vi "DM2000.vi"   [LabVIEW 2013, in "main.lvlib"]
uses:
  main.lvlib
  Controls/Enum Variables.ctl
  Controls/Enum Save Action Events.ctl
  Controls/Enum Paper Action Events.ctl
  Controls/Enum Process Data.ctl
  Controls/Enum DICOM.ctl
  Controls/Enum User Events.ctl
  New Design/Controls/Reference AE Control.ctl
  Controls/SaveDataCluster.ctl
  Controls/Combobox Filename.ctl
  <vilib>/Utility/error.llb/DialogTypeEnum.ctl
  Components/TypeDef - SHIFTER.ctl
  New Design/Menu/Top Menu.vi
  New Design/Profile/Profile.vi
  New Design/Configuration/Configuration.vi
  New Design/Configuration/Configuration_table.vi
  New Design/Acquisition/Acquisition.vi
  New Design/Data/Data.vi
  New Design/Journal/Journal.vi
  <userlib>/_MGI/Error Handling/MGI Suppress Error Code/MGI Suppress Error Code (Scalar).vi
  Acquisition/RefData(SubVI).vi
  Bluetooth/AsyncBluetoothHandler.vi
  Globals/DataPathGlobalVariable.vi
  <userlib>/_OpenG.lib/file/file.llb/File Exists - Scalar__ogtk.vi
  Globals/DataAcqRecordPathGlobal.vi
  <vilib>/Utility/file.llb/Write To Spreadsheet File (string).vi
  <userlib>/_OpenG.lib/error/error.llb/Filter Error Codes (Array)__ogtk.vi
  <vilib>/Utility/file.llb/Read From Spreadsheet File (DBL).vi
  <vilib>/Utility/file.llb/Write To Spreadsheet File (DBL).vi
  <vilib>/Utility/file.llb/Read From Spreadsheet File (string).vi
  <userlib>/_OpenG.lib/file/file.llb/Valid Path - Traditional__ogtk.vi
  <vilib>/regexp/Match Regular Expression.xnode
  Components/Dependencies.llb/TLB_Dependencies.lvlib
  Settings/Options/Options.vi
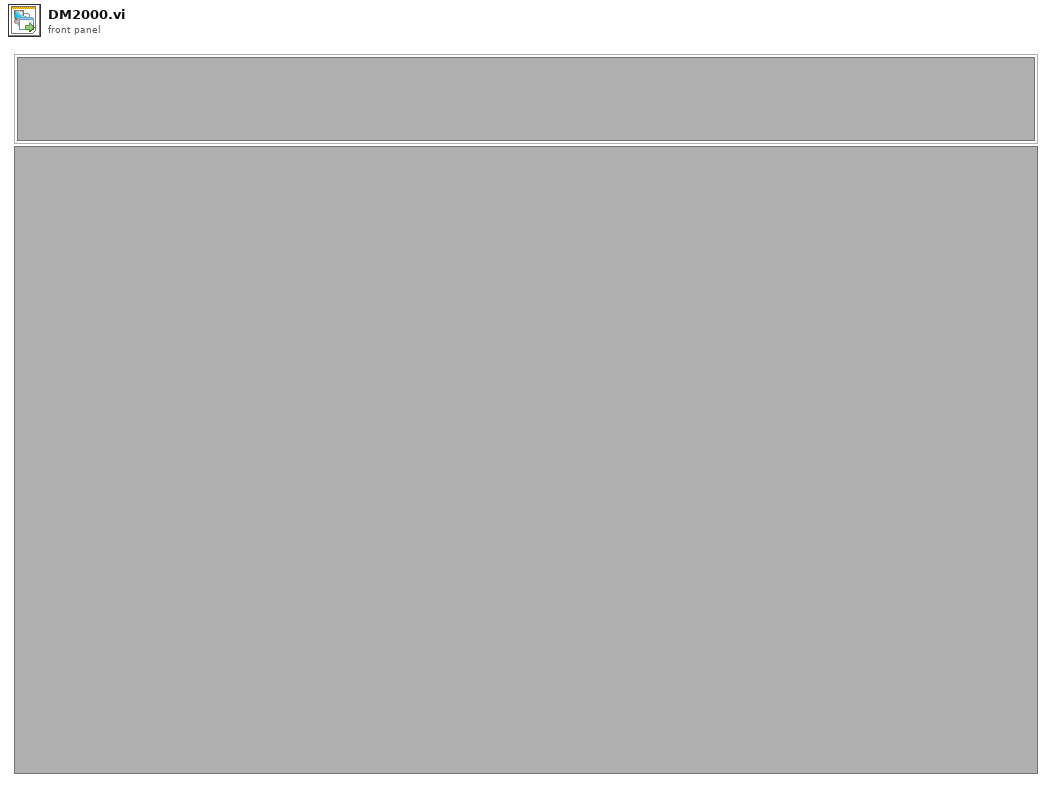
[diagram p1: front panel]
types:
  T1 = enum16{"Clear SR", "Set Display", "Set Shifter", "Initialize Events", "Init Q"}
  T2 = enum32{"Invalid", "Standard", "Closed", "Hidden", "Minimized", "Maximized"}
  T3 = typedef "main.lvlib/TypeDef - SHIFTER.ctl" = cluster{"Exit Event":T4, "Terminate Error":errorcluster, "User Parameter Controls":refnum<vi>[], "User Parameters":cluster{"Name":string, "CPR Number":string, "Measuring Type ":string, "Measuring Technique":string, "Measuring Limb":string, "Operator":string, "Doctor":string, "Comment":string, "AdditionalInfo":string, "RightArm":string[][], "LeftArm":string[][], "PalpationRight":string, "PalpationLeft":string, "Puls":dbl, "Temp One":dbl, "Temp Two":dbl, "ActivityBox":bool}, "System Parameters":cluster{"Paper Running?":bool, "GraphSelection":bool, "Date":string, "Active Page":string}, "Data Acquisition":cluster{"Acquisition":bool, "DAQmx Task":refnum<k21>, "DAQmx Error":errorcluster, "Record number":dbl, "RecordPath":path, "AcqDataRef":refnum<vi>, "Duration":timestamp, "Queue":refnum<queue>, "Control?":bool, "RelativeRecordPath":path}, "Reference signal":cluster{"DAQmx  Task ":refnum<k21>, "Monitor":bool, "Events":dbl, "Time":timestamp, "NullEvents":dbl, "RefDataRef":refnum<vi>, "Queue":refnum<queue>}, "Data Process":cluster{"SubpanelRef":refnum<vi>, "ActiveItemTag":string, "Queue":refnum<queue>}, "System Parameter Controls":refnum<vi>[], "Database":cluster{"PatientdataRef":refnum<file>, "PatientdataPath":path, "Blue Pressure":dbl, "Red Pressure":dbl, "ActiveItemTag":string, "Height Adjustment":dbl, "BluePositionArray":dbl[][], "RedPositionArray":dbl[][], "JournalPath":path}, "MWL":cluster{"PatientID":string, "Name":string, "DICOM Info":path, "DICOM Variables":string[], "Worklist":string[][]}, "Control":cluster{"Queue":refnum<queue>, "SignalCluster":cluster{"Pump":bool, "Finger":bool, "Ankle":bool, "Fast Def":bool, "Slow Def":bool, "Init Cal":bool, "Table Pres":bool, "Table":bool}}, "PageMenu":cluster{"VI Reference":refnum<vi>, "Queue":refnum<queue>}, "Profile":cluster{"VI Reference":refnum<vi>, "Queue":refnum<queue>}, "Configuration":cluster{"VI Reference":refnum<vi>, "Queue":refnum<queue>}, "Acquisition":cluster{"VI Reference":refnum<vi>, "Queue":refnum<queue>}, "Data":cluster{"VI Reference":refnum<vi>, "Queue":refnum<queue>}, "Journal":cluster{"VI Reference":refnum<vi>, "Queue":refnum<queue>}, "cRef":T5, "Bluetooth":cluster{"Queue":refnum<queue>, "VI Reference":refnum<vi>}}
  T4 = typedef "main.lvlib/TLB_Dependencies.lvlib/Exit Event Ref.ctl" = refnum<user-event>
  T5 = typedef "main.lvlib/Reference Cluster.ctl" = cluster{"Menu":cluster{"References":cluster{"Stop Acq":refnum<vi>, "MenuExit":refnum<vi>, "MenuStartADC":refnum<vi>, "PersonalInfoString":refnum<vi>, "Profile":refnum<vi>, "Configuration":refnum<vi>, "Acquisition":refnum<vi>, "Data":refnum<vi>, "Journal":refnum<vi>}}, "Profile":cluster{"References":cluster{"Search Patient ID":refnum<vi>, "Name":refnum<vi>, "CommentStr":refnum<vi>, "Listbox Patient ID":refnum<vi>, "ListboxDoctor":refnum<vi>, "ListboxOperator":refnum<vi>, "HospitalName":refnum<vi>, "HospitalDepartment":refnum<vi>, "HospitalAddress":refnum<vi>, "EditHospInfo":refnum<vi>, "Add Patient ID Btn":refnum<vi>, "Query Worklist":refnum<vi>}}, "Configuration":cluster{"References":cluster{"ListboxMeasurementArea":refnum<vi>, "ListboxMeasurementTechnique":refnum<vi>, "ListboxMeasurementMeth":refnum<vi>, "ListboxRightSegmentNr":refnum<vi>, "ListboxLeftSegmentNr":refnum<vi>, "HeightAdjustmentInt":refnum<vi>, "PalpationRight":refnum<vi>, "PalpationLeft":refnum<vi>, "ActivityBox":refnum<vi>}, "New method":cluster{"AddNewMeasurementBtn":refnum<vi>, "Left Time Table":refnum<vi>, "Right Time Table":refnum<vi>}, "Old method":cluster{"LeftArmPressureTable":refnum<vi>, "RightArmPressureTable":refnum<vi>, "SaveArmPressureBtn":refnum<vi>, "Puls":refnum<vi>, "TempTwo":refnum<vi>, "TempOne":refnum<vi>}, "Method":string}, "Acquisition":cluster{"References":cluster{"SegmentAcqString":refnum<vi>, "RingActGraph":refnum<vi>}}, "Data":cluster{"References":cluster{"cmString":refnum<vi>, "AdjustedHeight":refnum<vi>, "Menu":refnum<vi>, "Tangent On/Off":refnum<vi>, "FilterControl":refnum<vi>}}, "Journal":cluster{"References":cluster{"ReportSelection":refnum<vi>, "Data":refnum<vi>, "GenerateReport":refnum<vi>, "Menu":refnum<vi>, "Send To PACS":refnum<vi>}}}
  T6 = typedef "main.lvlib/TLB_Dependencies.lvlib/amc_Message Queue.ctl" = refnum<queue>
  T7 = typedef "main.lvlib/Enum Variables.ctl" = enum16{"SetAcqFilter", "GetAcqFilter", "Set Filter", "Get Filter", "Set Height", "Get Height", "Set Recorded Height", "Get Recorded Height", "Set Blue Pressure", "Get Blue Pressure", "Set Red Pressure", "Get Red Pressure", "Init", "Reset Pressure", "Set Red Cursors", "Get Red Cursors", "Set Blue Cursors", "Get Blue Cursors", "Set Language", "Get Language", "Set Active Graphs", "Get ActiveGraphs", "Set Method", "Get Method", "Set Encryption", "Get Encryption", "Set ExcelVersion", "Get ExcelVersion", "Set DICOM Avail", "Get DICOM Avail", "Set DICOM Encode", "Get DICOM Encode", "Set JournalExport", "Get JournalExport", "Set Sequence", "Get Sequence", "Set DAQ Connected", "Get DAQ Connected", "Set Current Graph", "Get Current Graph", "Set General Settings", "Get Hyphenation", "Set Arm Calc Method", "Get Arm Calc Method", "Set Dicom Tags", "Get Dicom Tags", "Set BT Serial", "Get BT Serial", "Set BT Accepted Serials", "Get BT Accepted Serials", "Get BT License", "Set BT License"}
  T8 = typedef "main.lvlib/Enum Save Action Events.ctl" = enum16{"LoadReportPath", "SaveReportPath", "Load Graph Path", "Save Graph Path", "LoadDataPath", "SaveDataPath", "Load Template Path", "Save Template Path", "Load PressureFactor", "Save PressureFactor", "Init", "Load Listbox", "Save Listbox", "LoadHospInfo", "SaveHospInfo", "Load DICOM Activation", "Save DICOM Activation", "LoadDICOMInfoWL", "SaveDICOMInfoWL", "LoadDICOMInfoPACS", "SaveDICOMInfoPACS", "Load ArmCalcMethod", "Save ArmCalcMethod", "LoadItemTags", "SaveItemTags", "LoadDICOMEncoding", "SaveDICOMEncoding", "LoadJournalType", "SaveJournalType", "LoadAcqFilterType", "SaveAcqFilterType", "Load Sequence", "Save Sequence", "Load Acquisition Mode", "Save Acquisition Mode", "Load General Settings", "Save General Settings", "Load Language", "Save Language", "Load Dicom Tags", "Save Dicom Tags", "Load BT Serial", "Save BT Serial", "Load BT License", "Save BT License"}
  T9 = typedef "LVPoint32TypeDef.ctl" = cluster{"Horizontal":i32, "Vertical":i32}
  T10 = typedef "LVRowAndColumnTypeDef.ctl" = cluster{"Row":i32, "Column":i32}
  T11 = typedef "eventvkey.ctl" = enum16{"ASCII", "Enter", "Return", "Shift", "Ctrl", "Alt", "Cmd", "Opt", "Caps", "NumLock", "Clear", "Break", "Up", "Down", "Left", "Right", "Insert", "Delete", "Home", "End", "PageUp", "PageDown", "Escape", "Help", "Pause", "ScrollLock", "F1", "F2", "F3", "F4", "F5", "F6", "F7", "F8", "F9", "F10", "F11", "F12", "F13", "F14", "F15", "F16", "F17", "F18", "F19", "F20", "F21", "F22", "F23", "F24", "Play", "VolumeUp", "VolumeDown", "Mute", "Two Byte Char"}
  T12 = typedef "main.lvlib/Enum Paper Action Events.ctl" = enum16{"Paper State", "Init"}
  T13 = typedef "main.lvlib/Enum Process Data.ctl" = enum16{"Init", "Set Cursor Mode", "Set Data Path", "Get All"}
  T14 = typedef "main.lvlib/Enum DICOM.ctl" = enum16{"Set DICOM itemTags", "Set Dicom Encoding", "Set DICOM Attributes"}
  T15 = typedef "main.lvlib/Reference AE Control.ctl" = enum16{"Initialize", "Set Menu", "Set Profile", "Set Configuration", "Set Configuration_old", "Set Configuration_new", "Set Configuration Method", "Set Acquisition", "Set Data", "Set Journal", "Get"}
  T16 = typedef "main.lvlib/Enum User Events.ctl" = enum16{"User Event", "Init"}
  T17 = cluster{"License":string, "Accepted Serials":string[]}
  T18 = typedef "main.lvlib/SaveDataCluster.ctl" = cluster{"HospInfo":cluster{"Name":string, "Address":string, "Department":string}, "Pressure":cluster{"Pressure":dbl}, "DataPath":cluster{"DataPath":path}, "ReportPath":cluster{"Path":path, "Name":string}, "DICOM Info WL":cluster{"port":i32, "AEtitle":string, "host":string, "remoteAE":string}, "DICOM Info PACS":cluster{"port":i32, "AEtitle":string, "host":string, "remoteAE":string}, "ArmCalcMethod":dbl, "itemTags":string[], "DicomEncoding":u16, "JournalType":u16, "General Settings":cluster{"Hyphenation":bool, "Language":u16, "CellStr1":string, "CellStr2":string}, "Dicom Tags":string[][], "BT Serial":cluster{"Serial Number":string, "Side":string, "Ignore?":bool}[], "BT License":cluster{"License":string, "Accepted Serials":string[]}}
  T19 = typedef "main.lvlib/Combobox Filename.ctl" = string
  T20 = enum16{"leave excel open after last close", "close only if opened by LabVIEW", "close excel after last close"}
  T21 = cluster{"sys":dbl, "dia":dbl, "puls":dbl, "date":string, "time":string, "code":string, "serial":string, "temp":dbl, "activity":string}
  T22 = cluster{"name":string, "department":string, "address":string}
  T23 = cluster{"id":string, "name":string, "operator":string, "doctor":string, "comment":string}
  T24 = typedef "DialogTypeEnum.ctl" = enum16{"no dialog", "OK message", "continue or stop message", "auto error handling dialog", "OK message + warnings", "continue/stop + warnings"}
  T25 = cluster{"port":i32, "AEtitle":string, "host":string, "remoteAE":string}
  T26 = cluster{"Search Patient ID":refnum<vi>, "Name":refnum<vi>, "CommentStr":refnum<vi>, "Listbox Patient ID":refnum<vi>, "ListboxDoctor":refnum<vi>, "ListboxOperator":refnum<vi>, "HospitalName":refnum<vi>, "HospitalDepartment":refnum<vi>, "HospitalAddress":refnum<vi>, "EditHospInfo":refnum<vi>, "Add Patient ID Btn":refnum<vi>, "Query Worklist":refnum<vi>}
  T27 = cluster{"Name":refnum<vi>, "ListboxOperator":refnum<vi>, "ListboxDoctor":refnum<vi>, "CommentStr":refnum<vi>, "Name":string, "Operator":string, "Doctor":string, "Comment":string}
  T28 = cluster{"Hospital Name 2":string, "Hospital Address 2":string, "Department 2":string}
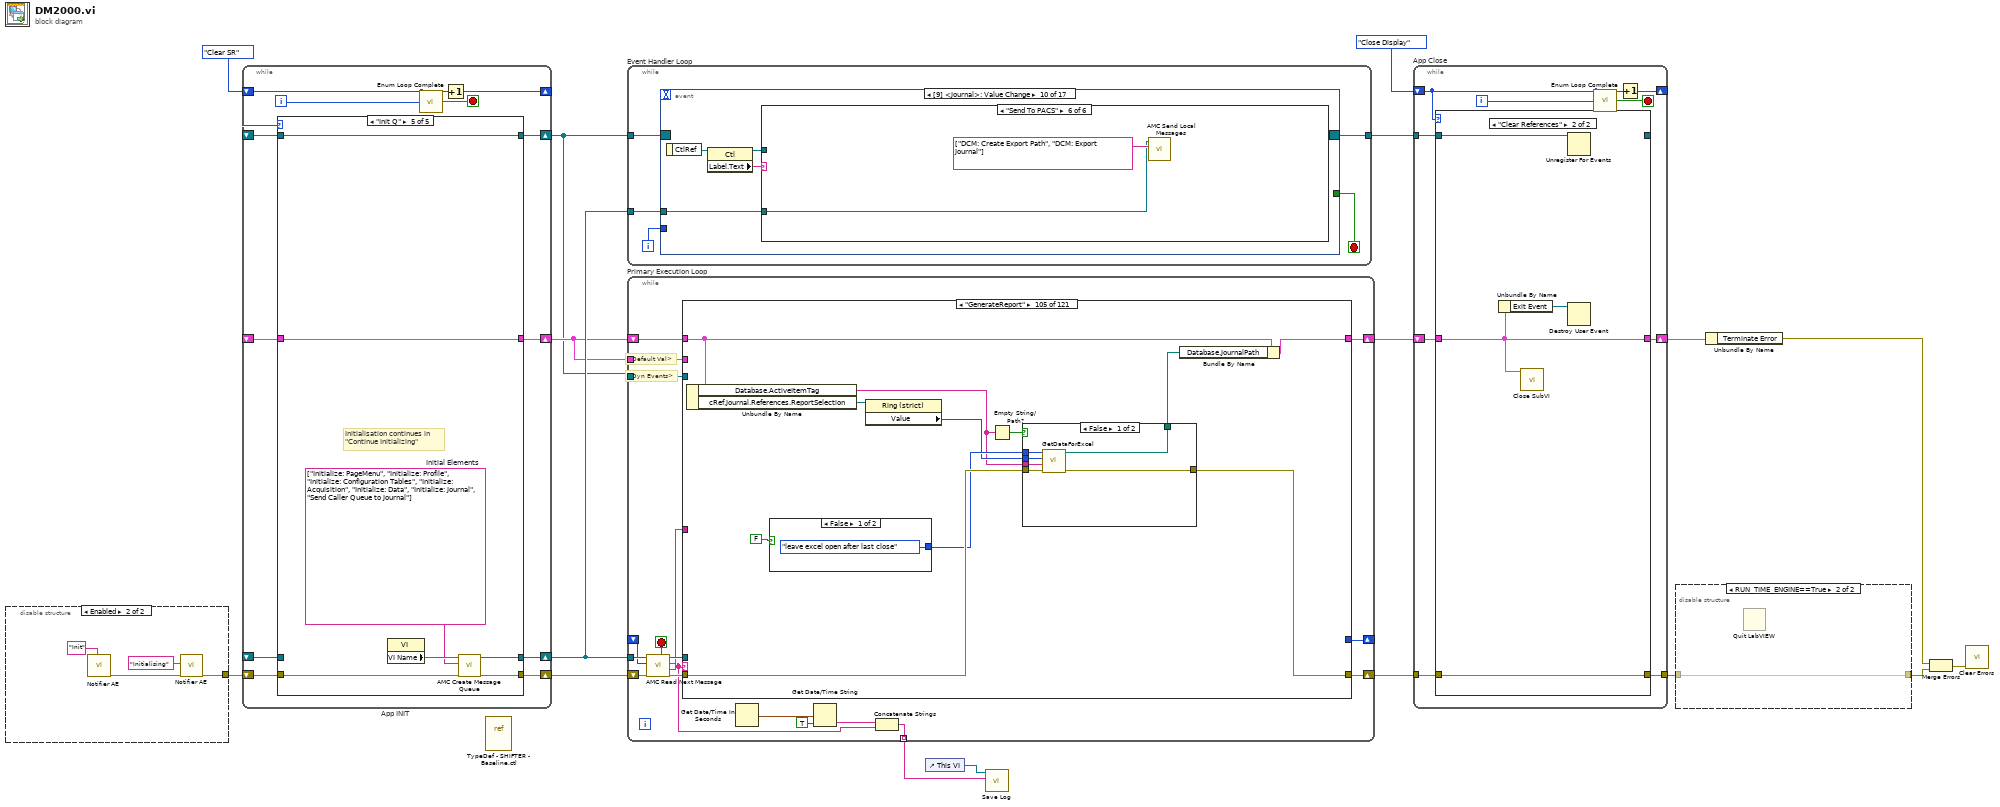
[diagram p0: block diagram]
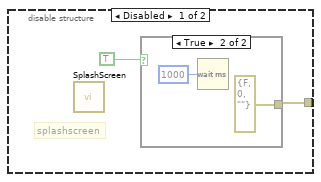
[diagram p2: hidden frame]
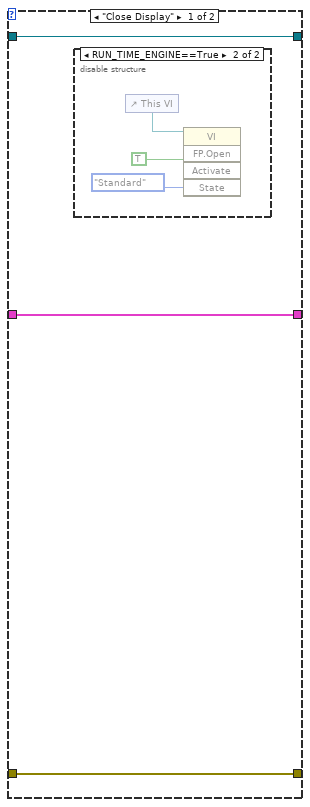
[diagram p5: hidden frame]
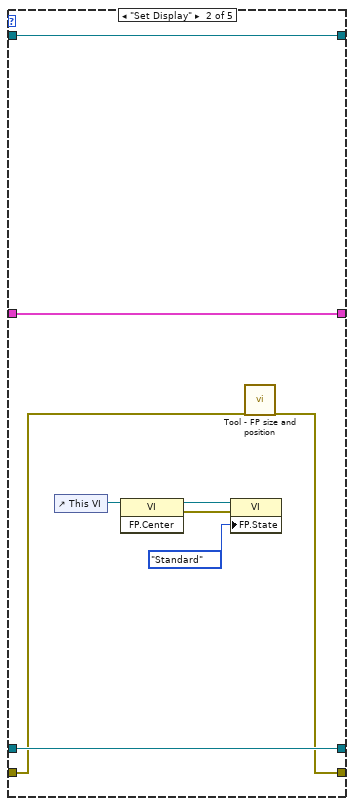
[diagram p8: hidden frame]
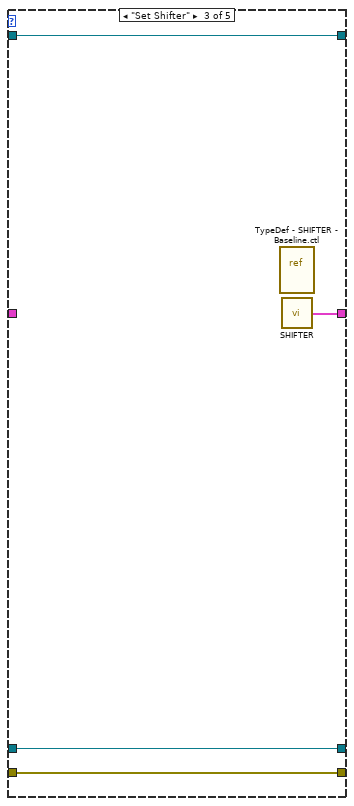
[diagram p9: hidden frame]
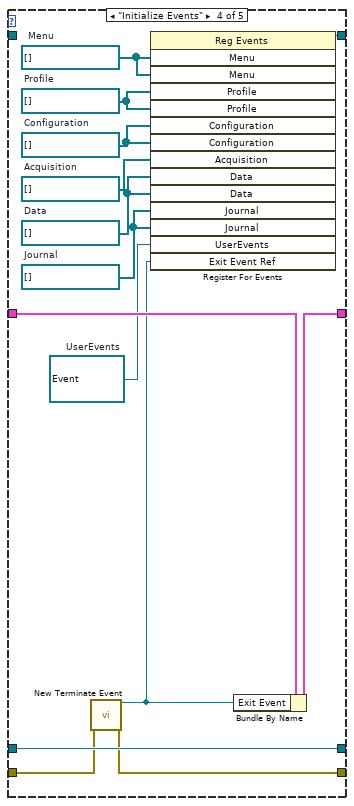
[diagram p10: hidden frame]
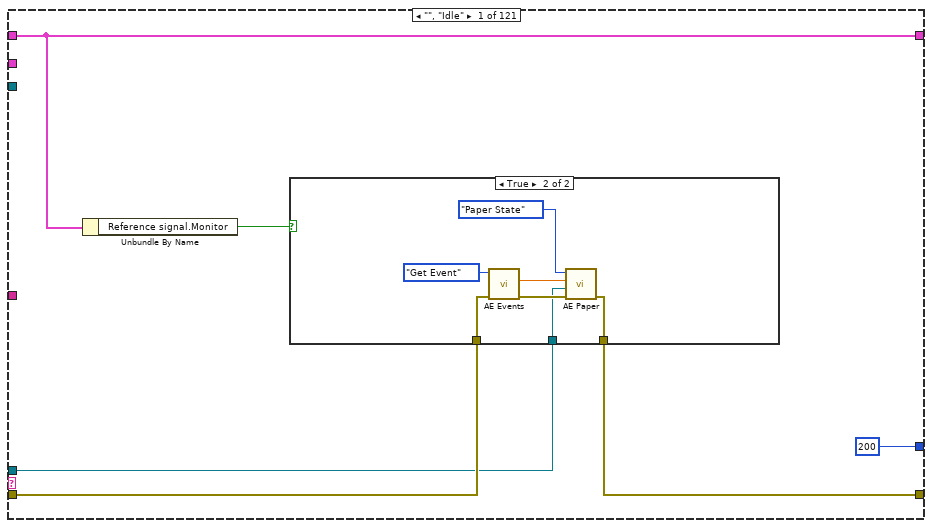
[diagram p11: hidden frame]
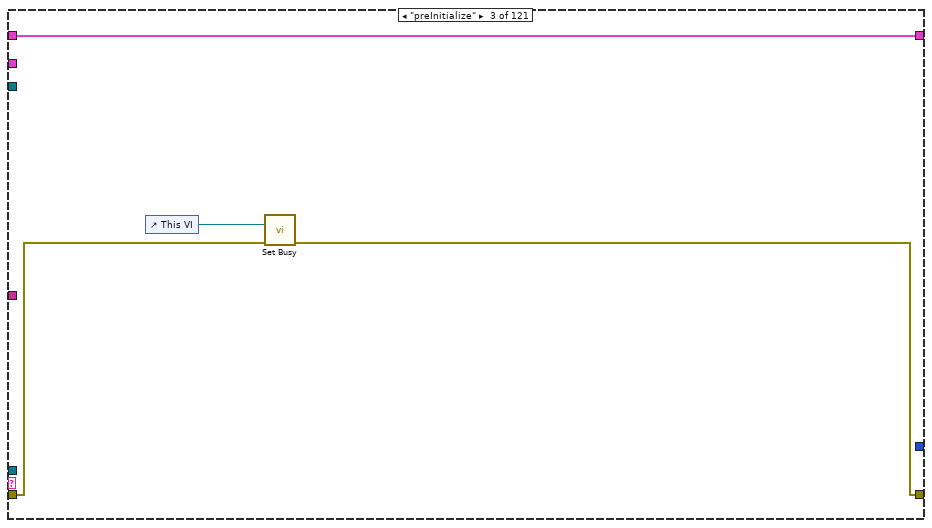
[diagram p14: hidden frame]
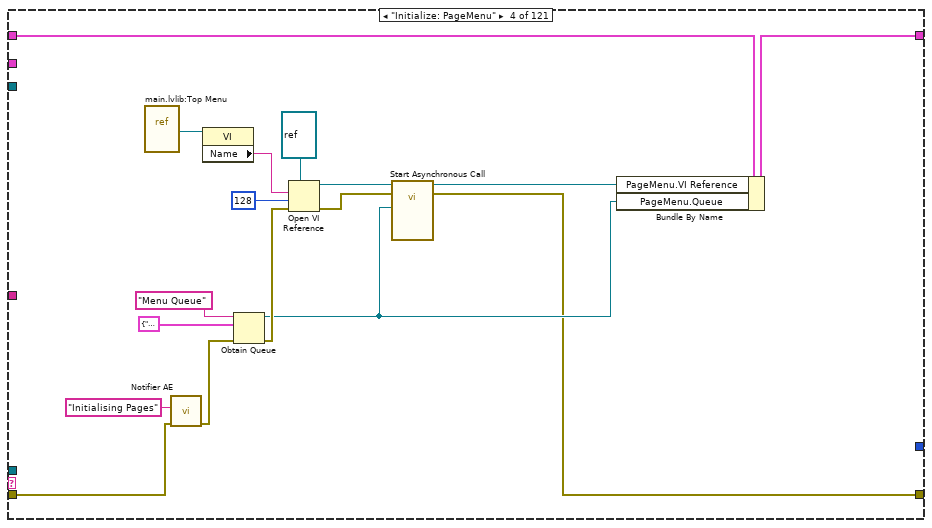
[diagram p15: hidden frame]
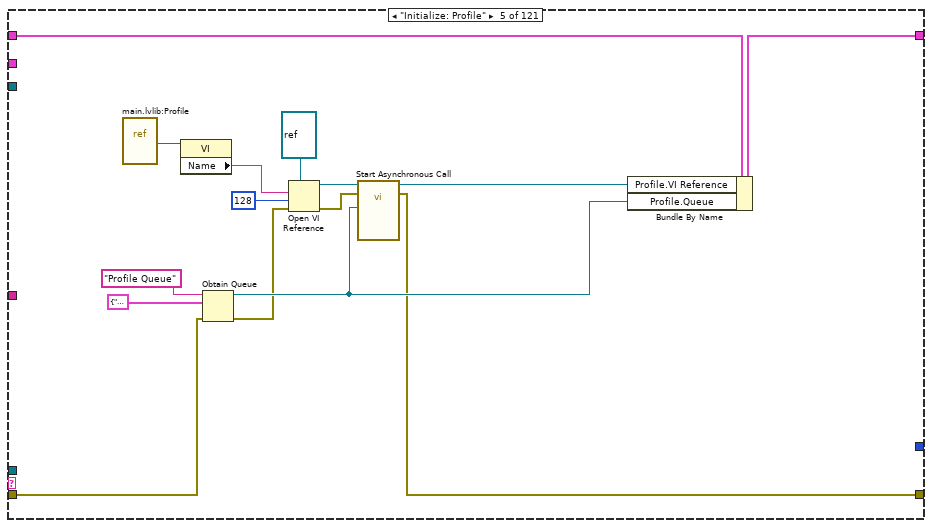
[diagram p16: hidden frame]
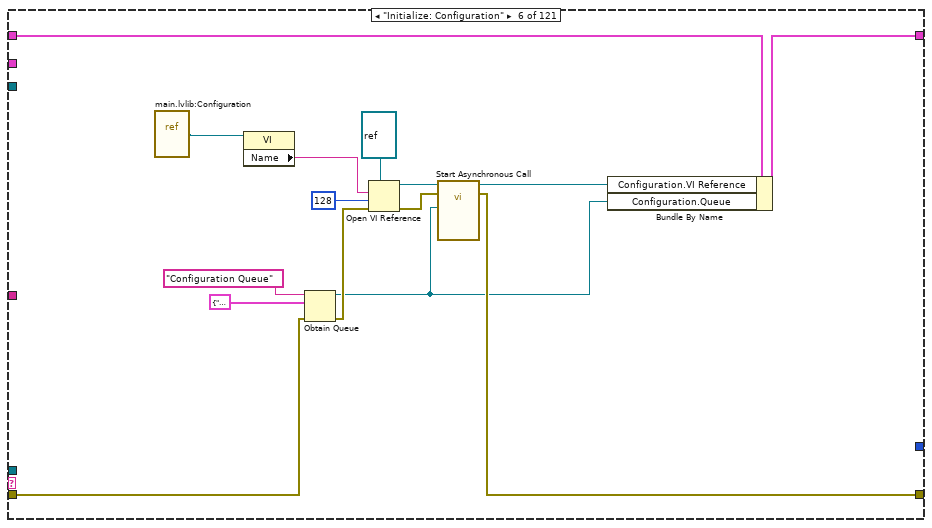
[diagram p17: hidden frame]
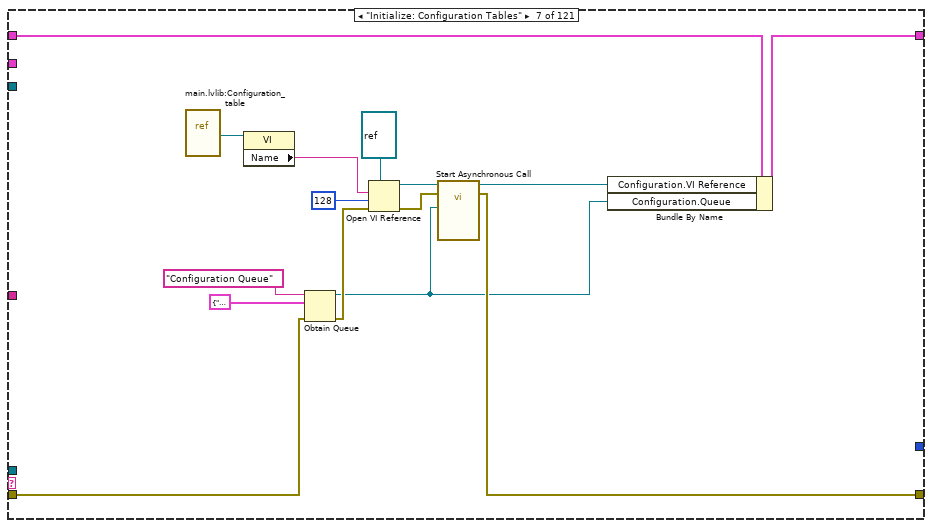
[diagram p18: hidden frame]
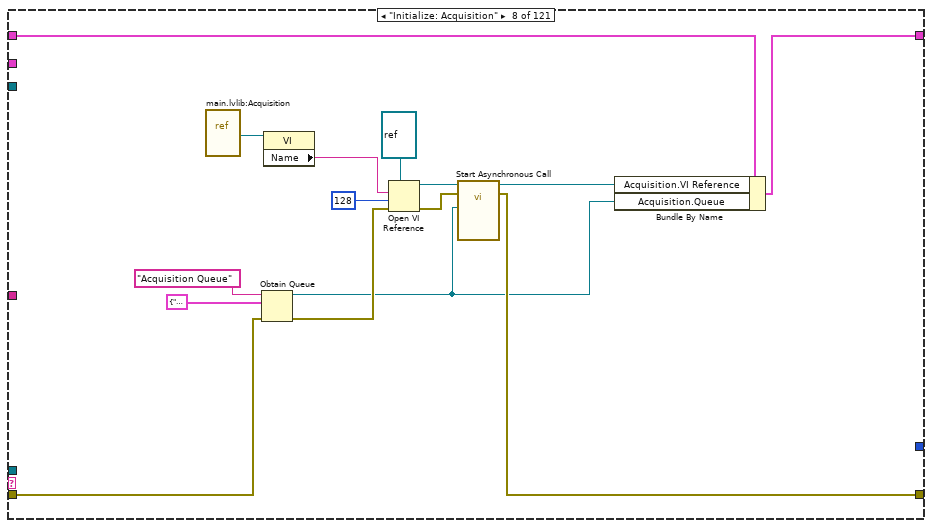
[diagram p19: hidden frame]
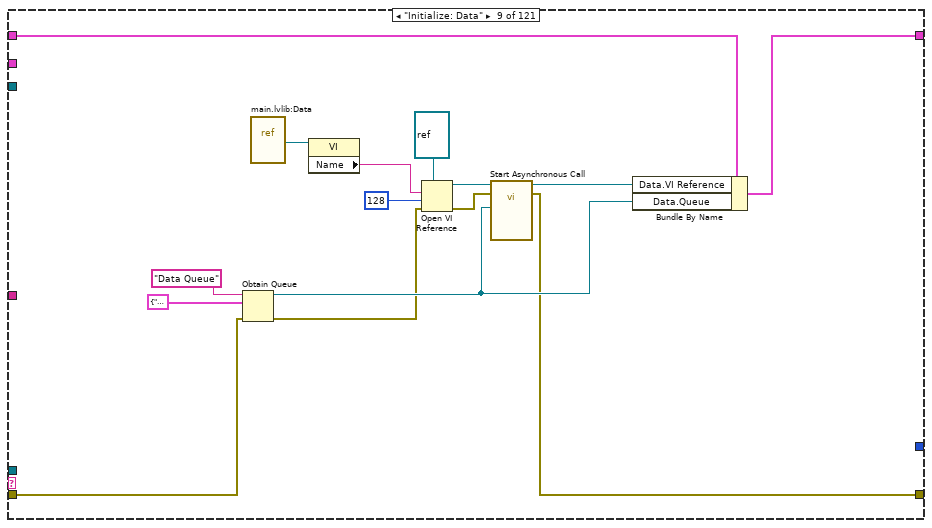
[diagram p20: hidden frame]
diagram:
  n1 = disable-structure shown="Enabled" {
    disable-tunnel: [w18 w23] -> w3
    frame Disabled {
      # "splashscreen"
      n2 = call "SplashScreen.vi"() -> ()  [unwired: 11 in, 1 out]
      n3 = case shown="True" TRUE {
        tunnel: [_ errorcluster {"status"=FALSE, "code"=0, "source"=""} ("error out")] -> w18
        frame False {
        }
        frame True {
          n4 = Wait (ms)(milliseconds to wait=u32 1000) -> ()  [unwired: 1 out]
        }
      }
    }
    frame Enabled {
      n5 = call "Notifier AE.vi"("Cmd"="Init") -> ("error out"=w24:errorcluster)  [unwired: 10 in]
      n6 = call "Notifier AE.vi"("error in (no error)"=w24, "String"="Initialising") -> ("error out"=w23:errorcluster)  [unwired: 9 in]
    }
  }
  n7 = while "App INIT" {
    shift-right: [w31] -> _
    shift-left: T1."Clear SR" -> [w26]
    shift-right: [w37] -> w7
    shift-left: _ -> [w30]
    shift-right: [w34] -> w12
    shift-left: w3 -> [w29]
    shift-right: [w36] -> w5
    shift-left: _ -> [w28]
    shift-right: [w35] -> w6
    shift-left: _ -> [w27]
    i -> [w32]
    stop <- w33 stop-if-true
    n8 = case shown="\"Init Q\"" w26 {
      tunnel: [_ w44 w49 w64 w68] -> w37
      tunnel: [_ w43 w48 w59 w66] -> w34
      tunnel: [_ w46 w50 w62 w70] -> w35
      tunnel: [_ w45 w47 w61 w71] -> w36
      tunnel: w30 -> [_ w44 w49 w64 _]
      tunnel: w29 -> [_ w42 w48 w60 w67]
      tunnel: w28 -> [_ w45 w47 _ w71]
      tunnel: w27 -> [_ w46 _ w63 w70]
      frame "Clear SR" {
      }
      frame "Set Display" {
        n9 = control-ref of="This VI"() -> (w40:refnum<vi>)
        n10 = invoke class="VI" method="FP.Center"(reference=w40) -> (reference out=w39:refnum<vi>, error out=w38:errorcluster)  [unwired: 2 in, 1 out]
        n11 = property class="VI"(reference=w39, error in=w38, "FP.State"=T2."Standard" ("Front Panel Window:State")) -> ()  [unwired: 2 out]
        n12 = call "Tool - FP size and position.vi"("error in (no error)"=w42) -> ("error out"=w43:errorcluster)  [unwired: 7 in, 11 out]
      }
      frame "Set Shifter" {
        n13 = vi-ref "TypeDef - SHIFTER - Baseline.ctl"() -> ()  [unwired: 1 out]
        n14 = call "SHIFTER.vi"() -> ("SHIFTER DATA"=w50:T3)  [unwired: 15 out]
      }
      frame "Initialize Events" {
        w53 = refnum<vi>[] []  # Journal
        w54 = refnum<vi>[] []  # Data
        w55 = refnum<vi>[] []  # Acquisition
        w56 = refnum<vi>[] []  # Configuration
        w52 = refnum<user-event> refnum  # UserEvents
        w57 = refnum<vi>[] []  # Profile
        w58 = refnum<vi>[] []  # Menu
        n15 = call "New Terminate Event.vi"("error in (no error)"=w60) -> ("Exit Event Ref"=w51:T4, "error out"=w59:errorcluster)  [unwired: 13 in]
        n16 = register-events(w58, w58, w57, w57, w56, w56, w55, w54, w54, w53, w53, w52, w51) -> (reference out=w61:refnum<event-registration>)  [unwired: 2 in, 1 out]
        n17 = Bundle By Name(cluster=w63, "Exit Event"=w51) -> (w62:T3)
      }
      frame "Init Q" {
        w65 = string[] ["Initialize: PageMenu", "Initialize: Profile", "Initialize: Configuration Tables", "Initialize: Acquisition", "Initialize: Data", "Initialize: Journal", "Send Caller Queue to Journal"]  # Initial Elements
        # "Initialisation continues in \n\"Continue Initializing\""
        n18 = property class="VI"() -> ("VI Name"=w69:string)  [unwired: 2 in, 2 out]
        n19 = call "AMC Create Message Queue.vi"("error in (no error)"=w67, "Initial Message Names"=w65, "Message Queue Name"=w69) -> ("error out"=w66:errorcluster, "Message Queue out"=w68:T6)  [unwired: 7 in]
      }
    }
    n20 = call "Enum Loop Complete.vi"("Current State Enum"=w26, "Itteration"=w32) -> ("Loop Complete?"=w33:bool)  [unwired: 13 out]
    n21 = Increment(x=w26) -> (x+1=w31:T1)
  }
  n22 = vi-ref "TypeDef - SHIFTER - Baseline.ctl"() -> ()  [unwired: 1 out]
  n23 = while "Event Handler Loop" {
    tunnel: w5 -> [w75]
    tunnel: w7 -> [w74]
    tunnel: [w73] -> w15
    i -> [w72]
    stop <- w76 stop-if-true
    n24 = event shown="[9] <Journal>: Value Change" {
      selector: w75 -> [_ _ _ _ _ _ _ _ _ _ _ _ _ _ _ _ _]
      dyn-events: [_ _ _ _ _ _ _ _ _ _ _ _ _ _ _ _ _] -> w73
      timeout: _ -> [_ _ _ _ _ _ _ _ _ _ _ _ _ _ _ _ _]
      tunnel: [_ _ _ _ _ _ _ _ _ _ _ _ TRUE ("NewVal") TRUE ("NewVal") _ w292 _] -> w76
      tunnel: w74 -> [w80 _ w106 w124 w155 _ _ w179 w191 w207 w219 w236 w269 w270 w274 w293 _]
      tunnel: w72 -> [_ _ _ _ _ _ _ _ _ _ _ _ _ _ _ _ _]
      event Value Change {
        n25 = event-data() -> ("CtlRef"=w82:refnum<vi>)  [unwired: 1 out]
        n26 = property class="Ctl"(reference=w82) -> (reference out=w77:refnum<vi>, "Label.Text"=w81:string)  [unwired: 1 in, 1 out]
        n27 = call "AMC Send Local Message.vi"("Message Name"="Cache User Parameters", "Message Queue in"=w80) -> ("Message Queue out"=w79:T6)  [unwired: 8 in, 1 out]
        n28 = case shown="\"Data\"" w81 {
          tunnel: w79 -> [_ w84 w85 w87 w89 w91 w97 w102 w105]
          tunnel: w77 -> [_ _ _ _ _ _ w96 _ _]
          frame "", Default {
          }
          frame "Profile" {
            n29 = call "AMC Send Local Messages.vi"("Message Names"=string[] ["Subpanel: Load Profile"], "Message Queue in"=w84) -> ()  [unwired: 8 in, 2 out]
          }
          frame "Configuration" {
            n30 = call "AMC Send Local Messages.vi"("Message Names"=string[] ["Subpanel: Load Configuration"], "Message Queue in"=w85) -> ()  [unwired: 8 in, 2 out]
          }
          frame "Acquisition" {
            n31 = call "AMC Send Local Messages.vi"("Message Names"=string[] ["Update Display", "Subpanel: Load Acquisition", "Send Segment to Acquisition"], "Message Queue in"=w87) -> ()  [unwired: 8 in, 2 out]
          }
          frame "Data" {
            n32 = call "AMC Send Local Messages.vi"("Message Names"=string[] ["Subpanel: Load Data"], "Message Queue in"=w89) -> ()  [unwired: 8 in, 2 out]
          }
          frame "Journal" {
            n33 = call "AMC Send Local Messages.vi"("Message Names"=string[] ["Subpanel: Load Journal", "FillDataTable"], "Message Queue in"=w91) -> ()  [unwired: 8 in, 2 out]
          }
          frame "MenuStartADC" {
            n34 = property class="Ctl"(reference=w96) -> ("Value"=w95:variant)  [unwired: 1 in, 2 out]
            n35 = Variant To Data(type=TRUE, Variant=w95) -> (data=w93:bool)  [unwired: 1 in, 1 out]
            n36 = case shown="True" w93 {
              tunnel: w97 -> [w98 w100]
              frame False {
                n37 = call "AMC Send Local Messages.vi"("Message Names"=string[] ["Stop Reference", "Update Display", "", "", ""], "Message Queue in"=w98) -> ()  [unwired: 8 in, 2 out]
              }
              frame True {
                n38 = call "AMC Send Local Messages.vi"("Message Names"=string[] ["Query DAQ Availability", "SavePatientDataOnDate"], "Message Queue in"=w100) -> ()  [unwired: 8 in, 2 out]
              }
            }
          }
          frame "Stop Acq" {
            n39 = call "AMC Send Local Messages.vi"("Message Names"=string[] ["Stop Reference", "Update Display", "", "", ""], "Message Queue in"=w102) -> ()  [unwired: 8 in, 2 out]
          }
          frame "MenuExit" {
            n40 = call "AMC Send Local Message.vi"("Message Name"="Exit", "Message Queue in"=w105) -> ()  [unwired: 8 in, 2 out]
          }
        }
      }
      event Shortcut Menu Selection (User) {
        n41 = event-data() -> ()  [unwired: 6 out]
      }
      event Value Change {
        n42 = event-data() -> ("CtlRef"=w108:refnum<vi>)  [unwired: 1 out]
        n43 = property class="Ctl"(reference=w108) -> ("Label.Text"=w107:string)  [unwired: 1 in, 2 out]
        n44 = case shown="\"CommentStr\", \"ListboxDoctor\", \"ListboxOperator\", \"Name\"" w107 {
          tunnel: w106 -> [_ w109 w111 w114 w115 w117 w119]
          frame "", Default {
          }
          frame "Search Patient ID" {
            n45 = call "AMC Send Local Message.vi"("Message Name"="FindCprNumber", "Message Queue in"=w109) -> ()  [unwired: 8 in, 2 out]
          }
          frame "CommentStr", "ListboxDoctor", "ListboxOperator", "Name" {
            n46 = call "AMC Send Local Messages.vi"("Message Names"=string[] ["Cache User Parameters", "SavePatientData", "Update Display", "DCM: Update Variables"], "Message Queue in"=w111) -> ()  [unwired: 8 in, 2 out]
          }
          frame "Listbox Patient ID" {
            n47 = call "AMC Send Local Messages.vi"("Message Names"=string[] ["ResetToDefault", "LoadNameCpr", "Cache User Parameters", "SelectCpr", "DCM: Load DICOM Info", "DCM: Update Variables", "Load Armpressure"], "Message Queue in"=w114) -> ()  [unwired: 8 in, 2 out]
          }
          frame "EditHospInfo" {
            n48 = call "AMC Send Local Message.vi"("Message Name"="EditHospInfo", "Message Queue in"=w115) -> ()  [unwired: 8 in, 2 out]
          }
          frame "Add Patient ID Btn" {
            n49 = call "AMC Send Local Messages.vi"("Message Names"=string[] ["AddCpr", ""], "Message Queue in"=w117) -> ()  [unwired: 8 in, 2 out]
          }
          frame "Query Worklist" {
            n50 = call "AMC Send Local Messages.vi"("Message Names"=string[] ["MWL: QueryWorklist", "MWL: PatientID", "ResetToDefault", "LoadNameCpr", "Cache User Parameters", "MWL: Update Data", "SelectCpr"], "Message Queue in"=w119) -> ()  [unwired: 8 in, 2 out]
          }
        }
      }
      event Shortcut Menu Selection (User) {
        n51 = event-data() -> ("CtlRef"=w123:refnum<vi>, "ItemTag"=w122:string, "Coords"=w121:T9)  [unwired: 3 out]
        n52 = case shown="\"Add New\"" w122 {
          tunnel: w124 -> [_ w129 w145 w152]
          tunnel: w123 -> [_ w128 w144 w151]
          tunnel: w121 -> [_ w125 w141 _]
          frame "False", Default {
          }
          frame "DeleteID" {
            w127 = refnum<vi> refnum  # ListBox
            n53 = To More Specific Class(target class=w127, reference=w128) -> (specific class reference=w126:refnum<vi>)  [unwired: 1 in, 1 out]
            n54 = invoke class="LstBox" method="Point To Row"(reference=w126, "Point"=w125) -> (reference out=w133:refnum<vi>, "Row"=w131:i32)  [unwired: 5 in, 5 out]
            n55 = property class="LstBox"(reference=w133) -> ("Item Names"=w132:string[])  [unwired: 1 in, 2 out]
            n56 = Index Array(array=w132, index=w131) -> (element=w130:string)
            n57 = call "AMC Send Local Message.vi"("Message Value"=w130, "Message Name"="RemoveCpr", "Message Queue in"=w129) -> ()  [unwired: 7 in, 2 out]
          }
          frame "Delete" {
            w143 = refnum<vi> refnum  # ListBox
            n58 = To More Specific Class(target class=w143, reference=w144) -> (specific class reference=w142:refnum<vi>)  [unwired: 1 in, 1 out]
            n59 = invoke class="LstBox" method="Point To Row"(reference=w142, "Point"=w141) -> (reference out=w140:refnum<vi>, "Row"=w139:i32)  [unwired: 5 in, 5 out]
            n60 = property class="LstBox"(reference=w140) -> ("Label.Text"=w137:string)  [unwired: 1 in, 2 out]
            n61 = Number To Decimal String(number=w139) -> (decimal integer string=w135:string)  [unwired: 1 in]
            n62 = Concatenate Strings("Delete: ", w137) -> (w136:string)
            n63 = call "AMC Send Local Message.vi"("Message Value"=w135, "Message Name"=w136, "Message Queue in"=w145) -> ()  [unwired: 7 in, 2 out]
          }
          frame "Add New" {
            w150 = refnum<vi> refnum  # ListBox
            n64 = To More Specific Class(target class=w150, reference=w151) -> (specific class reference=w146:refnum<vi>)  [unwired: 1 in, 1 out]
            n65 = property class="LstBox"(reference=w146) -> ("Label.Text"=w148:string)  [unwired: 1 in, 2 out]
            n66 = Concatenate Strings("Add New: ", w148) -> (w147:string)
            n67 = call "AMC Send Local Message.vi"("Message Name"=w147, "Message Queue in"=w152) -> ()  [unwired: 8 in, 2 out]
          }
        }
      }
      event Value Change {
        n68 = event-data() -> ("CtlRef"=w158:refnum<vi>)  [unwired: 1 out]
        n69 = call "AMC Send Local Message.vi"("Message Name"="Cache User Parameters", "Message Queue in"=w155) -> ("Message Queue out"=w154:T6)  [unwired: 8 in, 1 out]
        n70 = property class="Ctl"(reference=w158) -> (reference out=w156:refnum<vi>, "Label.Text"=w157:string)  [unwired: 1 in, 1 out]
        n71 = case shown="\"HeightAdjustmentInt\"" w157 {
          tunnel: w154 -> [_ _ _ _ _ _ w165 _ _ _ _ _ w166 _ _]
          tunnel: w156 -> [_ _ _ w162 _ _ _ _ _ _ _ _ _ _ _]
          frame "False", Default {
          }
          frame "ListboxMeasurementArea" {
          }
          frame "ListboxMeasurementTechnique" {
          }
          frame "ListboxMeasurementMeth" {
            w161 = refnum<vi> refnum  # ListBox
            n72 = To More Specific Class(target class=w161, reference=w162) -> (specific class reference=w160:refnum<vi>)  [unwired: 1 in, 1 out]
            n73 = property class="LstBox"(reference=w160) -> ("Value"=w159:variant)  [unwired: 1 in, 2 out]
            n74 = call "AE Variables.vi"("VariantIn"=w159, "Action"=Enum_Variables."Set Method") -> ()  [unwired: 10 in, 8 out]
          }
          frame "ListboxRightSegmentNr" {
          }
          frame "ListboxLeftSegmentNr" {
          }
          frame "HeightAdjustmentInt" {
            n75 = call "AMC Send Local Message.vi"("Message Name"="Set Height", "Message Queue in"=w165) -> ()  [unwired: 8 in, 2 out]
          }
          frame "TempOne" {
          }
          frame "TempTwo" {
          }
          frame "Puls" {
          }
          frame "RightArmPressureTable" {
          }
          frame "LeftArmPressureTable" {
          }
          frame "SaveArmPressureBtn" {
            n76 = call "AMC Send Local Messages.vi"("Message Names"=string[] ["SaveArmPressure", "SavePalpationData"], "Message Queue in"=w166) -> ()  [unwired: 8 in, 2 out]
          }
          frame "PalpationRight" {
          }
          frame "PalpationLeft" {
          }
        }
      }
      event Shortcut Menu Selection (User) {
        n77 = event-data() -> ("ItemTag"=w168:string)  [unwired: 5 out]
        n78 = case shown="\"True\"" w168 {
          frame "False", Default {
          }
          frame "True" {
          }
        }
      }
      event Value Change {
        n79 = event-data() -> ("CtlRef"=w171:refnum<vi>)  [unwired: 1 out]
        n80 = property class="Ctl"(reference=w171) -> (reference out=w169:refnum<vi>, "Label.Text"=w170:string)  [unwired: 1 in, 1 out]
        n81 = case shown="\"RingActGraph\"" w170 {
          tunnel: w169 -> [_ w176]
          frame "", Default {
          }
          frame "RingActGraph" {
            w175 = refnum<vi> refnum  # Ring
            n82 = To More Specific Class(target class=w175, reference=w176) -> (specific class reference=w174:refnum<vi>, error out=w173:errorcluster)  [unwired: 1 in]
            n83 = property class="Ring"(reference=w174, error in=w173) -> ("Value"=w172:variant)  [unwired: 2 out]
            n84 = call "AE Variables.vi"("VariantIn"=w172, "Action"=Enum_Variables."Set Active Graphs") -> ()  [unwired: 10 in, 8 out]
          }
        }
      }
      event Value Change {
        n85 = event-data() -> ("CtlRef"=w181:refnum<vi>)  [unwired: 1 out]
        n86 = property class="Ctl"(reference=w181) -> (reference out=w178:refnum<vi>, "Label.Text"=w180:string)  [unwired: 1 in, 1 out]
        n87 = case shown="\"ProcessDataTreeMenu\"" w180 {
          tunnel: w179 -> [_ w182 w187 w189]
          tunnel: w178 -> [_ w184 _ _]
          frame "", Default {
          }
          frame "ProcessDataTreeMenu" {
            n88 = call "Tree Menu to String.vi"("Control in"=w184) -> ("delimited string"=w183:string)  [unwired: 10 in]
            n89 = Build Array(w183) -> (w185:string[])
            n90 = call "AMC Send Local Messages.vi"("Message Values"=w185, "Message Names"=string[] ["GetActiveItemTag", "Display Data", "Update Display"], "Message Queue in"=w182) -> ()  [unwired: 7 in, 2 out]
          }
          frame "Tangent On/Off" {
            n91 = call "AMC Send Local Message.vi"("Message Name"="Set Tangent Mode", "Message Queue in"=w187) -> ()  [unwired: 8 in, 2 out]
          }
          frame "FilterControl" {
            n92 = call "AMC Send Local Messages.vi"("Message Names"=string[] ["FilterControl", "Display Data", ""], "Message Queue in"=w189) -> ()  [unwired: 8 in, 2 out]
          }
        }
      }
      event Shortcut Menu Selection (User) {
        n93 = event-data() -> ("CtlRef"=w192:refnum<vi>, "ItemTag"=w193:string)  [unwired: 4 out]
        n94 = case shown="\"ChangeSegment\"" w193 {
          tunnel: w192 -> [_ w196 w200 w204]
          tunnel: w191 -> [_ w194 w198 w202]
          frame "", Default {
          }
          frame "DeleteTreeItem" {
            n95 = call "Tree Menu to String.vi"("Control in"=w196) -> ("delimited string"=w195:string)  [unwired: 10 in]
            n96 = call "AMC Send Local Message.vi"("Message Value"=w195, "Message Name"="DeleteTreeItem", "Message Queue in"=w194) -> ()  [unwired: 7 in, 2 out]
          }
          frame "ChangeSegment" {
            n97 = call "Tree Menu to String.vi"("Control in"=w200) -> ("delimited string"=w199:string)  [unwired: 10 in]
            n98 = call "AMC Send Local Message.vi"("Message Value"=w199, "Message Name"="ChangeSegment", "Message Queue in"=w198) -> ()  [unwired: 7 in, 2 out]
          }
          frame "ExportGraphs" {
            n99 = call "Tree Menu to String.vi"("Control in"=w204) -> ("delimited string"=w203:string)  [unwired: 10 in]
            n100 = call "AMC Send Local Message.vi"("Message Value"=w203, "Message Name"="ExportGraphs", "Message Queue in"=w202) -> ()  [unwired: 7 in, 2 out]
          }
        }
      }
      event Value Change {
        n101 = event-data() -> ("CtlRef"=w209:refnum<vi>)  [unwired: 1 out]
        n102 = property class="Ctl"(reference=w209) -> (reference out=w206:refnum<vi>, "Label.Text"=w208:string)  [unwired: 1 in, 1 out]
        n103 = case shown="\"Send To PACS\"" w208 {
          tunnel: w207 -> [_ _ _ w210 w215 w217]
          tunnel: w206 -> [_ _ _ _ w214 _]
          frame "", Default {
          }
          frame "ReportSelection" {
          }
          frame "Data Listbox" {
          }
          frame "GenerateReport" {
            n104 = call "AMC Send Local Message.vi"("Message Name"="GenerateReport", "Message Queue in"=w210) -> ()  [unwired: 8 in, 2 out]
          }
          frame "Data Menu" {
            # "Need to convert to array because\nmultiple messages"
            n105 = call "Tree Menu to String.vi"("Control in"=w214) -> ("delimited string"=w213:string)  [unwired: 10 in]
            n106 = Build Array(w213) -> (w212:string[])
            n107 = call "AMC Send Local Messages.vi"("Message Values"=w212, "Message Names"=string[] ["FillDataTable", "DCM: Create Export Path", "DCM: Load DICOM Info", "DCM: Update Variables"], "Message Queue in"=w215) -> ()  [unwired: 7 in, 2 out]
          }
          frame "Send To PACS" {
            n108 = call "AMC Send Local Messages.vi"("Message Names"=string[] ["DCM: Create Export Path", "DCM: Export Journal"], "Message Queue in"=w217) -> ()  [unwired: 8 in, 2 out]
          }
        }
      }
      event Shortcut Menu Selection (User) {
        n109 = event-data() -> ("CtlRef"=w221:refnum<vi>, "ItemTag"=w222:string, "Coords"=w220:T9)  [unwired: 3 out]
        n110 = case shown="\"DeleteSingleMeasurement\"" w222 {
          tunnel: w221 -> [_ w224 w233]
          tunnel: w220 -> [_ _ w230]
          tunnel: w219 -> [_ w223 w228]
          frame "", Default {
          }
          frame "DeleteTreeItem" {
            n111 = call "Tree Menu to String.vi"("Control in"=w224) -> ("delimited string"=w225:string)  [unwired: 10 in]
            n112 = call "AMC Send Local Message.vi"("Message Value"=w225, "Message Name"="DeleteTreeItem", "Message Queue in"=w223) -> ()  [unwired: 7 in, 2 out]
          }
          frame "DeleteSingleMeasurement" {
            w232 = refnum<vi> refnum  # MulticolumnListbox
            n113 = To More Specific Class(target class=w232, reference=w233) -> (specific class reference=w231:refnum<vi>)  [unwired: 1 in, 1 out]
            n114 = invoke class="MCListbox" method="Point To Row Column"(reference=w231, "Point"=w230) -> ("CellPosition"=w234:T10)  [unwired: 5 in, 6 out]
            n115 = Flatten To String(anything=w234) -> (data string=w227:string)  [unwired: 3 in, 2 out]
            n116 = call "AMC Send Local Message.vi"("Message Value"=w227, "Message Name"="DeleteSingleMeasurement", "Message Queue in"=w228) -> ()  [unwired: 7 in, 2 out]
          }
        }
      }
      event User Event {
        n117 = event-data() -> ("Event"=w235:string)  [unwired: 1 out]
        n118 = case shown="\"BTelement\"" w235 {
          selector: w235 -> [_ _ _ _ _ _ _ _ _ w257 _ _ _ _]
          tunnel: w236 -> [_ w237 w243 w246 w247 w249 w251 w254 w256 w258 w260 w262 w264 w265]
          frame "", Default {
          }
          frame "DaqError" {
            n119 = One Button Dialog(message="Programmet kan ikke få kontakt til dit USB6008\ndataopsamlingskort. Undersøg venligst om dette er\ntilsluttet korrekt.", button name ("OK")="Luk") -> ()  [unwired: 1 out]
            n120 = call "AMC Send Local Messages.vi"("Message Names"=string[] ["Stop Reference", "Update Display"], "Message Queue in"=w237) -> ()  [unwired: 8 in, 2 out]
          }
          frame "tdmsError" {
            n121 = One Button Dialog(message="Data fejl", button name ("OK")="Luk") -> ()  [unwired: 1 out]
            n122 = call "AMC Send Local Messages.vi"("Message Names"=string[] ["Stop Reference", "Update Display"], "Message Queue in"=w243) -> ()  [unwired: 8 in, 2 out]
          }
          frame "SavePressure" {
            n123 = call "AMC Send Local Messages.vi"("Message Names"=string[] ["GetProcessData", "SaveProcessData"], "Message Queue in"=w246) -> ()  [unwired: 8 in, 2 out]
          }
          frame "TangentMode" {
            n124 = call "AMC Send Local Message.vi"("Message Name"="Set Tangent Mode: True", "Message Queue in"=w247) -> ()  [unwired: 8 in, 2 out]
          }
          frame "StopCalibration" {
            n125 = call "AMC Send Local Messages.vi"("Message Names"=string[] ["Calibrate Pressure: Step 3", "Monitor Reference"], "Message Queue in"=w249) -> ()  [unwired: 8 in, 2 out]
          }
          frame "Set Acquisition Mode" {
            n126 = call "AMC Send Local Messages.vi"("Message Names"=string[] ["Set Acquisition Mode"], "Message Queue in"=w251) -> ()  [unwired: 8 in, 2 out]
          }
          frame "Set DICOM Availability" {
            n127 = call "AMC Send Local Messages.vi"("Message Names"=string[] ["Load Menu", "Initialize: Dicom"], "Message Queue in"=w254) -> ()  [unwired: 8 in, 2 out]
          }
          frame "New Data Path" {
            n128 = call "AMC Send Local Messages.vi"("Message Names"=string[] ["ResetToDefault", "Load Patient Register"], "Message Queue in"=w256) -> ()  [unwired: 8 in, 2 out]
          }
          frame "Regulation Stopped" {
            n129 = call "AMC Send Local Message.vi"("Message Name"=w257, "Message Queue in"=w258) -> ()  [unwired: 8 in, 2 out]
          }
          frame "Set New Hospital Info" {
            n130 = call "AMC Send Local Message.vi"("Message Name"="Load Hospital Info", "Message Queue in"=w260) -> ()  [unwired: 8 in, 2 out]
          }
          frame "Change Language" {
            n131 = call "AMC Send Local Messages.vi"("Message Names"=string[] ["Change Language", "Load Patient Register", "Initialize: Dicom"], "Message Queue in"=w262) -> ()  [unwired: 8 in, 2 out]
          }
          frame "BTelement" {
            n132 = call "AMC Send Local Message.vi"("Message Name"="BT: Dequeue Element", "Message Queue in"=w264) -> ()  [unwired: 8 in, 2 out]
          }
          frame "SavePatientData" {
            n133 = call "AMC Send Local Message.vi"("Message Name"="SavePatientData", "Message Queue in"=w265) -> ()  [unwired: 8 in, 2 out]
          }
        }
      }
      event User Event {
        n134 = event-data() -> ()  [unwired: 2 out]
        n135 = call "AMC Send Local Messages.vi"("Message Names"=string[] ["BT: Stop", "Exit"], "Message Queue in"=w269) -> ()  [unwired: 8 in, 2 out]
      }
      event Panel Close? {
        w272 = TRUE  # Discard?
        n136 = event-data() -> ()  [unwired: 2 out]
        n137 = call "AMC Send Local Message.vi"("Message Name"="Exit", "Message Queue in"=w270) -> ()  [unwired: 8 in, 2 out]
        n138 = event-data("Discard?"=w272) -> ()  [unwired: 1 in, 1 out]
      }
      event Key Down {
        n139 = event-data() -> ("VKey"=w275:T11, "ScanCode"=w276:i16)  [unwired: 3 out]
        n140 = case shown="57" w276 {
          tunnel: w275 -> [_ _ w281 w286]
          tunnel: w274 -> [_ w278 w280 w285]
          frame 0, Default {
          }
          frame 57 {
            # "Space"
            n141 = call "AMC Send Local Message.vi"("Message Value"="Space", "Message Name"="KeyDown", "Message Queue in"=w278) -> ()  [unwired: 7 in, 2 out]
          }
          frame 77 {
            n142 = case shown="\"Right\"" w281 {
              tunnel: w280 -> [_ w283]
              frame "ASCII", Default {
              }
              frame "Right" {
                # "Rightarrow"
                n143 = call "AMC Send Local Message.vi"("Message Value"="Right", "Message Name"="KeyDown", "Message Queue in"=w283) -> ()  [unwired: 7 in, 2 out]
              }
            }
          }
          frame 75 {
            n144 = case shown="\"Left\"" w286 {
              tunnel: w285 -> [_ w288]
              frame "ASCII", Default {
              }
              frame "Left" {
                # "Leftarrow"
                n145 = call "AMC Send Local Message.vi"("Message Value"="Left", "Message Name"="KeyDown", "Message Queue in"=w288) -> ()  [unwired: 7 in, 2 out]
              }
            }
          }
        }
      }
      event Menu Selection (User) {
        n146 = event-data() -> ("MenuRef"=w290:refnum<k9>, "ItemTag"=w294:string, "ItemPath"=w291:string)  [unwired: 2 out]
        n147 = case shown="\"NewTest\"" w294 {
          tunnel: w293 -> [_ w295 w299 _ w301 _ w306 w312 _ _ w315 _ w318 w320 _ _ _ _ _ w330 _ _ _ _]
          tunnel: [_ _ TRUE _ _ _ _ _ _ _ _ _ _ _ _ _ _ _ _ _ _ _ _ _] -> w292
          tunnel: w291 -> [_ _ _ _ _ _ _ _ _ _ _ _ _ _ _ _ _ _ _ _ _ _ _ _]
          tunnel: w290 -> [_ _ _ _ _ _ _ _ _ _ _ _ _ _ _ _ _ _ _ _ _ _ _ _]
          frame Default {
          }
          frame "NewTest" {
            # "Opret ny undersøgelse"
            n148 = call "AMC Send Local Message.vi"("Message Name"="InitNewTest", "Message Queue in"=w295) -> ()  [unwired: 8 in, 2 out]
          }
          frame "ExitProgram" {
            n149 = call "AMC Send Local Messages.vi"("Message Names"=string[] ["Close SubVI", "Exit"], "Message Queue in"=w299) -> ()  [unwired: 8 in, 2 out]
          }
          frame "ArmPressureCalculation" {
            n150 = call "ArmPressureCalcMethod.vi"() -> ()  [unwired: 12 in]
          }
          frame "EditDataFolder" {
            n151 = call "SaveDataPath.vi"() -> ("Changed"=w300:bool)  [unwired: 11 in]
            n152 = case shown="True" w300 {
              tunnel: w301 -> [_ w302]
              frame False {
              }
              frame True {
                n153 = call "AMC Send Local Message.vi"("Message Name"="ResetToDefault", "Message Queue in"=w302) -> ()  [unwired: 8 in, 2 out]
              }
            }
          }
          frame "EditJournalFolder" {
            n154 = call "SaveReportPath.vi"() -> ()  [unwired: 12 in]
          }
          frame "StartCalibration" {
            # "Calibration is stopped as userEvent"
            n155 = call "AE Variables.vi"("Action"=Enum_Variables."Get DAQ Connected") -> ("BooleanOut"=w304:bool)  [unwired: 11 in, 7 out]
            n156 = case shown="True" w304 {
              tunnel: w306 -> [_ w309]
              frame False {
                n157 = One Button Dialog(message="Acquisition module must be active") -> ()  [unwired: 1 in, 1 out]
              }
              frame True {
                n158 = call "AMC Send Local Messages.vi"("Message Names"=string[] ["Idle Monitor Reference", "Calibrate Pressure: Step 1", "Calibrate Pressure: Step 2"], "Message Queue in"=w309) -> ()  [unwired: 8 in, 2 out]
                n159 = call "stopCalibrationPopUp.vi"() -> ()  [unwired: 12 in]
              }
            }
          }
          frame "MeasurementTest" {
            n160 = call "AE Variables.vi"("Action"=Enum_Variables."Get DAQ Connected") -> ("BooleanOut"=w310:bool)  [unwired: 11 in, 7 out]
            n161 = case shown="True" w310 {
              tunnel: w312 -> [_ w313]
              frame False {
              }
              frame True {
                n162 = call "AMC Send Local Messages.vi"("Message Names"=string[] ["Stop Monitor Reference", "AcqTest", "Monitor Reference"], "Message Queue in"=w313) -> ()  [unwired: 8 in, 2 out]
              }
            }
          }
          frame "LowpassFilter" {
            n163 = call "acqFilterSelection.vi"() -> ()  [unwired: 12 in]
          }
          frame "Options" {
            n164 = call-by-ref "?"() -> ()  [unwired: 14 in, 2 out]
          }
          frame "FlowCalc" {
            n165 = call "AMC Send Local Message.vi"("Message Name"="Flow: View Signals", "Message Queue in"=w315) -> ()  [unwired: 8 in, 2 out]
          }
          frame "DICOM Server" {
            n166 = call "DICOMServerSettings.vi"() -> ()  [unwired: 12 in]
          }
          frame "EditDicomValues" {
            n167 = call "AMC Send Local Messages.vi"("Message Names"=string[] ["DCM: Edit Values"], "Message Queue in"=w318) -> ()  [unwired: 8 in, 2 out]
          }
          frame "ShowDicomValues" {
            n168 = call "AMC Send Local Messages.vi"("Message Names"=string[] ["DCM: Show Values"], "Message Queue in"=w320) -> ()  [unwired: 8 in, 2 out]
          }
          frame "Journal" {
            w321 = u16 0 items=["Journal", "Graph"]
            n169 = call "AE Variables.vi"("VariantIn"=w321, "Action"=Enum_Variables."Set JournalExport") -> ()  [unwired: 10 in, 8 out]
            n170 = call "AE Save.vi"("Variant In"=w321, "Action"=Enum_Save_Action_Events."SaveJournalType") -> ()  [unwired: 7 in, 2 out]
          }
          frame "Graph" {
            w324 = u16 1 items=["Journal", "Graph"]
            n171 = call "AE Variables.vi"("VariantIn"=w324, "Action"=Enum_Variables."Set JournalExport") -> ()  [unwired: 10 in, 8 out]
            n172 = call "AE Save.vi"("Variant In"=w324, "Action"=Enum_Save_Action_Events."SaveJournalType") -> ()  [unwired: 7 in, 2 out]
          }
          frame "Bitmap" {
            w327 = u16 0 items=["Bitmap", "JPEG"] ("Encoding")
            n173 = call "DICOMFileEncoding.vi"("Encoding"=w327) -> ()  [unwired: 11 in]
          }
          frame "JPEG" {
            w328 = u16 1 items=["Bitmap", "JPEG"] ("Encoding")
            n174 = call "DICOMFileEncoding.vi"("Encoding"=w328) -> ()  [unwired: 11 in]
          }
          frame "ChangePassword" {
            n175 = call "change_password.vi"() -> ()  [unwired: 12 in]
          }
          frame "UpdateProgram" {
            n176 = call "AMC Send Local Message.vi"("Message Name"="Update Program", "Message Queue in"=w330) -> ()  [unwired: 8 in, 2 out]
          }
          frame "ActivateDICOM" {
            n177 = call "Activation.vi"() -> ()  [unwired: 12 in]
          }
          frame "Danish" {
            (unwired) u16 0 ("Value (Signaling)")
          }
          frame "English" {
            (unwired) u16 1 ("Value (Signaling)")
          }
          frame "French" {
            (unwired) u16 2 ("Value (Signaling)")
          }
        }
      }
      event Menu Activation? {
        n178 = event-data() -> ("MenuRef"=w331:refnum<k9>)  [unwired: 1 out]
        n179 = call "AE Variables.vi"("Action"=Enum_Variables."Get DICOM Avail") -> ("BooleanOut"=w332:bool)  [unwired: 11 in, 7 out]
        n180 = case shown="True" w332 {
          tunnel: w331 -> [_ w334]
          frame False {
          }
          frame True {
            n181 = Get Menu Item Info(7:"FileEncoding" ("item tag"), 11:w334) -> (3:w342:refnum<k9>, 5:w343:string[])  [unwired: 1 in, 5 out]
            n182 = call "AE Variables.vi"("Action"=Enum_Variables."Get DICOM Encode") -> ("RingOut"=w341:u16)  [unwired: 11 in, 7 out]
            n183 = for {
              tunnel: w343 -> [w355] mode=indexing
              tunnel: w342 -> [w356]
              tunnel: w341 -> [w354]
              tunnel: [w351] -> w340
              i -> [w353]
              n184 = Equal?(x=w354, y=w353) -> (x = y?=w352:bool)
              n185 = Set Menu Item Info(6:w352, 7:w355, 11:w356) -> (3:w351:refnum<k9>)  [unwired: 4 in, 1 out]
            }
            n186 = Get Menu Item Info(7:"ExportType" ("item tag"), 11:w340) -> (3:w337:refnum<k9>, 5:w338:string[])  [unwired: 1 in, 5 out]
            n187 = call "AE Variables.vi"("Action"=Enum_Variables."Get JournalExport") -> ("RingOut"=w336:u16)  [unwired: 11 in, 7 out]
            n188 = for {
              tunnel: w338 -> [w349] mode=indexing
              tunnel: w337 -> [w350]
              tunnel: w336 -> [w348]
              i -> [w347]
              n189 = Equal?(x=w348, y=w347) -> (x = y?=w346:bool)
              n190 = Set Menu Item Info(6:w346, 7:w349, 11:w350) -> ()  [unwired: 4 in, 2 out]
            }
          }
        }
        n191 = event-data() -> ()  [unwired: 2 in, 1 out]
      }
    }
  }
  n192 = while "Primary Execution Loop" {
    shift-right: [w374] -> w17
    shift-left: w12 -> [w362]
    shift-right: [w371] -> _
    shift-left: _ -> [w365]
    shift-right: [w370] -> w16
    shift-left: w6 -> [w373]
    tunnel: w6 -> [w372]
    tunnel: w7 -> [w368]
    tunnel: w5 -> [w369]
    tunnel: [w358] -> w1 mode=indexing
    stop <- w366 stop-if-true
    # "<Dyn Events>"
    # "<Default Val>"
    n193 = call "AMC Read Next Message.vi"("error in (no error)"=w362, "timeout (1ms)"=w365, "Message Queue in"=w368) -> ("error out"=w364:errorcluster, "Message Value"=w363:string, "Message Name"=w360:string, "Message Queue out"=w367:T6, "Exit Process"=w366:bool)  [unwired: 2 in, 2 out]
    n194 = case shown="\"GenerateReport\"" w360 {
      selector: w360 -> [_ _ _ _ _ _ _ _ _ _ _ _ _ _ _ _ _ _ _ w615 _ _ _ _ _ _ _ _ _ _ _ _ _ _ _ _ _ _ _ _ _ _ _ _ _ _ _ _ _ _ _ _ _ _ _ _ _ _ _ _ _ _ _ _ _ _ _ _ _ _ _ _ _ _ _ _ _ _ _ _ _ _ _ _ _ _ _ _ _ _ _ _ _ _ _ _ _ _ _ _ _ _ _ _ _ _ _ _ _ _ _ _ _ _ _ _ _ _ _ _ w2306]
      tunnel: [w377 w390 w391 w399 w414 w429 w443 w459 w472 w487 w503 w514 w525 w531 w549 w568 w577 w586 w611 w627 w631 w635 w648 w666 w672 w683 w685 w686 w693 w699 w705 w711 w717 w720 w726 w738 w757 w783 w785 w786 w807 w817 w828 w833 w863 w886 w916 w923 w1075 w1107 w1124 w1145 w1165 w1173 w1182 w1207 w1225 w1242 w1284 w1295 w1312 w1325 w1328 w1346 w1367 w1395 w1401 w1403 w1411 w1419 w1420 w1435 w1470 w1495 w1503 w1512 w1523 w1537 w1547 w1562 w1572 w1579 w1598 w1618 w1658 w1686 w1700 w1708 w1729 w1774 w1784 w1786 w1790 w1796 w1801 w1827 w1834 w1843 w1852 w1856 w1878 w1909 w1930 w1940 w1959 w1977 w2024 w2044 w2078 w2101 w2122 w2157 w2187 w2202 w2219 w2236 w2275 w2282 w2299 w2304 w2310] -> w374
      tunnel: w364 -> [w379 w390 w392 w396 w416 w430 w444 w458 w473 w488 w502 w515 w525 w532 w556 w563 w579 w583 w612 w617 w631 w634 w659 w666 w670 w683 w685 w687 w694 w700 w706 w712 w718 w721 w726 w731 w762 w783 w785 w788 w814 w820 w828 w833 w867 w887 w916 w927 w1076 w1108 w1125 w1145 w1166 w1174 w1184 w1206 w1226 w1241 w1285 w1297 w1300 w1313 w1329 w1347 w1366 w1395 w1401 w1404 w1412 w1419 w1428 w1436 w1471 w1496 w1504 w1513 w1525 w1539 w1549 w1563 w1573 w1584 w1598 w1616 w1659 w1685 w1700 w1707 w1730 w1775 w1784 w1786 w1790 w1792 w1802 w1827 w1836 w1845 w1854 w1867 w1881 w1906 w1930 w1932 w1964 w1980 w2024 w2045 w2079 w2100 w2123 w2158 w2187 w2194 w2219 w2238 w2275 w2283 w2297 w2304 w2311]
      tunnel: w367 -> [w375 _ _ _ _ _ _ _ _ _ w511 w519 w523 _ _ _ _ _ _ _ _ _ _ _ _ _ _ _ _ _ _ _ _ _ _ _ _ _ _ w789 _ _ _ w832 w861 _ _ _ _ _ _ _ _ _ _ _ _ _ _ _ _ _ _ _ _ _ _ _ _ _ _ w1438 w1473 _ _ _ _ _ _ _ _ w1583 _ _ _ _ _ _ _ w1776 _ _ _ _ _ _ _ _ _ _ _ _ _ _ _ _ _ _ _ _ _ _ w2185 _ _ _ _ w2281 _ _ _]
      tunnel: w373 -> [w376 w389 w394 w409 w422 w437 w452 w467 w482 w497 w513 w521 w524 w540 w545 w567 w582 w585 w614 w623 w630 w633 w664 w665 w681 w682 w684 w689 w692 w697 w703 w709 w715 w724 w725 w737 w760 w782 w784 w792 w816 w826 w827 w830 w860 w888 w913 w939 w1074 w1103 w1126 w1144 w1156 w1176 w1178 w1205 w1229 w1231 w1273 w1290 w1304 w1317 w1327 w1345 w1365 w1394 w1398 w1410 w1415 w1418 w1426 w1442 w1476 w1502 w1507 w1511 w1526 w1540 w1550 w1566 w1575 w1582 w1597 w1619 w1657 w1692 w1698 w1715 w1732 w1778 w1783 w1785 w1789 w1795 w1799 w1826 w1833 w1842 w1851 w1866 w1875 w1903 w1929 w1939 w1962 w1992 w2023 w2052 w2082 w2107 w2131 w2173 w2186 w2201 w2218 w2241 w2274 w2278 w2302 w2303 w2312]
      tunnel: w372 -> [_ _ _ _ _ _ _ _ _ _ _ _ _ _ _ _ _ _ _ _ _ _ _ _ _ _ _ _ _ _ _ _ _ _ _ _ _ _ _ _ _ _ _ _ _ _ _ _ _ _ _ _ _ _ _ _ _ _ _ _ _ _ _ _ _ _ _ _ _ _ _ _ _ _ _ _ _ _ _ _ _ _ _ _ _ _ _ _ _ _ _ _ _ _ _ _ _ _ _ _ _ _ _ _ _ _ _ _ _ _ _ _ _ _ _ _ _ _ _ _ _]
      tunnel: [w376 w389 w394 w408 w421 w436 w451 w466 w481 w496 w513 w521 w524 w540 w545 w567 w582 w587 w614 w622 w630 w636 w664 w665 w681 w682 w684 w689 w691 w696 w702 w708 w714 w724 w725 w736 w759 w782 w784 w792 w816 w826 w827 w830 w868 w888 w913 w938 w1074 w1109 w1126 w1143 w1156 w1176 w1178 w1205 w1229 w1240 w1272 w1290 w1304 w1317 w1327 w1345 w1365 w1394 w1397 w1410 w1414 w1418 w1425 w1442 w1476 w1502 w1507 w1511 w1526 w1540 w1550 w1565 w1577 w1586 w1597 w1619 w1656 w1691 w1705 w1715 w1751 w1778 w1783 w1785 w1788 w1795 w1798 w1826 w1833 w1842 w1851 w1866 w1875 w1903 w1929 w1941 w1961 w1992 w2023 w2052 w2082 w2107 w2131 w2173 w2186 w2200 w2218 w2241 w2274 w2277 w2302 w2303 w2312] -> w370
      tunnel: [200 _ _ _ _ _ _ _ _ _ _ _ _ _ _ _ _ _ _ _ _ _ _ _ _ _ _ _ _ _ _ _ _ _ _ _ _ _ _ _ _ _ _ _ _ _ _ _ _ _ _ _ _ _ _ _ _ _ _ _ _ _ _ _ _ _ _ _ _ _ _ _ _ _ _ _ _ _ _ _ _ _ _ _ _ _ _ _ _ _ _ _ _ _ _ _ _ _ _ _ _ _ _ _ _ _ _ _ _ _ _ _ _ _ _ _ _ _ _ _ _] -> w371
      tunnel: w369 -> [_ _ _ _ _ _ _ _ _ _ _ _ _ _ _ _ _ _ _ w621 _ _ _ _ _ _ _ _ _ _ _ _ _ _ _ _ _ _ _ _ _ _ _ _ _ _ _ _ _ _ _ _ _ _ _ _ _ _ _ _ _ _ _ _ _ _ _ _ _ _ _ _ _ _ _ _ _ _ _ _ _ _ _ _ _ _ _ _ _ _ _ _ _ _ _ _ _ _ _ _ _ _ _ _ _ _ _ _ _ _ _ _ _ _ _ _ _ _ _ _ _]
      tunnel: w363 -> [_ _ _ _ _ _ _ _ _ _ _ _ _ _ _ _ _ _ _ _ _ _ _ _ _ _ _ _ _ _ _ _ _ _ _ _ _ _ _ _ _ _ _ w831 _ _ _ _ _ _ _ _ _ _ _ _ _ w1236 _ _ w1302 w1315 _ _ _ _ _ w1406 _ _ _ _ _ _ _ _ _ _ _ _ _ _ _ _ _ _ _ _ _ _ _ _ w1787 _ _ _ _ _ _ w1863 w1876 w1908 _ w1936 _ w1995 _ _ _ _ _ _ _ _ _ _ _ _ _ _ _]
      frame "", "Idle" {
        n195 = Unbundle By Name(w376) -> ("Reference signal.Monitor"=w378:bool)
        n196 = case shown="True" w378 {
          tunnel: w379 -> [w381 w388]
          tunnel: [w381 w385] -> w377
          tunnel: w375 -> [_ w383]
          frame False {
          }
          frame True {
            n197 = call "AE Events.vi"("error in (no error)"=w388, "Action"=enum16{"Init", "Get Event", "Set Event"}."Get Event") -> ("error out"=w386:errorcluster, "Event Out"=w382:dbl)  [unwired: 8 in]
            n198 = call "AE Paper.vi"("error in (no error)"=w386, "Message Queue in"=w383, "Events"=w382, "Action Events"=Enum_Paper_Action_Events."Paper State") -> ("error out"=w385:errorcluster)  [unwired: 5 in, 1 out]
          }
        }
      }
      frame "/*********Initialize********/" {
      }
      frame "preInitialize" {
        n199 = control-ref of="This VI"() -> (w393:refnum<vi>)
        n200 = call <vilib>:"Set Busy.vi"("error in (no error)"=w392, "VI reference (current VI)"=w393) -> ("error out"=w391:errorcluster)  [unwired: 8 in, 1 out]
      }
      frame "Initialize: PageMenu" {
        n201 = vi-ref "main.lvlib:Top Menu.vi"() -> (w402:refnum<vi>)
        n202 = call "Notifier AE.vi"("error in (no error)"=w396, "String"="Initialising Pages") -> ("error out"=w395:errorcluster)  [unwired: 9 in]
        n203 = property class="VI"(reference=w402) -> ("Name"=w401:string)  [unwired: 1 in, 2 out]
        n204 = Obtain Queue(name (unnamed)="Menu Queue", element data type=cluster{"Msg":string, "Data":variant} {"Msg"="", "Data"=variant}, error in (no error)=w395) -> (queue out=w400:refnum<queue>, error out=w403:errorcluster)  [unwired: 2 in, 1 out]
        n205 = Open VI Reference(type specifier VI Refnum (for type only)=refnum<vi> refnum, vi path=w401, options=128, error in (no error)=w403) -> (vi reference=w407:refnum<vi>, error out=w406:errorcluster)  [unwired: 2 in]
        n206 = call-by-ref "Start Asynchronous Call"(reference=w407, error in=w406, "Menu Queue"=w400) -> (reference out=w398:refnum<vi>, error out=w399:errorcluster)  [unwired: 11 in]
        n207 = Bundle By Name(cluster=w409, "PageMenu.VI Reference"=w398, "PageMenu.Queue"=w400) -> (w408:T3)
      }
      frame "Initialize: Profile" {
        n208 = vi-ref "main.lvlib:Profile.vi"() -> (w413:refnum<vi>)
        n209 = property class="VI"(reference=w413) -> ("Name"=w412:string)  [unwired: 1 in, 2 out]
        n210 = Obtain Queue(name (unnamed)="Profile Queue", element data type=cluster{"Msg":string, "Data":variant} {"Msg"="", "Data"=variant}, error in (no error)=w416) -> (queue out=w417:refnum<queue>, error out=w415:errorcluster)  [unwired: 2 in, 1 out]
        n211 = Open VI Reference(type specifier VI Refnum (for type only)=refnum<vi> refnum, vi path=w412, options=128, error in (no error)=w415) -> (vi reference=w420:refnum<vi>, error out=w418:errorcluster)  [unwired: 2 in]
        n212 = call-by-ref "Start Asynchronous Call"(reference=w420, error in=w418, "Queue In"=w417) -> (reference out=w419:refnum<vi>, error out=w414:errorcluster)  [unwired: 11 in]
        n213 = Bundle By Name(cluster=w422, "Profile.VI Reference"=w419, "Profile.Queue"=w417) -> (w421:T3)
      }
      frame "Initialize: Configuration" {
        n214 = vi-ref "main.lvlib:Configuration.vi"() -> (w427:refnum<vi>)
        n215 = property class="VI"(reference=w427) -> ("Name"=w432:string)  [unwired: 1 in, 2 out]
        n216 = Obtain Queue(name (unnamed)="Configuration Queue", element data type=cluster{"Msg":string, "Data":variant} {"Msg"="", "Data"=variant}, error in (no error)=w430) -> (queue out=w428:refnum<queue>, error out=w431:errorcluster)  [unwired: 2 in, 1 out]
        n217 = Open VI Reference(type specifier VI Refnum (for type only)=refnum<vi> refnum, vi path=w432, options=128, error in (no error)=w431) -> (vi reference=w435:refnum<vi>, error out=w433:errorcluster)  [unwired: 2 in]
        n218 = call-by-ref "Start Asynchronous Call"(reference=w435, error in=w433, "Queue In"=w428) -> (reference out=w434:refnum<vi>, error out=w429:errorcluster)  [unwired: 11 in]
        n219 = Bundle By Name(cluster=w437, "Configuration.VI Reference"=w434, "Configuration.Queue"=w428) -> (w436:T3)
      }
      frame "Initialize: Configuration Tables" {
        n220 = vi-ref "main.lvlib:Configuration_table.vi"() -> (w447:refnum<vi>)
        n221 = property class="VI"(reference=w447) -> ("Name"=w446:string)  [unwired: 1 in, 2 out]
        n222 = Obtain Queue(name (unnamed)="Configuration Queue", element data type=cluster{"Msg":string, "Data":variant} {"Msg"="", "Data"=variant}, error in (no error)=w444) -> (queue out=w442:refnum<queue>, error out=w445:errorcluster)  [unwired: 2 in, 1 out]
        n223 = Open VI Reference(type specifier VI Refnum (for type only)=refnum<vi> refnum, vi path=w446, options=128, error in (no error)=w445) -> (vi reference=w450:refnum<vi>, error out=w448:errorcluster)  [unwired: 2 in]
        n224 = call-by-ref "Start Asynchronous Call"(reference=w450, error in=w448, "Queue In"=w442) -> (reference out=w449:refnum<vi>, error out=w443:errorcluster)  [unwired: 11 in]
        n225 = Bundle By Name(cluster=w452, "Configuration.VI Reference"=w449, "Configuration.Queue"=w442) -> (w451:T3)
      }
      frame "Initialize: Acquisition" {
        n226 = vi-ref "main.lvlib:Acquisition.vi"() -> (w462:refnum<vi>)
        n227 = Obtain Queue(name (unnamed)="Acquisition Queue", element data type=cluster{"Msg":string, "Data":variant} {"Msg"="", "Data"=variant}, error in (no error)=w458) -> (queue out=w457:refnum<queue>, error out=w460:errorcluster)  [unwired: 2 in, 1 out]
        n228 = property class="VI"(reference=w462) -> ("Name"=w461:string)  [unwired: 1 in, 2 out]
        n229 = Open VI Reference(type specifier VI Refnum (for type only)=refnum<vi> refnum, vi path=w461, options=128, error in (no error)=w460) -> (vi reference=w465:refnum<vi>, error out=w463:errorcluster)  [unwired: 2 in]
        n230 = call-by-ref "Start Asynchronous Call"(reference=w465, error in=w463, "Queue In"=w457) -> (reference out=w464:refnum<vi>, error out=w459:errorcluster)  [unwired: 11 in]
        n231 = Bundle By Name(cluster=w467, "Acquisition.VI Reference"=w464, "Acquisition.Queue"=w457) -> (w466:T3)
      }
      frame "Initialize: Data" {
        n232 = Obtain Queue(name (unnamed)="Data Queue", element data type=cluster{"Msg":string, "Data":variant} {"Msg"="", "Data"=variant}, error in (no error)=w473) -> (queue out=w475:refnum<queue>, error out=w474:errorcluster)  [unwired: 2 in, 1 out]
        n233 = vi-ref "main.lvlib:Data.vi"() -> (w477:refnum<vi>)
        n234 = property class="VI"(reference=w477) -> ("Name"=w476:string)  [unwired: 1 in, 2 out]
        n235 = Open VI Reference(type specifier VI Refnum (for type only)=refnum<vi> refnum, vi path=w476, options=128, error in (no error)=w474) -> (vi reference=w480:refnum<vi>, error out=w478:errorcluster)  [unwired: 2 in]
        n236 = call-by-ref "Start Asynchronous Call"(reference=w480, error in=w478, "Queue In"=w475) -> (reference out=w479:refnum<vi>, error out=w472:errorcluster)  [unwired: 11 in]
        n237 = Bundle By Name(cluster=w482, "Data.VI Reference"=w479, "Data.Queue"=w475) -> (w481:T3)
      }
      frame "Initialize: Journal" {
        n238 = vi-ref "main.lvlib:Journal.vi"() -> (w492:refnum<vi>)
        n239 = Obtain Queue(name (unnamed)="Journal Queue", element data type=cluster{"Msg":string, "Data":variant} {"Msg"="", "Data"=variant}, error in (no error)=w488) -> (queue out=w490:refnum<queue>, error out=w489:errorcluster)  [unwired: 2 in, 1 out]
        n240 = property class="VI"(reference=w492) -> ("Name"=w491:string)  [unwired: 1 in, 2 out]
        n241 = Open VI Reference(type specifier VI Refnum (for type only)=refnum<vi> refnum, vi path=w491, options=128, error in (no error)=w489) -> (vi reference=w495:refnum<vi>, error out=w493:errorcluster)  [unwired: 2 in]
        n242 = call-by-ref "Start Asynchronous Call"(reference=w495, error in=w493, "Queue In"=w490) -> (reference out=w494:refnum<vi>, error out=w487:errorcluster)  [unwired: 11 in]
        n243 = Bundle By Name(cluster=w497, "Journal.VI Reference"=w494, "Journal.Queue"=w490) -> (w496:T3)
      }
      frame "Send Caller Queue to Journal" {
        w508 = cluster{"Msg":string, "Data":variant} {"Msg"="", "Data"=variant} ("element")
        # "To make sure all references are passed to References.vi the rest of the initialization is activated from Journal.vi"
        n244 = Unbundle By Name(w513) -> ("Journal.Queue"=w512:refnum<queue>)
        n245 = Bundle By Name(cluster=w508, "Msg"="Set Caller Queue", "Data"=w511) -> (w510:cluster{"Msg":string, "Data":variant})
        n246 = Enqueue Element(queue=w512, element=w510, error in (no error)=w502) -> (queue out=w506:refnum<queue>, error out=w504:errorcluster)  [unwired: 1 in, 1 out]
        n247 = Bundle By Name(cluster=w508, "Msg"="Register Refs") -> (w505:cluster{"Msg":string, "Data":variant})
        n248 = Enqueue Element(queue=w506, element=w505, error in (no error)=w504) -> (error out=w503:errorcluster)  [unwired: 1 in, 2 out]
      }
      frame "Send Caller Queue to Acquisition" {
        # "To control the acquisition"
        n249 = Unbundle By Name(w521) -> ("Acquisition.Queue"=w520:refnum<queue>)
        n250 = Bundle By Name(cluster=cluster{"Msg":string, "Data":variant} {"Msg"="", "Data"=variant} ("element"), "Msg"="Set Caller Queue", "Data"=w519) -> (w518:cluster{"Msg":string, "Data":variant})
        n251 = Enqueue Element(queue=w520, element=w518, error in (no error)=w515) -> (error out=w514:errorcluster)  [unwired: 1 in, 2 out]
      }
      frame "Continue Initializing" {
        w522 = string[] ["Send Caller Queue to Acquisition", "Register User Parameters", "InitNewTest", "Initialize", "Change Language", "Initialize: Dicom", "Load Patient Register", "Cache User Parameters", "Load Hospital Info", "Subpanel: Load Menu", "Subpanel: Load Profile", "Reset Graphs", "Set SubVi Color", "Silent DAQ Initialization", "Update Display", "Set Acquisition Mode", "BT: Initialize", "Set Height", "ResetToDefault", "End Initializing"]  # Initial Elements
        n252 = call "AMC Send Local Messages.vi"("Message Names"=w522, "Message Queue in"=w523) -> ()  [unwired: 8 in, 2 out]
      }
      frame "Set SubVi Color" {
        w526 = u32 16777226
        n253 = Unbundle By Name(w540) -> ("PageMenu.Queue"=w539:refnum<queue>, "Profile.Queue"=w538:refnum<queue>, "Configuration.Queue"=w537:refnum<queue>, "Acquisition.Queue"=w536:refnum<queue>, "Data.Queue"=w535:refnum<queue>, "Journal.Queue"=w534:refnum<queue>)
        n254 = Bundle By Name(cluster=cluster{"Msg":string, "Data":variant} {"Msg"="", "Data"=variant} ("element"), "Msg"="Set Color", "Data"=w526) -> (w528:cluster{"Msg":string, "Data":variant})
        n255 = control-ref of="This VI"() -> (w527:refnum<vi>)
        n256 = call "Set VI Color.vi"("Pane Color"=w526, "VI in"=w527) -> ()  [unwired: 10 in]
        n257 = Build Array(w539, w538, w537, w536, w535, w534) -> (w533:refnum<queue>[])
        n258 = for {
          tunnel: w533 -> [w544] mode=indexing
          shift-right: [w543] -> w531
          shift-left: w532 -> [w542]
          tunnel: w528 -> [w541]
          n259 = Enqueue Element(queue=w544, element=w541, error in (no error)=w542) -> (error out=w543:errorcluster)  [unwired: 1 in, 2 out]
        }
      }
      frame "Initialize" {
        n260 = Unbundle By Name(w545) -> ("cRef.Profile.References.ListboxDoctor"=w552:refnum<vi>, "cRef.Profile.References.ListboxOperator"=w551:refnum<vi>)
        n261 = call "UpdateGlobals.vi"("error in (no error)"=w556, "Operator Listbox Ref"=w551, "Doctor Listbox Ref"=w552) -> ("error out"=w550:errorcluster)  [unwired: 7 in]
        n262 = call "AE DataProcessControl.vi"("Action"=Enum_Process_Data."Init", "error in (no error)"=w550) -> ("error out"=w557:errorcluster)  [unwired: 7 in, 2 out]
        n263 = call "AE Variables.vi"("VariantIn"=TRUE, "error in (no error)"=w557, "Action"=Enum_Variables."Set Encryption") -> ("error out"=w555:errorcluster)  [unwired: 9 in, 7 out]
        n264 = call "AE Variables.vi"("error in (no error)"=w555, "Action"=Enum_Variables."Set ExcelVersion") -> ("error out"=w553:errorcluster)  [unwired: 10 in, 7 out]
        n265 = call "PassNill.vi"("Error In"=w553) -> ("Error Out"=w546:errorcluster)  [unwired: 10 in]
        n266 = call-poly <userlib>:"MGI Suppress Error Code.vi"("Error Code"=666, "Error In"=w546) -> ("Error Supressed?"=w547:bool, "Error Out"=w549:errorcluster)  [unwired: 4 in]
        n267 = disable-structure shown="Default" {
          disable-tunnel: w547 -> [w561 _]
          frame condition #0 {
            n268 = Quit LabVIEW(quit? (T)=w561) -> ()
          }
          frame condition #1 (active) {
          }
        }
      }
      frame "Initialize: Dicom" {
        n269 = Unbundle By Name(w567) -> ("cRef.Profile.References.Query Worklist"=w566:refnum<vi>, "cRef.Journal.References.Send To PACS"=w565:refnum<vi>)
        n270 = call "CheckLicens.vi"("error in (no error)"=w563) -> ("error out"=w564:errorcluster, "Dicom Active"=w562:bool)  [unwired: 9 in]
        n271 = case shown="False" w562 {
          frame False {
            n272 = Current VI's Menubar() -> (w576:refnum<k9>)
            n273 = Delete Menu Items(7:"DICOM" ("item name"), 9:w576) -> ()  [unwired: 2 in, 2 out]
          }
          frame True {
          }
        }
        n274 = property class="Bool"(reference=w565, "Visible"=w562) -> ()  [unwired: 1 in, 2 out]
        n275 = property class="Bool"(reference=w566, "Visible"=w562) -> ()  [unwired: 1 in, 2 out]
        n276 = case shown="True" w562 {
          tunnel: w564 -> [w569 w572]
          tunnel: [w569 w573] -> w568
          frame False {
          }
          frame True {
            n277 = call "AE Save.vi"("error in (no error)"=w572, "Action"=Enum_Save_Action_Events."Load Dicom Tags") -> ("error out"=w571:errorcluster)  [unwired: 7 in, 1 out]
            n278 = call "AE DICOM.vi"("Action"=Enum_DICOM."Set Dicom Encoding", "Error In"=w571) -> ("Error Out"=w573:errorcluster)  [unwired: 9 in]
          }
        }
      }
      frame "postInitialize" {
        n279 = control-ref of="This VI"() -> (w581:refnum<vi>)
        n280 = call <vilib>:"Unset Busy.vi"("error in (no error)"=w579, "VI reference (current VI)"=w581) -> ("error out"=w578:errorcluster)  [unwired: 9 in]
        n281 = property class="VI"(reference=w581, error in=w578, "FP:Transparency"=u8 0 ("Front Panel Window:Transparency")) -> (error out=w577:errorcluster)  [unwired: 1 out]
      }
      frame "Initialize Reference" {
        n282 = Unbundle By Name(w585) -> ("Data Acquisition.Control?"=w584:bool)
        n283 = case shown="False" w584 {
          tunnel: [w608 w609] -> w587
          tunnel: [w590 w610] -> w586
          tunnel: w583 -> [w589 w610]
          tunnel: w585 -> [w588 w609]
          frame False {
            # "Initialize reference  signal acquisition"
            n284 = vi-ref "main.lvlib:RefData(SubVI).vi"() -> (w599:refnum<vi>)
            n285 = property class="VI"(reference=w599) -> ("Name"=w598:string)  [unwired: 1 in, 2 out]
            n286 = Open VI Reference(type specifier VI Refnum (for type only)=refnum<vi> refnum, vi path=w598, options=128, error in (no error)=w589) -> (vi reference=w595:refnum<vi>, error out=w596:errorcluster)  [unwired: 2 in]
            n287 = call-by-ref "Start Asynchronous Call"(reference=w595, error in=w596) -> (reference out=w592:refnum<vi>, error out=w593:errorcluster)  [unwired: 1 in, 1 out]
            n288 = Obtain Queue(name (unnamed)="RefControl", element data type="", error in (no error)=w593) -> (queue out=w602:refnum<queue>, error out=w601:errorcluster)  [unwired: 2 in, 1 out]
            n289 = Flush Queue(queue=w602, error in (no error)=w601) -> (queue out=w600:refnum<queue>, error out=w591:errorcluster)  [unwired: 1 out]
            n290 = Close Reference(reference=w592, error in (no error)=w591) -> (error out=w590:errorcluster)
            n291 = Bundle By Name(cluster=w588, "Reference signal.Queue"=w600, "Reference signal.Monitor"=TRUE, "System Parameters.Paper Running?"=FALSE ("Paper Running?"), "Reference signal.Events"=0.0) -> (w608:T3)
          }
          frame True {
          }
        }
      }
      frame "End Initializing" {
        n292 = call "Notifier AE.vi"("error in (no error)"=w612, "String"="Ready") -> ("error out"=w611:errorcluster)  [unwired: 9 in]
      }
      frame "Register User Parameters" {
        w628 = ""  # Event
        n293 = call "Notifier AE.vi"("error in (no error)"=w617, "String"=w615) -> ("error out"=w616:errorcluster)  [unwired: 9 in]
        n294 = Create User Event(user event datatype=w628, error in=w616) -> (user event=w620:refnum<user-event>, error out=w626:errorcluster)
        n295 = call "Register User Parameters.vi"("User Events"=w620, "error in (no error)"=w617, "SHIFTER DATA"=w623, "Event Registration Refnum in"=w621) -> ("error out"=w619:errorcluster)  [unwired: 7 in]
        n296 = call "References.vi"("error in"=w619, "Reference AE Control"=Reference_AE_Control."Get") -> ("error out"=w618:errorcluster, "Cluster out"=w624:T5)  [unwired: 8 in]
        n297 = call "AE User Events.vi"("Action"=Enum_User_Events."Init", "user event in"=w620) -> ()  [unwired: 8 in, 2 out]
        n298 = Bundle By Name(cluster=w623, "cRef"=w624) -> (w622:T3)
        n299 = Merge Errors(w618, w626) -> (w627:errorcluster)
      }
      frame "/*********Display Updates********/" {
      }
      frame "Cache User Parameters" {
        n300 = Unbundle By Name(w633) -> ("cRef.Configuration.Method"=w632:string)
        n301 = case shown="\"new\", Default" w632 {
          tunnel: [w638 w644] -> w636
          tunnel: [w637 w643] -> w635
          tunnel: w634 -> [w639 w642]
          tunnel: w633 -> [w640 w641]
          frame "new", Default {
            n302 = call "Cache User Parameters_new method.vi"("error in (no error)"=w639, "SHIFTER DATA in"=w640) -> ("error out"=w637:errorcluster, "SHIFTER DATA out"=w638:T3)  [unwired: 8 in]
          }
          frame "old" {
            n303 = call "Cache User Parameters.vi"("error in (no error)"=w642, "SHIFTER DATA in"=w641) -> ("error out"=w643:errorcluster, "SHIFTER DATA out"=w644:T3)  [unwired: 8 in]
          }
        }
      }
      frame "Update Display" {
        n304 = Unbundle By Name(w664) -> ("cRef.Menu.References.PersonalInfoString"=w652:refnum<vi>, "User Parameters.Name"=w650:string, "User Parameters.CPR Number"=w651:string, "cRef.Data.References.AdjustedHeight"=w656:refnum<vi>, "cRef.Acquisition.References.SegmentAcqString"=w663:refnum<vi>, "User Parameters.Measuring Limb"=w662:string, "cRef.Menu.References.MenuStartADC"=w661:refnum<vi>)
        n305 = call "AE Variables.vi"("error in (no error)"=w659, "Action"=Enum_Variables."Get DAQ Connected") -> ("BooleanOut"=w658:bool, "error out"=w657:errorcluster)  [unwired: 10 in, 6 out]
        n306 = property class="Bool (strict)"(reference=w661, error in=w657, "Value"=w658) -> (error out=w645:errorcluster)  [unwired: 1 out]
        n307 = property class="Str"(reference=w663, error in=w645, "Value"=w662) -> (error out=w655:errorcluster)  [unwired: 1 out]
        n308 = call "AE Variables.vi"("Action"=Enum_Variables."Get Recorded Height") -> ("NumericOut"=w647:dbl)  [unwired: 11 in, 7 out]
        n309 = property class="DigNum (strict)"(reference=w656, error in=w655, "Val(Sgnl)"=w647) -> (error out=w649:errorcluster)  [unwired: 1 out]
        n310 = Concatenate Strings(w650, "\r", w651) -> (w653:string)
        n311 = property class="Str"(reference=w652, error in=w649, "Value"=w653) -> (error out=w648:errorcluster)  [unwired: 1 out]
      }
      frame "/ ***Language***/" {
      }
      frame "Change Language" {
        n312 = call "AE Variables.vi"("Action"=Enum_Variables."Get Language") -> ("RingOut"=w667:u16)  [unwired: 11 in, 7 out]
        n313 = call "getAllRefs.vi"("error in (no error)"=w670, "Language"=w667, "Change Language"=TRUE) -> ("error out"=w669:errorcluster)  [unwired: 7 in, 1 out]
        n314 = Current VI's Path() -> (path=w677:path)
        n315 = Strip Path(path=w677) -> (stripped path=w676:path)  [unwired: 1 out]
        n316 = Index Array(array=string[] ["DM2000RuntimeMenu.rtm", "DM2000RuntimeMenuEng.rtm", "DM2000RuntimeMenuFrench.rtm"], index=w667) -> (element=w678:string)
        n317 = control-ref of="This VI"() -> (w680:refnum<vi>)
        n318 = Build Path(base path=w676, name or relative path=w678) -> (appended path=w675:path)
        n319 = property class="VI"(reference=w680, error in=w669, "RT Menu Path"=w675) -> (reference out=w673:refnum<vi>, error out=w674:errorcluster)
        n320 = Close Reference(reference=w673, error in (no error)=w674) -> (error out=w672:errorcluster)
      }
      frame "/*********Primary Execution********/" {
      }
      frame "/***Subpanel Control***/" {
      }
      frame "Subpanel: Load Menu" {
        n321 = Unbundle By Name(w689) -> ("PageMenu.VI Reference"=w688:refnum<vi>)
        n322 = invoke on="Top Subpanel" class="SubPanel" method="Insert VI"(error in=w687, "VI Ref"=w688) -> (error out=w686:errorcluster)  [unwired: 2 in, 3 out]
      }
      frame "Subpanel: Load Profile" {
        n323 = Unbundle By Name(w692) -> ("Profile.VI Reference"=w695:refnum<vi>)
        n324 = invoke on="Main Subpanel" class="SubPnl" method="Insert VI"(error in=w694, "VI Ref"=w695) -> (error out=w693:errorcluster)  [unwired: 2 in, 3 out]
        n325 = Bundle By Name(cluster=w692, "System Parameters.Active Page"="Profile") -> (w691:T3)
      }
      frame "Subpanel: Load Configuration" {
        n326 = Unbundle By Name(w697) -> ("Configuration.VI Reference"=w701:refnum<vi>)
        n327 = invoke on="Main Subpanel" class="SubPanel" method="Insert VI"(error in=w700, "VI Ref"=w701) -> (error out=w699:errorcluster)  [unwired: 2 in, 3 out]
        n328 = Bundle By Name(cluster=w697, "System Parameters.Active Page"="Configuration") -> (w696:T3)
      }
      frame "Subpanel: Load Acquisition" {
        n329 = Unbundle By Name(w703) -> ("Acquisition.VI Reference"=w707:refnum<vi>)
        n330 = invoke on="Main Subpanel" class="SubPanel" method="Insert VI"(error in=w706, "VI Ref"=w707) -> (error out=w705:errorcluster)  [unwired: 2 in, 3 out]
        n331 = Bundle By Name(cluster=w703, "System Parameters.Active Page"="Acquisition") -> (w702:T3)
      }
      frame "Subpanel: Load Data" {
        n332 = Unbundle By Name(w709) -> ("Data.VI Reference"=w713:refnum<vi>)
        n333 = invoke on="Main Subpanel" class="SubPanel" method="Insert VI"(error in=w712, "VI Ref"=w713) -> (error out=w711:errorcluster)  [unwired: 2 in, 3 out]
        n334 = Bundle By Name(cluster=w709, "System Parameters.Active Page"="Data") -> (w708:T3)
      }
      frame "Subpanel: Load Journal" {
        n335 = Unbundle By Name(w715) -> ("Journal.VI Reference"=w719:refnum<vi>)
        n336 = invoke on="Main Subpanel" class="SubPanel" method="Insert VI"(error in=w718, "VI Ref"=w719) -> (error out=w717:errorcluster)  [unwired: 2 in, 3 out]
        n337 = Bundle By Name(cluster=w715, "System Parameters.Active Page"="Journal") -> (w714:T3)
      }
      frame "Subpanel: Set Splitters" {
        n338 = Unbundle By Name(w724) -> ("Configuration.Queue"=w723:refnum<queue>)
        n339 = Enqueue Element(queue=w723, element=cluster{"Msg":string, "Data":variant} {"Msg"="Set Splitter", "Data"=variant}, error in (no error)=w721) -> (error out=w720:errorcluster)  [unwired: 1 in, 2 out]
      }
      frame "/*** Bluetooth ***/" {
      }
      frame "BT: Initialize" {
        n340 = call "AE Save.vi"("error in (no error)"=w731, "Action"=Enum_Save_Action_Events."Load BT License") -> ("error out"=w734:errorcluster, "Anything"=w733:variant)  [unwired: 7 in]
        n341 = Variant To Data(error in=w734, type=T17 {"License"="", "Accepted Serials"=[]} ("data"), Variant=w733) -> (data=w728:T17, error out=w730:errorcluster)
        n342 = Unbundle By Name(w728) -> ("License"=w727:string)
        n343 = Empty String/Path?(string/path=w727) -> (empty?=w732:bool)
        n344 = case shown="False" w732 {
          tunnel: [w742 w756] -> w738
          tunnel: w730 -> [w740 w756]
          tunnel: w737 -> [w748 w755]
          tunnel: [w747 w755] -> w736
          frame False {
            # "Start listening for incomming BT messages"
            n345 = vi-ref "main.lvlib:AsyncBluetoothHandler.vi"() -> (w750:refnum<vi>)
            n346 = property class="VI"(reference=w750, error in=w740) -> (error out=w739:errorcluster, "Name"=w749:string)  [unwired: 1 out]
            n347 = Open VI Reference(type specifier VI Refnum (for type only)=refnum<vi> refnum, vi path=w749, options=128, error in (no error)=w739) -> (vi reference=w752:refnum<vi>, error out=w751:errorcluster)  [unwired: 2 in]
            n348 = Obtain Queue(element data type=cluster{"Cmd":string, "Msg":string} {"Cmd"="", "Msg"=""}, error in (no error)=w740) -> (queue out=w746:refnum<queue>, error out=w743:errorcluster)  [unwired: 3 in, 1 out]
            n349 = call-by-ref "Start Asynchronous Call"(reference=w752, error in=w751, "Queue"=w746) -> (reference out=w745:refnum<vi>, error out=w741:errorcluster)  [unwired: 11 in]
            n350 = Merge Errors(w741, w743) -> (w742:errorcluster)
            n351 = Bundle By Name(cluster=w748, "Bluetooth.VI Reference"=w745, "Bluetooth.Queue"=w746) -> (w747:T3)
          }
          frame True {
          }
        }
      }
      frame "BT: Dequeue Element" {
        n352 = Unbundle By Name(w760) -> ("Bluetooth.Queue"=w766:refnum<queue>)
        n353 = Dequeue Element(queue=w766, timeout in ms (-1)=10, error in (no error)=w762) -> (element=w765:cluster{"Cmd":string, "Msg":string}, error out=w761:errorcluster)  [unwired: 2 out]
        n354 = Unbundle By Name(w765) -> ("Cmd"=w764:string, "Msg"=w763:string)
        n355 = case shown="\"BTelement\"" w764 {
          tunnel: w763 -> [w767 w770 w776]
          tunnel: w761 -> [w768 w771 w774]
          tunnel: [w768 w771 w775] -> w757
          tunnel: w760 -> [w769 w772 w773]
          tunnel: [w769 w772 w773] -> w759
          frame "False", Default {
            n356 = One Button Dialog(message=w767) -> ()  [unwired: 1 in, 1 out]
          }
          frame "Error" {
            # "Handle .NET error"
            n357 = One Button Dialog(message=w770) -> ()  [unwired: 1 in, 1 out]
          }
          frame "BTelement" {
            # "Received new Bluetooth message"
            n358 = call "HandleMessage.vi"("error in (no error)"=w774, "Msg"=w776, "SHIFTER DATA"=w773) -> ("error out"=w775:errorcluster)  [unwired: 7 in, 1 out]
          }
        }
      }
      frame "BT: Stop" {
        n359 = Unbundle By Name(w782) -> ("Bluetooth.Queue"=w781:refnum<queue>, "Bluetooth.VI Reference"=w780:refnum<vi>)
        n360 = Release Queue(queue=w781) -> (error out=w778:errorcluster)  [unwired: 2 in, 2 out]
        n361 = Close Reference(reference=w780) -> (error out=w779:errorcluster)  [unwired: 1 in]
        n362 = Merge Errors(w778, w779) -> (w777:errorcluster)
        n363 = call <vilib>:"Clear Errors.vi"("error in (no error)"=w777) -> ()  [unwired: 6 in, 1 out]
      }
      frame "/*** Menu ***/" {
      }
      frame "Update Program" {
        n364 = call "Update.vi"("error in (no error)"=w788) -> ("error out"=w787:errorcluster, "Update"=w790:bool, "UpdatePath"=w791:string)  [unwired: 8 in]
        n365 = case shown="True" w790 {
          tunnel: w789 -> [_ w805]
          tunnel: w791 -> [_ w798]
          tunnel: w787 -> [w793 w795]
          tunnel: [w793 w794] -> w786
          frame False {
          }
          frame True {
            w797 = "\""
            n366 = Concatenate Strings("cmd /c", w797, w798, w797, "\r\n") -> (w803:string)
            n367 = Temporary Directory() -> (w800:path)
            n368 = call <vilib>:"System Exec.vi"("run minimized? (F)"=TRUE, "wait until completion? (T)"=FALSE, "error in (no error)"=w795, "working directory"=w800, "command line"=w803) -> ("error out"=w796:errorcluster)  [unwired: 3 in, 3 out]
            n369 = call "AMC Send Local Messages.vi"("error in (no error)"=w796, "Message Names"=string[] ["Close SubVI", "Exit"], "Message Queue in"=w805) -> ("error out"=w794:errorcluster)  [unwired: 7 in, 1 out]
          }
        }
      }
      frame "Load Patient Register" {
        n370 = Unbundle By Name(w816) -> ("cRef.Profile.References.ListboxOperator"=w812:refnum<vi>, "cRef.Profile.References.ListboxDoctor"=w811:refnum<vi>, "cRef.Profile.References.Listbox Patient ID"=w815:refnum<vi>)
        n371 = call "ListboxItemsCpr(SubVI).vi"("error in (no error)"=w814, "LstBox Refnum"=w815) -> ("error out"=w809:errorcluster)  [unwired: 8 in, 1 out]
        n372 = call "AE Save.vi"("error in (no error)"=w809, "LstBox Refnum"=w811, "Action"=Enum_Save_Action_Events."Load Listbox") -> ("error out"=w810:errorcluster)  [unwired: 6 in, 1 out]
        n373 = call "AE Save.vi"("error in (no error)"=w810, "LstBox Refnum"=w812, "Action"=Enum_Save_Action_Events."Load Listbox") -> ("error out"=w807:errorcluster)  [unwired: 6 in, 1 out]
      }
      frame "Load Menu" {
        n374 = control-ref of="This VI"() -> (w823:refnum<vi>)
        n375 = Current VI's Path() -> (path=w825:path)
        n376 = Strip Path(path=w825) -> (stripped path=w821:path)  [unwired: 1 out]
        n377 = Build Path(base path=w821, name or relative path="DM2000RuntimeMenu.rtm") -> (appended path=w822:path)
        n378 = property class="VI"(reference=w823, error in=w820, "RT Menu Path"=w822) -> (reference out=w819:refnum<vi>, error out=w818:errorcluster)
        n379 = Close Reference(reference=w819, error in (no error)=w818) -> (error out=w817:errorcluster)
      }
      frame "/****Profile Page***/" {
      }
      frame "KeyDown" {
        n380 = Unbundle By Name(w830) -> ("System Parameters.Active Page"=w829:string)
        n381 = case shown="\"Left\"" w831 {
          tunnel: w832 -> [_ w835 w844 w853]
          tunnel: w829 -> [_ w834 w845 w852]
          frame "0", Default {
          }
          frame "Right" {
            # "Rightarrow"
            n382 = case shown="\"Configuration\"" w834 {
              tunnel: w835 -> [_ w836 w838 w840 w842]
              frame "Profile", Default {
              }
              frame "Configuration" {
                n383 = call "AMC Send Local Messages.vi"("Message Names"=string[] ["Subpanel: Load Acquisition"], "Message Queue in"=w836) -> ()  [unwired: 8 in, 2 out]
              }
              frame "Acquisition" {
                n384 = call "AMC Send Local Messages.vi"("Message Names"=string[] ["Subpanel: Load Data"], "Message Queue in"=w838) -> ()  [unwired: 8 in, 2 out]
              }
              frame "Data" {
                n385 = call "AMC Send Local Messages.vi"("Message Names"=string[] ["Subpanel: Load Journal"], "Message Queue in"=w840) -> ()  [unwired: 8 in, 2 out]
              }
              frame "Journal" {
                n386 = call "AMC Send Local Messages.vi"("Message Names"=string[] ["Subpanel: Load Profile"], "Message Queue in"=w842) -> ()  [unwired: 8 in, 2 out]
              }
            }
          }
          frame "Left" {
            # "Leftarrow"
            n387 = case shown="\"Journal\"" w845 {
              tunnel: w844 -> [_ _ w846 w848 w850]
              frame "Profile", Default {
              }
              frame "Configuration" {
              }
              frame "Acquisition" {
                n388 = call "AMC Send Local Messages.vi"("Message Names"=string[] ["Subpanel: Load Configuration"], "Message Queue in"=w846) -> ()  [unwired: 8 in, 2 out]
              }
              frame "Data" {
                n389 = call "AMC Send Local Messages.vi"("Message Names"=string[] ["Subpanel: Load Acquisition"], "Message Queue in"=w848) -> ()  [unwired: 8 in, 2 out]
              }
              frame "Journal" {
                n390 = call "AMC Send Local Messages.vi"("Message Names"=string[] ["Subpanel: Load Data"], "Message Queue in"=w850) -> ()  [unwired: 8 in, 2 out]
              }
            }
          }
          frame "Space" {
            # "Space"
            n391 = case shown="\"Configuration\"" w852 {
              tunnel: w853 -> [_ w855 w857 w858 _]
              frame "Profile", Default {
              }
              frame "Configuration" {
                n392 = call "AMC Send Local Messages.vi"("Message Names"=string[] ["Subpanel: Load Acquisition"], "Message Queue in"=w855) -> ()  [unwired: 8 in, 2 out]
              }
              frame "Acquisition" {
                n393 = call "AMC Send Local Message.vi"("Message Name"="Subpanel: Load Data", "Message Queue in"=w857) -> ()  [unwired: 8 in, 2 out]
              }
              frame "Data" {
                n394 = call "AMC Send Local Message.vi"("Message Name"="Subpanel: Load Configuration", "Message Queue in"=w858) -> ()  [unwired: 8 in, 2 out]
              }
              frame "Journal" {
              }
            }
          }
        }
      }
      frame "MWL: QueryWorklist" {
        n395 = call "fo_MWLQuery.vi"("error in (no error)"=w867) -> ("error out"=w864:errorcluster, "Cancel?"=w862:bool, "Worklist"=w866:string[][], "SelectedRow"=w865:string[])  [unwired: 7 in]
        n396 = case shown="False" w862 {
          tunnel: [w879 w882] -> w868
          tunnel: w860 -> [w876 w882]
          tunnel: w866 -> [w875 _]
          tunnel: w865 -> [w874 _]
          tunnel: w864 -> [w872 w881]
          tunnel: [w871 w881] -> w863
          tunnel: w861 -> [_ w880]
          frame False {
            n397 = global read "DataPathGlobalVariable.vi" "Current Measurement ID"() -> (w869:string)
            n398 = call "fo_LocatePatientInfo.vi"("subarray"=w874) -> ("PatientId"=w873:string, "PatientName"=w878:string)  [unwired: 9 in]
            n399 = call "CreateDicomPath.vi"("error in (no error)"=w872, "Measurement ID"=w869, "patientID"=w873) -> ("error out"=w871:errorcluster, "Path"=w870:path)  [unwired: 6 in, 1 out]
            n400 = call "DICOMFormatToName.vi"("DICOM Format Name"=w878) -> ("Name"=w877:string)  [unwired: 10 in]
            n401 = Bundle By Name(cluster=w876, "MWL.Name"=w877, "MWL.PatientID"=w873, "MWL.DICOM Variables"=w874, "MWL.Worklist"=w875, "MWL.DICOM Info"=w870, "System Parameters.Date"=w869) -> (w879:T3)
          }
          frame True {
            n402 = call "AMC Flush Message Queue.vi"("Message Queue in"=w880) -> ()  [unwired: 8 in, 2 out]
          }
        }
      }
      frame "MWL: PatientID" {
        # "This will put patientID into the listbox and\nthen select that patientID"
        n403 = Unbundle By Name(w888) -> ("cRef.Profile.References.Listbox Patient ID"=w883:refnum<vi>, "MWL.PatientID"=w885:string)
        n404 = Empty String/Path?(string/path=w885) -> (empty?=w884:bool)
        n405 = case shown="False" w884 {
          tunnel: w887 -> [w899 w909]
          tunnel: [w897 w909] -> w886
          tunnel: w885 -> [w893 _]
          tunnel: w883 -> [w889 _]
          frame False {
            # "Already exist?"
            n406 = property class="LstBox (strict)"(reference=w889) -> (reference out=w890:refnum<vi>, "Item Names"=w894:string[])  [unwired: 1 in, 1 out]
            n407 = Search 1D Array(1D array=w894, element=w893) -> (index of element=w892:i32)  [unwired: 1 in]
            n408 = Greater Or Equal To 0?(x=w892) -> (x >= 0?=w891:bool)
            n409 = case shown="False" w891 {
              tunnel: w893 -> [w905 w907]
              tunnel: w899 -> [w900 w908]
              tunnel: [w904 w908] -> w898
              tunnel: [w903 w906] -> w896
              tunnel: [w902 w907] -> w895
              tunnel: w890 -> [w901 w906]
              frame False {
                n410 = call "InsertPatientIDIntoList.vi"("error in (no error)"=w900, "CPR Number"=w905, "ListBox in"=w901) -> ("error out"=w904:errorcluster, "CPR Number Out"=w902:string, "ListBox out"=w903:refnum<vi>)  [unwired: 6 in]
              }
              frame True {
              }
            }
            n411 = call "FocusItemInListbox.vi"("error in (no error)"=w898, "patientID"=w895, "ListBox in"=w896) -> ("error out"=w897:errorcluster)  [unwired: 8 in]
          }
          frame True {
          }
        }
      }
      frame "MWL: Update Data" {
        n412 = Unbundle By Name(w913) -> ("MWL.PatientID"=w910:string, "cRef.Profile.References.Name"=w911:refnum<vi>, "MWL.Name"=w914:string, "User Parameters.Name"=w915:string)  [unwired: 1 out]
        n413 = Empty String/Path?(string/path=w910) -> (empty?=w912:bool)
        n414 = case shown="False" w912 {
          tunnel: w915 -> [w920 _]
          tunnel: w914 -> [w919 _]
          tunnel: w911 -> [w917 _]
          frame False {
            n415 = Empty String/Path?(string/path=w920) -> (empty?=w918:bool)
            n416 = case shown="True" w918 {
              tunnel: w919 -> [_ w921]
              tunnel: w917 -> [_ w922]
              frame False {
              }
              frame True {
                n417 = property class="Str"(reference=w922, "Val(Sgnl)"=w921) -> ()  [unwired: 1 in, 2 out]
              }
            }
          }
          frame True {
          }
        }
      }
      frame "DCM: Create Export Path" {
        # "patient id and date"
        # "Search existing journal"
        n418 = Unbundle By Name(w939) -> ("User Parameters.CPR Number"=w935:string, "Database.ActiveItemTag"=w926:string)
        n419 = global read "DataPathGlobalVariable.vi" "DataPath"() -> (w944:path)
        n420 = global read "DataPathGlobalVariable.vi" "ReportPath"() -> (w934:path)
        n421 = call "Encrypt.vi"("Input"=w935) -> ("Output"=w940:string)  [unwired: 10 in]
        n422 = String To Path(string=w926) -> (path=w925:path)
        n423 = Strip Path(path=w925) -> (name=w924:string)  [unwired: 1 out]
        n424 = Build Path(base path=w944, name or relative path=w940) -> (appended path=w941:path)
        n425 = call <vilib>:"Space Constant.vi"() -> ("String"=w936:string)
        n426 = List Folder(path=w934, error in=w927) -> (filenames=w931:string[], error out=w923:errorcluster)  [unwired: 2 in, 2 out]
        n427 = Build Path(base path=w941, name or relative path=w924) -> (appended path=w943:path)
        n428 = Concatenate Strings(w935, w936, w924) -> (w933:string)
        n429 = Build Path(base path=w943, name or relative path="info.dcm") -> (appended path=w937:path)
        n430 = while {
          tunnel: w931 -> [w953] mode=indexing
          tunnel: w933 -> [w956]
          tunnel: [w953] -> w932
          tunnel: w931 -> [w952]
          tunnel: [w947] -> w928
          i -> [w951]
          stop <- w949 stop-if-true
          n431 = Array Size(array=w952) -> (size(s)=w950:i32)
          n432 = xnode "Match Regular Expression"("input string"=w953, "regular expression"=w956) -> ("offset past match"=w955:i32)  [unwired: 4 in, 4 out]
          n433 = Less?(x=w950, y=w951) -> (x < y?=w947:bool)
          n434 = Greater?(x=w955, y=0) -> (0:w948:bool)
          n435 = Or(x=w948, y=w947) -> (x .or. y?=w949:bool)
        }
        n436 = Build Path(base path=w934, name or relative path=w932) -> (appended path=w930:path)
        n437 = case shown="False" w928 {
          tunnel: [w945 path "" ("appended path")] -> w929
          tunnel: w930 -> [w945 _]
          frame False {
          }
          frame True {
          }
        }
        n438 = Bundle By Name(cluster=w939, "Database.JournalPath"=w929, "MWL.DICOM Info"=w937) -> (w938:T3)
      }
      frame "DCM: Export Journal" {
        n439 = Unbundle By Name(w1074) -> ("Database.JournalPath"=w1072:path, "MWL.DICOM Info"=w1073:path)
        n440 = Empty String/Path?(string/path=w1072) -> (empty?=w1071:bool)
        n441 = call-poly <userlib>:"File Exists__ogtk.vi"("file path"=w1073) -> ("exists"=w1068:bool)  [unwired: 6 in, 1 out]
        n442 = Not(x=w1071) -> (.not. x?=w1070:bool)
        n443 = And(x=w1070, y=w1068) -> (x .and. y?=w1069:bool)
        n444 = case shown="True" w1069 {
          tunnel: w1076 -> [w1078 w1092]
          tunnel: [w1078 w1091] -> w1075
          tunnel: w1072 -> [_ w1082]
          tunnel: w1073 -> [_ w1081]
          frame False {
            n445 = One Button Dialog(message="To generate a DICOM file it is neccessary to acquire study information from the Worklist beforehand or generate DICOM values manually. It is also neccessary to generate a journal beforehand by using the button to the left.") -> ()  [unwired: 1 in, 1 out]
          }
          frame True {
            n446 = Unbundle By Name(T18 {"HospInfo"={"Name"="", "Address"="", "Department"=""}, "Pressure"={"Pressure"=0.0}, "DataPath"={"DataPath"=path ""}, "ReportPath"={"Path"=path "", "Name"=""}, "DICOM Info WL"={"port"=0, "AEtitle"="", "host"="", "remoteAE"=""}, "DICOM Info PACS"={"port"=0, "AEtitle"="", "host"="", "remoteAE"=""}, "ArmCalcMethod"=0.0, "itemTags"=[], "DicomEncoding"=0, "JournalType"=0, "General Settings"={"Hyphenation"=FALSE, "Language"=0, "CellStr1"="", "CellStr2"=""}, "Dicom Tags"=[], "BT Serial"=[], "BT License"={"License"="", "Accepted Serials"=[]}} ("Data")) -> ("DICOM Info PACS"=w1093:T25)
            n447 = call "AE Save.vi"("error in (no error)"=w1092, "Action"=Enum_Save_Action_Events."LoadDICOMInfoPACS") -> ("error out"=w1096:errorcluster, "Anything"=w1095:variant)  [unwired: 7 in]
            n448 = Variant To Data(error in=w1096, type=w1093, Variant=w1095) -> (data=w1090:T25, error out=w1089:errorcluster)
            n449 = call <vilib>:"Set Busy.vi"("error in (no error)"=w1089) -> ("error out"=w1088:errorcluster)  [unwired: 9 in, 1 out]
            n450 = call "fo_ExcelToDcm.vi"("DICOM Info"=w1081, "error in (no error)"=w1088, "JournalPath"=w1082, "ServerInfo"=w1090) -> ("error out"=w1085:errorcluster, "No active excel error"=w1080:bool)  [unwired: 6 in]
            n451 = call-poly <userlib>:"MGI Suppress Error Code.vi"("Error Code"=51000, "Error In"=w1085) -> ("Error Supressed?"=w1083:bool, "Error Out"=w1086:errorcluster)  [unwired: 4 in]
            n452 = call <vilib>:"Unset Busy.vi"("error in (no error)"=w1086) -> ("error out"=w1087:errorcluster)  [unwired: 10 in]
            n453 = case shown="True" w1080 {
              tunnel: w1087 -> [w1099 w1100]
              tunnel: [w1099 w1100] -> w1091
              frame False {
              }
              frame True {
                n454 = One Button Dialog(message="Cannot connect to Excel. Please make sure that Excel is running. ") -> ()  [unwired: 1 in, 1 out]
              }
            }
            n455 = case shown="True" w1083 {
              tunnel: "Some error: 51000" ("VerificationFailure") -> [_ w1098]
              frame False {
              }
              frame True {
                n456 = One Button Dialog(message=w1098) -> ()  [unwired: 1 in, 1 out]
              }
            }
          }
        }
      }
      frame "DCM: Load DICOM Info" {
        n457 = Unbundle By Name(w1103) -> ("MWL.DICOM Info"=w1102:path)
        n458 = call-poly <userlib>:"File Exists__ogtk.vi"("file path"=w1102) -> ("exists"=w1106:bool)  [unwired: 6 in, 1 out]
        n459 = Empty String/Path?(string/path=w1102) -> (empty?=w1105:bool)
        n460 = Implies(1:w1105, 2:w1106) -> (0:w1104:bool)
        n461 = case shown="False" w1104 {
          tunnel: w1103 -> [w1116 w1120]
          tunnel: [w1115 w1119] -> w1109
          tunnel: w1102 -> [w1114 w1117]
          tunnel: w1108 -> [w1112 w1121]
          tunnel: [w1111 w1121] -> w1107
          frame False {
            n462 = Path To String(path=w1114) -> (string=w1113:string)
            n463 = call "fo_DumpDataset.vi"("error in (no error)"=w1112, "file"=w1113) -> ("error out"=w1111:errorcluster, "items"=w1110:string[])  [unwired: 6 in, 2 out]
            n464 = Bundle By Name(cluster=w1116, "MWL.DICOM Info"=w1114, "MWL.DICOM Variables"=w1110) -> (w1115:T3)
          }
          frame True {
            n465 = Bundle By Name(cluster=w1120, "MWL.DICOM Info"=w1117, "MWL.DICOM Variables"=string[] []) -> (w1119:T3)
          }
        }
      }
      frame "DCM: Show Values" {
        n466 = Unbundle By Name(w1126) -> ("MWL.DICOM Info"=w1123:path)
        n467 = call-poly <userlib>:"File Exists__ogtk.vi"("file path"=w1123) -> ("exists"=w1122:bool)  [unwired: 6 in, 1 out]
        n468 = case shown="True" w1122 {
          tunnel: w1125 -> [w1128 w1135]
          tunnel: [w1128 w1137] -> w1124
          tunnel: w1123 -> [_ w1136]
          frame False {
            n469 = One Button Dialog(message="No DICOM files found") -> ()  [unwired: 1 in, 1 out]
          }
          frame True {
            n470 = Path To String(path=w1136) -> (string=w1133:string)
            n471 = call "fo_DumpDataset.vi"("error in (no error)"=w1135, "file"=w1133) -> ("error out"=w1134:errorcluster, "items"=w1130:string[], "keywords"=w1131:string[], "tags"=w1132:string[])  [unwired: 6 in]
            n472 = Build Array(w1132, w1131, w1130) -> (w1129:string[][])
            n473 = call "ShowDicomValues.vi"("error in (no error)"=w1134, "Array"=w1129) -> ("error out"=w1137:errorcluster)  [unwired: 9 in]
          }
        }
      }
      frame "DCM: Update Variables" {
        n474 = Unbundle By Name(w1144) -> ("MWL.DICOM Variables"=w1138:string[], "User Parameters.Name"=w1142:string, "User Parameters.CPR Number"=w1141:string, "User Parameters.Operator"=w1139:string)
        n475 = call "InputDICOMVariables.vi"("values"=w1138, "Operator"=w1139, "CPR Number"=w1141, "Name"=w1142) -> ("Array"=w1140:string[])  [unwired: 7 in]
        n476 = Bundle By Name(cluster=w1144, "MWL.DICOM Variables"=w1140) -> (w1143:T3)
      }
      frame "LoadNameCpr" {
        n477 = Unbundle By Name(w1156) -> ("cRef.Profile.References"=w1154:T26, "cRef.Profile.References.Listbox Patient ID"=w1155:refnum<vi>, "System Parameters.Date"=w1147:string)
        n478 = property class="LstBox (strict)"(reference=w1155, error in=w1166) -> (error out=w1158:errorcluster, "Item Names"=w1169:string[], "Value"=w1168:i32)  [unwired: 1 out]
        n479 = Index Array(array=w1169, index=w1168) -> (element=w1159:string)
        n480 = global read "DataPathGlobalVariable.vi" "DataPath"() -> (w1167:path)
        n481 = call "Encrypt.vi"("Input"=w1159) -> ("Output"=w1160:string)  [unwired: 10 in]
        n482 = Build Path(base path=w1167, name or relative path=w1160) -> (appended path=w1148:path)
        n483 = Build Path(base path=w1148, name or relative path=w1147) -> (appended path=w1146:path)
        n484 = global write "DataPathGlobalVariable.vi" "DataPatientDatePath"(w1146) -> ()
        n485 = global write "DataPathGlobalVariable.vi" "DataPatientPath"(w1148) -> ()
        n486 = Unbundle By Name(w1154) -> ("Name"=w1153:refnum<vi>, "ListboxOperator"=w1152:refnum<vi>, "ListboxDoctor"=w1151:refnum<vi>, "CommentStr"=w1150:refnum<vi>)
        n487 = call "LoadProfileInfo.vi"("error in (no error)"=w1158, "DataPatientPath"=w1148) -> ("error out"=w1157:errorcluster, "Doctor"=w1162:string, "Operator"=w1163:string, "Name"=w1164:string, "Comment"=w1161:string)  [unwired: 5 in]
        n488 = Bundle("Name"=w1153, "ListboxOperator"=w1152, "ListboxDoctor"=w1151, "CommentStr"=w1150, "Name"=w1164, "Operator"=w1163, "Doctor"=w1162, "Comment"=w1161) -> (w1149:T27)  [unwired: 1 in]
        n489 = call "UpdateProfile.vi"("error in"=w1157, "cluster"=w1149) -> ("error out"=w1165:errorcluster)  [unwired: 5 in]
      }
      frame "Load Armpressure" {
        n490 = Unbundle By Name(w1176) -> ("Configuration.Queue"=w1175:refnum<queue>)
        n491 = Bundle By Name(cluster=cluster{"Msg":string, "Data":variant} {"Msg"="", "Data"=variant} ("element"), "Msg"="Load Arm Pressure") -> (w1172:cluster{"Msg":string, "Data":variant})
        n492 = Enqueue Element(queue=w1175, element=w1172, error in (no error)=w1174) -> (error out=w1173:errorcluster)  [unwired: 1 in, 2 out]
      }
      frame "AddCpr" {
        n493 = Unbundle By Name(w1178) -> ("cRef.Profile.References.Listbox Patient ID"=w1177:refnum<vi>)
        n494 = call "TypeCPRNum(SubVI).vi"() -> ("CprOut"=w1180:string, "Boolean"=w1181:bool)  [unwired: 2 in]
        n495 = property class="LstBox (strict)"(reference=w1177, error in=w1184) -> (reference out=w1179:refnum<vi>, error out=w1183:errorcluster, "Item Names"=w1185:string[])
        n496 = case shown="False" w1181 {
          tunnel: w1185 -> [w1200 _]
          tunnel: w1179 -> [w1199 _]
          tunnel: w1183 -> [w1194 w1203]
          tunnel: w1180 -> [w1187 _]
          tunnel: [w1197 w1203] -> w1182
          frame False {
            w1192 = 10 items=["No error", "Argument error", "Memory is full", "Out of zone", "End of file", "File already open", "Generic file I/O error", "File not found", "File permission error", "Disk is full", "Duplicate path", "Too many files open", "System feature not enabled", "Resource file not found", "Cannot add resource", "Resource not found", "Image not found", "Image memory error", "Pen does not exist", "Config type invalid", "Config token not found", "Config parse error", "Config memory error", "Bad external code format", "Bad external code offset", "External code not present", "Null window", "Destroy window error", "Null menu", "Print aborted", "Bad print record", "Print driver error", "Windows error during printing", "Memory error during printing", "Print dialog error", "Generic print error", "Invalid device refnum", "Device not found", "Device parameter error", "Device unit error", "Cannot open device", "Device call aborted", "Generic error", "Cancelled by user", "Object ID too low", "Object ID too high", "Object not in heap", "Unknown heap", "Unknown object (invalid DefProc)", "Unknown object (DefProc not in table)", "Message out of range", "Invalid (null) method", "Unknown message", "Manager call not supported", "Bad address", "Network operation in progress", "Network operation timed out", "Connection is busy", "Network attribute not supported", "Network error", "Address in use", "System out of memory", "Connection aborted", "Connection refused", "Not connected", "Already connected", "Connection closed", "Initialization error (interapplication manager)", "Bad occurrence", "Wait on unbound occurrence handler", "Occurrence queue overflow", "Datalog type conflict", "Unused", "Unrecognized type (interapplication manager)", "Memory corrupt", "Failed to make temporary DLL", "Old CIN version", "Drag socket not found", "Failed to load drop-object", "Failed to register OLE object", "Failed to release OLE object", "Format specifier type mismatch", "Unknown format specifier", "Too few format specifiers", "Too many format specifiers", "Scan failed", "Newer CIN version", "OLE Convert", "Runtime menu error", "Password tampered", "Unknown error code"] ("Error Code")
            # "If CPR number exists, suppress error\nand display message"
            # "Create new folder"
            n497 = global read "DataPathGlobalVariable.vi" "DataPath"() -> (w1198:path)
            n498 = Insert Into Array(array=w1200, index=0, new element=w1187) -> (w1190:string[])
            n499 = call "Encrypt.vi"("Input"=w1187) -> ("Output"=w1186:string)  [unwired: 10 in]
            n500 = Build Path(base path=w1198, name or relative path=w1186) -> (appended path=w1193:path)
            n501 = Create Folder(path (use dialog)=w1193, error in=w1194) -> (error out=w1195:errorcluster)  [unwired: 1 in, 2 out]
            n502 = property class="LstBox (strict)"(reference=w1199, error in=w1195, "Item Names"=w1190, "Val(Sgnl)"=0 ("Value (Signaling)")) -> (error out=w1196:errorcluster)  [unwired: 1 out]
            n503 = call-poly <userlib>:"MGI Suppress Error Code.vi"("Error Code"=w1192, "Error In"=w1196) -> ("Error Supressed?"=w1191:bool, "Error Out"=w1197:errorcluster)  [unwired: 4 in]
            n504 = case shown="True" w1191 {
              frame False {
              }
              frame True {
                n505 = One Button Dialog(message="The CPR number already exists", button name ("OK")="Close") -> ()  [unwired: 1 out]
              }
            }
          }
          frame True {
            # "Cancel true?"
          }
        }
      }
      frame "EditHospInfo" {
        n506 = Unbundle By Name(w1205) -> ("Profile.Queue"=w1204:refnum<queue>)
        n507 = call "SaveHospInfo.vi"() -> ("Cancel?"=w1208:bool, "Department 2"=w1209:string, "Hospital Address 2"=w1210:string, "Hospital Name 2"=w1211:string)  [unwired: 8 in]
        n508 = case shown="False" w1208 {
          tunnel: w1211 -> [w1222 _]
          tunnel: w1210 -> [w1221 _]
          tunnel: w1209 -> [w1220 _]
          tunnel: [w1216 w1224] -> w1207
          tunnel: w1206 -> [w1218 w1224]
          tunnel: w1204 -> [w1215 _]
          frame False {
            n509 = Bundle("Hospital Name 2"=w1222, "Hospital Address 2"=w1221, "Department 2"=w1220) -> (w1219:T28)  [unwired: 1 in]
            n510 = To Variant(anything=w1219) -> (Variant=w1213:variant)
            n511 = call "AE Save.vi"("error in (no error)"=w1218, "Variant In"=w1213, "Action"=Enum_Save_Action_Events."SaveHospInfo") -> ("error out"=w1217:errorcluster)  [unwired: 6 in, 1 out]
            n512 = Bundle By Name(cluster=cluster{"Msg":string, "Data":variant} {"Msg"="Load Hospital Info", "Data"=variant} ("element"), "Data"=w1213) -> (w1212:cluster{"Msg":string, "Data":variant})
            n513 = Enqueue Element(queue=w1215, element=w1212, error in (no error)=w1217) -> (error out=w1216:errorcluster)  [unwired: 1 in, 2 out]
          }
          frame True {
          }
        }
      }
      frame "Load Hospital Info" {
        n514 = Unbundle By Name(w1229) -> ("Profile.Queue"=w1228:refnum<queue>)
        n515 = Enqueue Element(queue=w1228, element=cluster{"Msg":string, "Data":variant} {"Msg"="Load Hospital Info", "Data"=variant}, error in (no error)=w1226) -> (error out=w1225:errorcluster)  [unwired: 1 in, 2 out]
      }
      frame "RemoveCpr" {
        n516 = global read "DataPathGlobalVariable.vi" "DataPath"() -> (w1237:path)
        n517 = Unbundle By Name(w1231) -> ("cRef.Profile.References.Listbox Patient ID"=w1230:refnum<vi>)
        n518 = call "Encrypt.vi"("Input"=w1236) -> ("Output"=w1238:string)  [unwired: 10 in]
        n519 = Build Path(base path=w1237, name or relative path=w1238) -> (appended path=w1232:path)
        n520 = call-poly <userlib>:"File Exists__ogtk.vi"("file path"=w1232) -> ("is directory"=w1234:bool, "exists"=w1233:bool)  [unwired: 6 in]
        n521 = And(x=w1234, y=w1233) -> (x .and. y?=w1235:bool)
        n522 = case shown="True" w1235 {
          tunnel: [w1243 w1250] -> w1242
          tunnel: w1241 -> [w1243 w1249]
          tunnel: [w1244 w1248] -> w1239
          tunnel: w1236 -> [w1244 w1246]
          tunnel: w1232 -> [_ w1247]
          tunnel: w1230 -> [_ w1245]
          frame False {
          }
          frame True {
            n523 = Concatenate Strings("Do you want to delete patient ID: " ("message"), w1246, " and all the data in the folder?" ("string")) -> (w1253:string)
            n524 = Two Button Dialog(message=w1253, 1:"Cancel" ("F button name (\"Cancel\")"), 2:"Yes" ("T button name (\"OK\")")) -> (T button?=w1256:bool)
            n525 = case shown="True" w1256 {
              tunnel: [w1258 w1263] -> w1250
              tunnel: w1249 -> [w1258 w1262]
              tunnel: [w1257 w1261] -> w1248
              tunnel: w1247 -> [_ w1260]
              tunnel: w1246 -> [w1257 _]
              tunnel: w1245 -> [_ w1259]
              frame False {
              }
              frame True {
                n526 = while {
                  tunnel: [w1269] -> w1264
                  tunnel: w1262 -> [w1268]
                  tunnel: w1260 -> [w1267]
                  stop <- w1265 continue-if-true
                  n527 = Delete(path (use dialog)=w1267, entire hierarchy (F)=TRUE, error in=w1268) -> (deleted path=w1266:path, error out=w1269:errorcluster)  [unwired: 2 in, 1 out]
                  n528 = call-poly <userlib>:"File Exists__ogtk.vi"("file path"=w1266) -> ("exists"=w1265:bool)  [unwired: 6 in, 1 out]
                }
                n529 = call "ListboxItemsCpr(SubVI).vi"("error in (no error)"=w1264, "LstBox Refnum"=w1259) -> ("error out"=w1263:errorcluster, "FirstCpr"=w1261:string)  [unwired: 8 in]
              }
            }
          }
        }
        n530 = Bundle By Name(cluster=w1231, "User Parameters.CPR Number"=w1239) -> (w1240:T3)
      }
      frame "SelectCpr" {
        n531 = Unbundle By Name(w1273) -> ("User Parameters.Name"=w1289:string, "User Parameters.CPR Number"=w1275:string, "cRef.Menu.References.PersonalInfoString"=w1287:refnum<vi>, "System Parameters.Date"=w1274:string, "cRef.Data.References.Menu"=w1283:refnum<vi>, "cRef.Journal.References.Data"=w1282:refnum<vi>, "cRef.Journal.References.Menu"=w1281:refnum<vi>)
        n532 = call "SelectCprRutine.vi"("CPR Number"=w1275, "error in"=w1285, "Journal Menu"=w1281, "Data Listbox"=w1282, "ProcessDataTreeMenu"=w1283) -> ("error out"=w1284:errorcluster)  [unwired: 5 in]
        n533 = global read "DataPathGlobalVariable.vi" "DataPath"() -> (w1280:path)
        n534 = Concatenate Strings(w1289, "\r", w1275) -> (w1286:string)
        n535 = call "Encrypt.vi"("Input"=w1275) -> ("Output"=w1279:string)  [unwired: 10 in]
        n536 = property class="Str"(reference=w1287, "Value"=w1286) -> ()  [unwired: 1 in, 2 out]
        n537 = Build Path(base path=w1280, name or relative path=w1279) -> (appended path=w1278:path)
        n538 = Build Path(base path=w1278, name or relative path=w1274) -> (appended path=w1277:path)
        n539 = Build Path(base path=w1277, name or relative path="info.dcm") -> (appended path=w1271:path)
        n540 = Bundle By Name(cluster=w1273, "MWL.DICOM Info"=w1271) -> (w1272:T3)
      }
      frame "ResetToDefault" {
        n541 = Unbundle By Name(w1290) -> ("Configuration.Queue"=w1294:refnum<queue>, "Journal.Queue"=w1293:refnum<queue>, "Data.Queue"=w1292:refnum<queue>)
        n542 = Enqueue Element(queue=w1292, element=cluster{"Msg":string, "Data":variant} {"Msg"="ResetGraphs", "Data"=variant}, error in (no error)=w1297) -> (error out=w1295:errorcluster)  [unwired: 1 in, 2 out]
        n543 = Build Array(w1294, w1293, w1292) -> (w1291:refnum<queue>[])
        n544 = for {
          tunnel: w1291 -> [w1299] mode=indexing
          n545 = Enqueue Element(queue=w1299, element=cluster{"Msg":string, "Data":variant} {"Msg"="Clear", "Data"=variant}) -> ()  [unwired: 2 in, 3 out]
        }
      }
      frame "Delete: ListboxDoctor" {
        n546 = Unbundle By Name(w1304) -> ("cRef.Profile.References.ListboxDoctor"=w1303:refnum<vi>)
        n547 = Decimal String To Number(string=w1302) -> (number=w1301:i32)  [unwired: 2 in, 1 out]
        n548 = property class="LstBox (strict)"(reference=w1303, error in=w1300) -> (reference out=w1309:refnum<vi>, error out=w1308:errorcluster, "Item Names"=w1311:string[])
        n549 = Delete From Array(array=w1311, index=w1301) -> (array with subset deleted=w1310:string[])  [unwired: 1 in, 1 out]
        n550 = property class="LstBox (strict)"(reference=w1309, error in=w1308, "Item Names"=w1310) -> (reference out=w1305:refnum<vi>, error out=w1307:errorcluster)
        n551 = call "AE Save.vi"("error in (no error)"=w1307, "LstBox Refnum"=w1305, "Action"=Enum_Save_Action_Events."Save Listbox") -> ("error out"=w1312:errorcluster)  [unwired: 6 in, 1 out]
      }
      frame "Delete: ListboxOperator" {
        n552 = Unbundle By Name(w1317) -> ("cRef.Profile.References.ListboxOperator"=w1316:refnum<vi>)
        n553 = Decimal String To Number(string=w1315) -> (number=w1314:i32)  [unwired: 2 in, 1 out]
        n554 = property class="LstBox (strict)"(reference=w1316, error in=w1313) -> (reference out=w1322:refnum<vi>, error out=w1321:errorcluster, "Item Names"=w1324:string[])
        n555 = Delete From Array(array=w1324, index=w1314) -> (array with subset deleted=w1323:string[])  [unwired: 1 in, 1 out]
        n556 = property class="LstBox (strict)"(reference=w1322, error in=w1321, "Item Names"=w1323) -> (reference out=w1318:refnum<vi>, error out=w1320:errorcluster)
        n557 = call "AE Save.vi"("error in (no error)"=w1320, "LstBox Refnum"=w1318, "Action"=Enum_Save_Action_Events."Save Listbox") -> ("error out"=w1325:errorcluster)  [unwired: 6 in, 1 out]
      }
      frame "Add New: ListboxDoctor" {
        n558 = Unbundle By Name(w1327) -> ("cRef.Profile.References.ListboxDoctor"=w1326:refnum<vi>)
        n559 = call "AddName.vi"() -> ("Cancel Indicator"=w1330:bool, "NameString"=w1331:string)  [unwired: 9 in]
        n560 = case shown="False" w1330 {
          tunnel: w1331 -> [w1340 _]
          tunnel: w1329 -> [w1334 w1343]
          tunnel: [w1333 w1343] -> w1328
          tunnel: w1326 -> [w1332 _]
          frame False {
            n561 = property class="LstBox (strict)"(reference=w1332, error in=w1334) -> (reference out=w1342:refnum<vi>, error out=w1336:errorcluster, "Item Names"=w1339:string[])
            n562 = Insert Into Array(array=w1339, new element=w1340) -> (w1341:string[])  [unwired: 1 in]
            n563 = property class="LstBox (strict)"(reference=w1342, error in=w1336, "Item Names"=w1341) -> (reference out=w1337:refnum<vi>, error out=w1335:errorcluster)
            n564 = call "AE Save.vi"("error in (no error)"=w1335, "LstBox Refnum"=w1337, "Action"=Enum_Save_Action_Events."Save Listbox") -> ("error out"=w1333:errorcluster)  [unwired: 6 in, 1 out]
          }
          frame True {
          }
        }
      }
      frame "Add New: ListboxOperator" {
        n565 = Unbundle By Name(w1345) -> ("cRef.Profile.References.ListboxOperator"=w1344:refnum<vi>)
        n566 = call "AddName.vi"() -> ("Cancel Indicator"=w1348:bool, "NameString"=w1349:string)  [unwired: 9 in]
        n567 = case shown="False" w1348 {
          tunnel: w1349 -> [w1358 _]
          tunnel: w1347 -> [w1352 w1361]
          tunnel: [w1351 w1361] -> w1346
          tunnel: w1344 -> [w1350 _]
          frame False {
            n568 = property class="LstBox (strict)"(reference=w1350, error in=w1352) -> (reference out=w1360:refnum<vi>, error out=w1354:errorcluster, "Item Names"=w1357:string[])
            n569 = Insert Into Array(array=w1357, new element=w1358) -> (w1359:string[])  [unwired: 1 in]
            n570 = property class="LstBox (strict)"(reference=w1360, error in=w1354, "Item Names"=w1359) -> (reference out=w1355:refnum<vi>, error out=w1353:errorcluster)
            n571 = call "AE Save.vi"("error in (no error)"=w1353, "LstBox Refnum"=w1355, "Action"=Enum_Save_Action_Events."Save Listbox") -> ("error out"=w1351:errorcluster)  [unwired: 6 in, 1 out]
          }
          frame True {
          }
        }
      }
      frame "FindCprNumber" {
        # "Exclude non-match"
        # "Search for CPR number"
        n572 = Unbundle By Name(w1365) -> ("cRef.Profile.References.Listbox Patient ID"=w1364:refnum<vi>, "cRef.Profile.References.Search Patient ID"=w1363:refnum<vi>)
        n573 = global read "DataPathGlobalVariable.vi" "DataPath"() -> (w1378:path)
        n574 = property class="Str"(reference=w1363) -> ("Value"=w1362:string)  [unwired: 1 in, 2 out]
        n575 = call <userlib>:"List Directory__ogtk.vi"("directory path"=w1378) -> ("directory names"=w1377:string[])  [unwired: 3 in, 3 out]
        n576 = for {
          tunnel: w1377 -> [w1390] mode=indexing
          tunnel: [w1392] -> w1376 mode=indexing
          tunnel: [w1391] -> w1375 mode=indexing
          tunnel: w1362 -> [w1388]
          n577 = call "Decrypt.vi"("Input"=w1390) -> ("Output"=w1389:string)  [unwired: 10 in]
          n578 = String Subset(string=w1389) -> (substring=w1393:string)  [unwired: 2 in]
          n579 = Search/Split String(string=w1393, search string/char (-)=w1388) -> (match + rest of string=w1391:string, offset of match=w1392:i32)  [unwired: 1 in, 1 out]
        }
        n580 = for {
          tunnel: w1376 -> [w1382] mode=indexing
          tunnel: w1375 -> [w1380] mode=indexing
          shift-right: [w1379] -> w1371
          shift-left: string[] [] -> [w1383]
          n581 = Equal To 0?(x=w1382) -> (x = 0?=w1381:bool)
          n582 = case shown="True" w1381 {
            tunnel: [w1384 w1387] -> w1379
            tunnel: w1383 -> [w1384 w1386]
            tunnel: w1380 -> [_ w1385]
            frame False {
            }
            frame True {
              n583 = Build Array (concatenate)(w1386, w1385) -> (w1387:string[])
            }
          }
        }
        n584 = property class="LstBox (strict)"(reference=w1364, error in=w1366, "Item Names"=w1371) -> (reference out=w1372:refnum<vi>, error out=w1373:errorcluster)
        n585 = property class="LstBox (strict)"(reference=w1372, error in=w1373, "Value"=-1 ("Value (Signaling)")) -> (reference out=w1369:refnum<vi>, error out=w1368:errorcluster)
        n586 = Close Reference(reference=w1369, error in (no error)=w1368) -> (error out=w1367:errorcluster)
      }
      frame "/*** Configuration ***/" {
      }
      frame "InitNewTest" {
        n587 = Get Date/Time In Seconds() -> (seconds since 1Jan1904=w1400:timestamp)
        n588 = Format Date/Time String(time format string (%c)="%Y-%m-%d", seconds (now)=w1400) -> (date/time string=w1396:string)  [unwired: 1 in]
        n589 = Bundle By Name(cluster=w1398, "System Parameters.Date"=w1396) -> (w1397:T3)
        n590 = global write "DataPathGlobalVariable.vi" "Current Measurement ID"(w1396) -> ()
      }
      frame "Change Segment" {
        n591 = Unbundle By Name(w1410) -> ("cRef.Configuration.References.ListboxMeasurementArea"=w1409:refnum<vi>)
        n592 = property class="LstBox (strict)"(reference=w1409, error in=w1404) -> (reference out=w1408:refnum<vi>, error out=w1402:errorcluster, "Item Names"=w1407:string[])
        n593 = Match First String(2:w1407, 3:w1406) -> (0:w1405:i32)  [unwired: 1 out]
        n594 = property class="LstBox (strict)"(reference=w1408, error in=w1402, "Value"=w1405) -> (error out=w1403:errorcluster)  [unwired: 1 out]
      }
      frame "Set Height" {
        n595 = Unbundle By Name(w1415) -> ("cRef.Configuration.References.HeightAdjustmentInt"=w1416:refnum<vi>)
        n596 = property class="DigNum (strict)"(reference=w1416) -> ("Value"=w1413:dbl)  [unwired: 1 in, 2 out]
        n597 = Bundle By Name(cluster=w1415, "Database.Height Adjustment"=w1413) -> (w1414:T3)
        n598 = call "AE Variables.vi"("VariantIn"=w1413, "error in (no error)"=w1412, "Action"=Enum_Variables."Set Height") -> ("error out"=w1411:errorcluster)  [unwired: 9 in, 7 out]
      }
      frame "/******Acquisition******/" {
      }
      frame "Set Acquisition Mode" {
        n599 = call "AE Save.vi"("error in (no error)"=w1428, "Action"=Enum_Save_Action_Events."Load Acquisition Mode") -> ("error out"=w1427:errorcluster, "Anything"=w1424:variant)  [unwired: 7 in]
        n600 = Unbundle By Name(w1426) -> ("Acquisition.Queue"=w1433:refnum<queue>)
        n601 = Bundle By Name(cluster=cluster{"Msg":string, "Data":variant} {"Msg"="", "Data"=variant} ("element"), "Msg"="Set Mode", "Data"=w1424) -> (w1430:cluster{"Msg":string, "Data":variant})
        n602 = Enqueue Element(queue=w1433, element=w1430, error in (no error)=w1427) -> (error out=w1421:errorcluster)  [unwired: 1 in, 2 out]
        n603 = Variant To Data(error in=w1421, type=FALSE, Variant=w1424) -> (data=w1422:bool, error out=w1420:errorcluster)
        n604 = Bundle By Name(cluster=w1426, "Data Acquisition.Control?"=w1422) -> (w1425:T3)
      }
      frame "Query DAQ Availability" {
        n605 = Unbundle By Name(w1442) -> ("Acquisition.Queue"=w1434:refnum<queue>, "cRef.Menu.References.MenuStartADC"=w1439:refnum<vi>)
        n606 = call "availableDAQ.vi"("error in (no error)"=w1436) -> ("error out"=w1437:errorcluster, "DAQmx Device Name"=w1441:tag)  [unwired: 9 in]
        n607 = Empty String/Path?(string/path=w1441) -> (empty?=w1440:bool)
        n608 = case shown="False" w1440 {
          tunnel: w1439 -> [_ w1466]
          tunnel: w1438 -> [w1446 w1464]
          tunnel: w1437 -> [w1445 w1463]
          tunnel: [w1444 w1462] -> w1435
          tunnel: w1434 -> [w1443 _]
          frame False {
            n609 = call "AE Variables.vi"("error in (no error)"=w1445, "Action"=Enum_Variables."Get DAQ Connected") -> ("BooleanOut"=w1447:bool, "error out"=w1449:errorcluster)  [unwired: 10 in, 6 out]
            n610 = case shown="False" w1447 {
              tunnel: [w1450 w1459] -> w1444
              tunnel: w1449 -> [w1451 w1460]
              tunnel: w1446 -> [w1452 w1461]
              tunnel: w1443 -> [w1457 _]
              frame False {
                n611 = Enqueue Element(queue=w1457, element=cluster{"Msg":string, "Data":variant} {"Msg"="Initialize DAQ", "Data"=variant}, error in (no error)=w1451) -> (error out=w1455:errorcluster)  [unwired: 1 in, 2 out]
                n612 = call "AE Variables.vi"("VariantIn"=TRUE, "error in (no error)"=w1455, "Action"=Enum_Variables."Set DAQ Connected") -> ("error out"=w1450:errorcluster)  [unwired: 9 in, 7 out]
                n613 = call "AMC Send Local Messages.vi"("Message Names"=string[] ["Initialize Reference", "Monitor Reference", "Update Display"], "Message Queue in"=w1452) -> ()  [unwired: 8 in, 2 out]
              }
              frame True {
                # "If DAQ is already active\nignore commands"
                n614 = call "AMC Flush Message Queue.vi"("error in (no error)"=w1460, "Message Queue in"=w1461) -> ("error out"=w1459:errorcluster)  [unwired: 7 in, 1 out]
              }
            }
          }
          frame True {
            n615 = call "AMC Flush Message Queue.vi"("Message Queue in"=w1464) -> ()  [unwired: 8 in, 2 out]
            n616 = property class="Bool (strict)"(reference=w1466, error in=w1463, "Value"=FALSE) -> (error out=w1462:errorcluster)  [unwired: 1 out]
            n617 = One Button Dialog(message="The USB interface cannot be registered. Please connect") -> ()  [unwired: 1 in, 1 out]
          }
        }
      }
      frame "Silent DAQ Initialization" {
        n618 = Unbundle By Name(w1476) -> ("Acquisition.Queue"=w1469:refnum<queue>, "cRef.Menu.References.MenuStartADC"=w1468:refnum<vi>)
        n619 = call "availableDAQ.vi"("error in (no error)"=w1471) -> ("error out"=w1472:errorcluster, "DAQmx Device Name"=w1475:tag)  [unwired: 9 in]
        n620 = Empty String/Path?(string/path=w1475) -> (empty?=w1474:bool)
        n621 = case shown="False" w1474 {
          tunnel: w1468 -> [w1486 w1494]
          tunnel: w1473 -> [w1481 _]
          tunnel: w1472 -> [w1487 w1493]
          tunnel: w1469 -> [w1488 _]
          tunnel: [w1477 w1490] -> w1470
          frame False {
            n622 = property class="Bool (strict)"(reference=w1486, "Value"=TRUE) -> ()  [unwired: 1 in, 2 out]
            n623 = call "AMC Send Local Messages.vi"("Message Names"=string[] ["Initialize Reference", "Monitor Reference"], "Message Queue in"=w1481) -> ()  [unwired: 8 in, 2 out]
            n624 = Enqueue Element(queue=w1488, element=cluster{"Msg":string, "Data":variant} {"Msg"="Initialize DAQ", "Data"=variant}, error in (no error)=w1487) -> (error out=w1482:errorcluster)  [unwired: 1 in, 2 out]
            n625 = call "AE Variables.vi"("VariantIn"=TRUE, "error in (no error)"=w1482, "Action"=Enum_Variables."Set DAQ Connected") -> ("error out"=w1478:errorcluster)  [unwired: 9 in, 7 out]
            n626 = call "Notifier AE.vi"("error in (no error)"=w1478, "String"="Starting DAQ") -> ("error out"=w1477:errorcluster)  [unwired: 9 in]
          }
          frame True {
            w1492 = FALSE ("Value")
            n627 = property class="Bool (strict)"(reference=w1494, error in=w1493, "Value"=w1492) -> (error out=w1490:errorcluster)  [unwired: 1 out]
            n628 = call "AE Variables.vi"("VariantIn"=w1492, "Action"=Enum_Variables."Set DAQ Connected") -> ()  [unwired: 10 in, 8 out]
          }
        }
      }
      frame "Send Segment to Acquisition" {
        n629 = Unbundle By Name(w1502) -> ("Acquisition.Queue"=w1501:refnum<queue>, "User Parameters.Measuring Limb"=w1498:string)
        n630 = Bundle By Name(cluster=cluster{"Msg":string, "Data":variant} {"Msg"="", "Data"=variant} ("element"), "Msg"="Set Segment", "Data"=w1498) -> (w1500:cluster{"Msg":string, "Data":variant})
        n631 = Enqueue Element(queue=w1501, element=w1500, error in (no error)=w1496) -> (error out=w1495:errorcluster)  [unwired: 1 in, 2 out]
      }
      frame "Regulation Stopped" {
        n632 = Unbundle By Name(w1507) -> ("Acquisition.Queue"=w1506:refnum<queue>)
        n633 = Enqueue Element(queue=w1506, element=cluster{"Msg":string, "Data":variant} {"Msg"="Control: Regulation Stopped", "Data"=variant}, error in (no error)=w1504) -> (error out=w1503:errorcluster)  [unwired: 1 in, 2 out]
      }
      frame "AcqTest" {
        n634 = Unbundle By Name(w1511) -> ("Acquisition.Queue"=w1510:refnum<queue>)
        n635 = flat-sequence {
          tunnel: w1510 -> [w1516]
          tunnel: [w1515] -> w1508
          tunnel: w1513 -> [w1519]
          tunnel: [w1519] -> w1512
          tunnel: [w1517] -> w1509
          tunnel: w1508 -> [w1517]
          tunnel: w1509 -> [w1521]
          frame #0 {
            n636 = Enqueue Element(queue=w1516, element=cluster{"Msg":string, "Data":variant} {"Msg"="Test", "Data"=variant}) -> (queue out=w1515:refnum<queue>)  [unwired: 2 in, 2 out]
          }
          frame #1 {
            n637 = Wait (ms)(milliseconds to wait=u32 10000) -> ()  [unwired: 1 out]
          }
          frame #2 {
            n638 = Enqueue Element(queue=w1521, element=cluster{"Msg":string, "Data":variant} {"Msg"="Idle", "Data"=variant}) -> ()  [unwired: 2 in, 3 out]
          }
        }
      }
      frame "Monitor Reference" {
        n639 = Unbundle By Name(w1526) -> ("Reference signal.Queue"=w1524:refnum<queue>, "Data Acquisition.Control?"=w1522:bool)
        n640 = case shown="False" w1522 {
          tunnel: w1525 -> [w1534 w1535]
          tunnel: w1524 -> [w1530 _]
          tunnel: [w1527 w1535] -> w1523
          frame False {
            n641 = call "AE Paper.vi"("error in (no error)"=w1534, "Action Events"=Enum_Paper_Action_Events."Init") -> ("error out"=w1532:errorcluster)  [unwired: 7 in, 1 out]
            n642 = call "AE Events.vi"("error in (no error)"=w1532, "Action"=enum16{"Init", "Get Event", "Set Event"}."Init") -> ("error out"=w1529:errorcluster)  [unwired: 8 in, 1 out]
            n643 = Enqueue Element(queue=w1530, element="Start", error in (no error)=w1529) -> (error out=w1527:errorcluster)  [unwired: 1 in, 2 out]
          }
          frame True {
          }
        }
      }
      frame "Idle Monitor Reference" {
        n644 = Unbundle By Name(w1540) -> ("Reference signal.Queue"=w1538:refnum<queue>, "Data Acquisition.Control?"=w1536:bool)
        n645 = case shown="False" w1536 {
          tunnel: w1539 -> [w1543 w1545]
          tunnel: w1538 -> [w1542 _]
          tunnel: [w1541 w1545] -> w1537
          frame False {
            n646 = Enqueue Element(queue=w1542, element="Idle", error in (no error)=w1543) -> (error out=w1541:errorcluster)  [unwired: 1 in, 2 out]
          }
          frame True {
          }
        }
      }
      frame "Stop Monitor Reference" {
        n647 = Unbundle By Name(w1550) -> ("Reference signal.Queue"=w1548:refnum<queue>, "Data Acquisition.Control?"=w1546:bool)
        n648 = case shown="True" w1546 {
          tunnel: w1549 -> [w1551 w1554]
          tunnel: w1548 -> [_ w1553]
          tunnel: [w1551 w1552] -> w1547
          frame False {
          }
          frame True {
            n649 = Enqueue Element(queue=w1553, element="Stop", error in (no error)=w1554) -> (error out=w1552:errorcluster)  [unwired: 1 in, 2 out]
          }
        }
      }
      frame "CreateLogPath" {
        # "Store data to local temporary directory"
        n650 = Unbundle By Name(w1566) -> ("User Parameters.CPR Number"=w1567:string, "User Parameters.Measuring Limb"=w1564:string, "System Parameters.Date"=w1556:string)
        n651 = disable-structure shown="Disabled" {
          frame Disabled {
            # "Create date string"
            n652 = Get Date/Time In Seconds() -> (seconds since 1Jan1904=w1568:timestamp)
            n653 = Format Date/Time String(time format string (%c)="%Y-%m-%d", seconds (now)=w1568) -> ()  [unwired: 1 in, 1 out]
          }
          frame Enabled {
          }
        }
        n654 = call "DataFileName(SubVI).vi"("error in (no error)"=w1563, "Date"=w1556, "Segment"=w1564, "CPR"=w1567) -> ("error out"=w1562:errorcluster, "Relative path"=w1557:path, "Path"=w1558:path)  [unwired: 1 in]
        n655 = Temporary Directory() -> (w1561:path)
        n656 = Build Path(base path=w1561, name or relative path="data.tdms") -> (appended path=w1559:path)
        n657 = Bundle By Name(cluster=w1566, "Data Acquisition.RecordPath"=w1558, "Data Acquisition.RelativeRecordPath"=w1557) -> (w1565:T3)
        n658 = global write "DataAcqRecordPathGlobal.vi" "DataAcqRecordPath"(w1559) -> ()
      }
      frame "Acquisition" {
        # "Set the start of acquisition"
        n659 = Unbundle By Name(w1575) -> ("Acquisition.Queue"=w1574:refnum<queue>)
        n660 = Enqueue Element(queue=w1574, element=cluster{"Msg":string, "Data":variant} {"Msg"="Acquire", "Data"=variant}, error in (no error)=w1573) -> (error out=w1572:errorcluster)  [unwired: 1 in, 2 out]
        n661 = Get Date/Time In Seconds() -> (seconds since 1Jan1904=w1576:timestamp)
        n662 = Bundle By Name(cluster=w1575, "Data Acquisition.Duration"=w1576, "Data Acquisition.Acquisition"=TRUE) -> (w1577:T3)
      }
      frame "Stop Acquisition" {
        n663 = call "removeShortMeasurement.vi"("error in (no error)"=w1584, "Queue in"=w1583, "SHIFTER DATA"=w1582) -> ("error out"=w1580:errorcluster)  [unwired: 8 in]
        n664 = Unbundle By Name(w1582) -> ("Acquisition.Queue"=w1578:refnum<queue>)
        n665 = Enqueue Element(queue=w1578, element=cluster{"Msg":string, "Data":variant} {"Msg"="Reset Active Graphs", "Data"=variant}, error in (no error)=w1580) -> (error out=w1579:errorcluster)  [unwired: 1 in, 2 out]
        n666 = Bundle By Name(cluster=w1582, "Data Acquisition.Acquisition"=FALSE) -> (w1586:T3)
      }
      frame "LogData" {
        n667 = Unbundle By Name(w1597) -> ("Data Acquisition.RecordPath"=w1594:path, "User Parameters.Measuring Type"=w1593:string, "User Parameters.Measuring Technique"=w1596:string, "User Parameters.Measuring Limb"=w1592:string)
        n668 = call "AE Variables.vi"("Action"=Enum_Variables."Get Height") -> ("NumericOut"=w1589:dbl)  [unwired: 11 in, 7 out]
        n669 = Divide(x=w1589, y=0.76) -> (x/y=w1587:dbl)
        n670 = Number To Decimal String(number=w1587) -> (decimal integer string=w1591:string)  [unwired: 1 in]
        n671 = Empty String/Path?(string/path=w1594) -> (empty?=w1595:bool)
        n672 = case shown="False" w1595 {
          tunnel: w1596 -> [w1610 _]
          tunnel: w1594 -> [w1602 _]
          tunnel: w1593 -> [w1601 _]
          tunnel: w1592 -> [w1600 _]
          tunnel: w1591 -> [w1599 _]
          frame False {
            n673 = Build Array(w1601, w1610, w1600, w1599) -> (w1604:string[])
            n674 = Strip Path(path=w1602) -> (stripped path=w1603:path)  [unwired: 1 out]
            n675 = Build Path(base path=w1603, name or relative path=T19 "patientdata.dm2000") -> (appended path=w1605:path)
            n676 = call-poly <vilib>:"Write To Spreadsheet File.vi"("delimiter (\\t)"="," ("delimiter (\\t)"), "format (%s)"="%s", "append to file? (new file:F)"=FALSE, "1D data"=w1604, "file path (dialog if empty)"=w1605) -> ()  [unwired: 3 in, 1 out]
          }
          frame True {
          }
        }
      }
      frame "AddTreeItems" {
        n677 = Unbundle By Name(w1619) -> ("cRef.Journal.References.Menu"=w1611:refnum<vi>, "cRef.Data.References.Menu"=w1613:refnum<vi>, "Data Acquisition.RecordPath"=w1612:path)
        n678 = call <vilib>:"Check if File or Folder Exists.vi"("error in (no error)"=w1616, "path"=w1612) -> ("error out"=w1617:errorcluster, "file or folder exists?"=w1615:bool, "dup path"=w1614:path)  [unwired: 7 in]
        n679 = case shown="True" w1615 {
          tunnel: w1617 -> [w1623 w1633]
          tunnel: [w1622 w1635] -> w1618
          tunnel: w1614 -> [w1621 w1634]
          tunnel: w1613 -> [_ w1631]
          tunnel: w1611 -> [_ w1630]
          frame False {
            n680 = Empty String/Path?(string/path=w1621) -> (empty?=w1620:bool)
            n681 = case shown="False" w1620 {
              tunnel: w1623 -> [w1626 w1629]
              tunnel: [w1625 w1629] -> w1622
              tunnel: w1621 -> [w1624 _]
              frame False {
                n682 = Strip Path(path=w1624) -> (stripped path=w1628:path)  [unwired: 1 out]
                n683 = Delete(path (use dialog)=w1628, entire hierarchy (F)=TRUE, error in=w1626) -> (error out=w1625:errorcluster)  [unwired: 2 in, 2 out]
              }
              frame True {
              }
            }
          }
          frame True {
            n684 = case shown="False" FALSE {
              tunnel: w1634 -> [w1644 w1649]
              tunnel: w1633 -> [w1645 w1648]
              tunnel: [w1641 w1647] -> w1635
              tunnel: w1631 -> [w1637 _]
              tunnel: w1630 -> [w1636 _]
              frame False {
                n685 = Strip Path(path=w1644) -> (stripped path=w1643:path)  [unwired: 1 out]
                n686 = call "TreeMenuUpdatePath.vi"("error in"=w1645, "Level"=2, "ProcessDataTreeMenu"=w1637, "stripped path"=w1643) -> ("error out"=w1642:errorcluster, "stripped path out"=w1640:path)  [unwired: 1 in]
                n687 = call "TreeMenuUpdatePath.vi"("error in"=w1642, "Level"=1, "ProcessDataTreeMenu"=w1636, "stripped path"=w1640) -> ("error out"=w1641:errorcluster)  [unwired: 1 in, 1 out]
              }
              frame True {
                n688 = disable-structure shown="Disabled" {
                  disable-tunnel: w1649 -> [w1654 _]
                  disable-tunnel: w1648 -> [w1653 _]
                  disable-tunnel: [w1652 _] -> w1647
                  frame Disabled {
                    n689 = Strip Path(path=w1654) -> (stripped path=w1651:path)  [unwired: 1 out]
                    n690 = Delete(path (use dialog)=w1651, entire hierarchy (F)=TRUE, error in=w1653) -> (error out=w1652:errorcluster)  [unwired: 2 in, 2 out]
                  }
                  frame Enabled {
                  }
                }
                n691 = One Button Dialog(message="Yes") -> ()  [unwired: 1 in, 1 out]
              }
            }
          }
        }
      }
      frame "ProcessRecent" {
        n692 = Unbundle By Name(w1657) -> ("Data Acquisition.RecordPath"=w1660:path, "cRef.Data.References.Menu"=w1655:refnum<vi>)
        n693 = Empty String/Path?(string/path=w1660) -> (empty?=w1661:bool)
        n694 = case shown="False" w1661 {
          tunnel: w1660 -> [w1675 _]
          tunnel: w1659 -> [w1664 w1676]
          tunnel: [w1662 w1676] -> w1658
          tunnel: w1657 -> [w1672 w1677]
          tunnel: [w1670 w1677] -> w1656
          tunnel: w1655 -> [w1663 _]
          frame False {
            n695 = Strip Path(path=w1675) -> (stripped path=w1666:path)  [unwired: 1 out]
            n696 = Strip Path(path=w1666) -> (stripped path=w1674:path)  [unwired: 1 out]
            n697 = Path To String(path=w1674) -> (string=w1667:string)
            n698 = invoke class="Tree (strict)" method="Open/Close.Item"(reference=w1663, error in=w1664, "tag"=w1667, "Open"=TRUE ("Open?")) -> (reference out=w1669:refnum<vi>, error out=w1668:errorcluster)  [unwired: 1 in, 3 out]
            n699 = Path To String(path=w1666) -> (string=w1671:string)
            n700 = Path To String(path=w1666) -> (string=w1665:string)
            n701 = property class="Tree (strict)"(reference=w1669, error in=w1668, "Value"=w1665) -> (error out=w1662:errorcluster)  [unwired: 1 out]
            n702 = Bundle By Name(cluster=w1672, "Data Process.ActiveItemTag"=w1671) -> (w1670:T3)
          }
          frame True {
          }
        }
      }
      frame "Stop Reference" {
        n703 = Unbundle By Name(w1692) -> ("Reference signal.Queue"=w1688:refnum<queue>, "Data Acquisition.Control?"=w1679:bool, "Acquisition.Queue"=w1680:refnum<queue>)
        n704 = Enqueue Element(queue=w1680, element=cluster{"Msg":string, "Data":variant} {"Msg"="Halt DAQ", "Data"=variant}, error in (no error)=w1685) -> (error out=w1689:errorcluster)  [unwired: 1 in, 2 out]
        n705 = case shown="False" w1679 {
          tunnel: w1689 -> [w1696 w1697]
          tunnel: w1688 -> [w1695 _]
          tunnel: [w1693 w1697] -> w1684
          frame False {
            n706 = Enqueue Element(queue=w1695, element="Stop" ("DataAcqState"), error in (no error)=w1696) -> (error out=w1693:errorcluster)  [unwired: 1 in, 2 out]
          }
          frame True {
          }
        }
        n707 = call "AE Variables.vi"("VariantIn"=FALSE, "error in (no error)"=w1684, "Action"=Enum_Variables."Set DAQ Connected") -> ("error out"=w1683:errorcluster)  [unwired: 9 in, 7 out]
        n708 = call-poly <userlib>:"Filter Error Codes__ogtk.vi"("Error In"=w1683, "Error Codes to Filter"=i32[] [1, 1000]) -> ("Error Out"=w1686:errorcluster)  [unwired: 7 in, 2 out]
        n709 = Bundle By Name(cluster=w1692, "Reference signal.Monitor"=FALSE) -> (w1691:T3)
      }
      frame "Calibrate Pressure: Step 1" {
        # "Dont detect paper movement"
        # "Temporary file location"
        n710 = global read "DataPathGlobalVariable.vi" "DataPath"() -> (w1703:path)
        n711 = global write "DataAcqRecordPathGlobal.vi" "PressureCalibrationFactor"(1.0 ("PressureCalibrationFactor")) -> ()
        n712 = Build Path(base path=w1703, name or relative path="calibration.tdms") -> (appended path=w1701:path)
        n713 = global write "DataAcqRecordPathGlobal.vi" "DataAcqRecordPath"(w1701) -> ()
        n714 = Bundle By Name(cluster=w1698, "Reference signal.Monitor"=FALSE) -> (w1705:T3)
      }
      frame "Calibrate Pressure: Step 2" {
        w1710 = cluster{"Msg":string, "Data":variant} {"Msg"="", "Data"=variant} ("element")
        # "Start acquisition"
        n715 = Unbundle By Name(w1715) -> ("Acquisition.Queue"=w1714:refnum<queue>, "Data Acquisition.Control?"=w1706:bool)
        n716 = Bundle By Name(cluster=w1710, "Msg"="Acquire") -> (w1711:cluster{"Msg":string, "Data":variant})
        n717 = Enqueue Element(queue=w1714, element=w1711, error in (no error)=w1707) -> (queue out=w1713:refnum<queue>, error out=w1709:errorcluster)  [unwired: 1 in, 1 out]
        n718 = case shown="True" w1706 {
          tunnel: w1713 -> [_ w1722]
          tunnel: w1710 -> [_ w1721]
          tunnel: w1709 -> [w1716 w1718]
          tunnel: [w1716 w1717] -> w1708
          frame False {
          }
          frame True {
            n719 = Bundle By Name(cluster=w1721, "Msg"="Control: Deflate") -> (w1720:cluster{"Msg":string, "Data":variant})
            n720 = Enqueue Element(queue=w1722, element=w1720, error in (no error)=w1718) -> (error out=w1717:errorcluster)  [unwired: 1 in, 2 out]
          }
        }
      }
      frame "Calibrate Pressure: Step 3" {
        w1745 = 5 items=["No error", "Argument error", "Memory is full", "Out of zone", "End of file", "File already open", "Generic file I/O error", "File not found", "File permission error", "Disk is full", "Duplicate path", "Too many files open", "System feature not enabled", "Resource file not found", "Cannot add resource", "Resource not found", "Image not found", "Image memory error", "Pen does not exist", "Config type invalid", "Config token not found", "Config parse error", "Config memory error", "Bad external code format", "Bad external code offset", "External code not present", "Null window", "Destroy window error", "Null menu", "Print aborted", "Bad print record", "Print driver error", "Windows error during printing", "Memory error during printing", "Print dialog error", "Generic print error", "Invalid device refnum", "Device not found", "Device parameter error", "Device unit error", "Cannot open device", "Device call aborted", "Generic error", "Cancelled by user", "Object ID too low", "Object ID too high", "Object not in heap", "Unknown heap", "Unknown object (invalid DefProc)", "Unknown object (DefProc not in table)", "Message out of range", "Invalid (null) method", "Unknown message", "Manager call not supported", "Bad address", "Network operation in progress", "Network operation timed out", "Connection is busy", "Network attribute not supported", "Network error", "Address in use", "System out of memory", "Connection aborted", "Connection refused", "Not connected", "Already connected", "Connection closed", "Initialization error (interapplication manager)", "Bad occurrence", "Wait on unbound occurrence handler", "Occurrence queue overflow", "Datalog type conflict", "Unused", "Unrecognized type (interapplication manager)", "Memory corrupt", "Failed to make temporary DLL", "Old CIN version", "Drag socket not found", "Failed to load drop-object", "Failed to register OLE object", "Failed to release OLE object", "Format specifier type mismatch", "Unknown format specifier", "Too few format specifiers", "Too many format specifiers", "Scan failed", "Newer CIN version", "OLE Convert", "Runtime menu error", "Password tampered", "Unknown error code"] ("Error Code")
        # "Calculate calibration factor from measurement"
        n721 = global read "DataAcqRecordPathGlobal.vi" "DataAcqRecordPath"() -> (w1749:path)
        n722 = Unbundle By Name(w1732) -> ("Data Acquisition.Control?"=w1724:bool, "Acquisition.Queue"=w1731:refnum<queue>)
        n723 = call "AutomaticCalibration.vi"("error in (no error)"=w1730, "Path"=w1749) -> ("error out"=w1747:errorcluster, "Path Out"=w1748:path)  [unwired: 8 in]
        n724 = Delete(path (use dialog)=w1748, error in=w1747) -> (deleted path=w1738:path, error out=w1746:errorcluster)  [unwired: 3 in, 1 out]
        n725 = call-poly <userlib>:"MGI Suppress Error Code.vi"("Error Code"=w1745, "Error In"=w1746) -> ("Error Supressed?"=w1739:bool, "Error Out"=w1736:errorcluster)  [unwired: 4 in]
        n726 = case shown="True" w1739 {
          tunnel: w1738 -> [w1758 w1761]
          tunnel: [w1758 w1759] -> w1737
          tunnel: w1736 -> [w1757 w1764]
          tunnel: [w1757 w1762] -> w1735
          frame False {
          }
          frame True {
            n727 = flat-sequence {
              tunnel: w1764 -> [w1766]
              tunnel: [w1766] -> w1763
              tunnel: w1761 -> [w1765]
              tunnel: [w1765] -> w1760
              tunnel: w1763 -> [w1771]
              tunnel: [w1770] -> w1762
              tunnel: w1760 -> [w1769]
              tunnel: [w1768] -> w1759
              frame #0 {
                n728 = Wait (ms)(milliseconds to wait=u32 1000) -> ()  [unwired: 1 out]
              }
              frame #1 {
                n729 = Delete(path (use dialog)=w1769, error in=w1771) -> (deleted path=w1768:path, error out=w1770:errorcluster)  [unwired: 3 in, 1 out]
              }
            }
          }
        }
        n730 = Enqueue Element(queue=w1731, element=cluster{"Msg":string, "Data":variant} {"Msg"="Idle", "Data"=variant}, error in (no error)=w1730) -> (queue out=w1723:refnum<queue>, error out=w1726:errorcluster)  [unwired: 1 in, 1 out]
        n731 = case shown="True" w1724 {
          tunnel: w1726 -> [w1752 w1755]
          tunnel: [w1752 w1754] -> w1725
          tunnel: w1723 -> [_ w1753]
          frame False {
          }
          frame True {
            n732 = Enqueue Element(queue=w1753, element=cluster{"Msg":string, "Data":variant} {"Msg"="Control: Halt Deflate", "Data"=variant}, error in (no error)=w1755) -> (error out=w1754:errorcluster)  [unwired: 1 in, 2 out]
          }
        }
        n733 = Strip Path(path=w1737) -> (stripped path=w1740:path, name=w1743:string)
        n734 = Concatenate Strings(w1743, "_index" ("name or relative path")) -> (w1741:string)
        n735 = Bundle By Name(cluster=w1732, "Reference signal.Monitor"=TRUE) -> (w1751:T3)
        n736 = Build Path(base path=w1740, name or relative path=w1741) -> (appended path=w1744:path)
        n737 = Delete(path (use dialog)=w1744, error in=w1735) -> (error out=w1734:errorcluster)  [unwired: 3 in, 2 out]
        n738 = call-poly <userlib>:"MGI Suppress Error Code.vi"("Error Code"=1430, "Error In"=w1734) -> ("Error Out"=w1728:errorcluster)  [unwired: 4 in, 1 out]
        n739 = Merge Errors(w1728, w1725) -> (w1729:errorcluster)
      }
      frame "Check Data Folder" {
        n740 = global read "DataPathGlobalVariable.vi" "DataPath"() -> (w1773:path)
        n741 = call <vilib>:"Check if File or Folder Exists.vi"("error in (no error)"=w1775, "path"=w1773) -> ("error out"=w1772:errorcluster, "file or folder exists?"=w1777:bool)  [unwired: 7 in, 1 out]
        n742 = case shown="False" w1777 {
          tunnel: w1776 -> [_ _]
          tunnel: w1772 -> [w1779 w1782]
          tunnel: [w1779 w1782] -> w1774
          frame False {
            n743 = One Button Dialog(message="The Data folder has not been found. Please replace the Data folder in the application directory or start data acquisition to generate a new one. ", button name ("OK")="Close") -> ()  [unwired: 1 out]
          }
          frame True {
          }
        }
      }
      frame "ChangeTab" {
      }
      frame "/***Data Processing***/" {
      }
      frame "GetActiveItemTag" {
        n744 = Bundle By Name(cluster=w1789, "Data Process.ActiveItemTag"=w1787) -> (w1788:T3)
      }
      frame "FilterControl" {
        n745 = Unbundle By Name(w1795) -> ("cRef.Data.References.FilterControl"=w1794:refnum<vi>)
        n746 = property class="Bool (strict)"(reference=w1794, error in=w1792) -> (error out=w1791:errorcluster, "Value"=w1793:bool)  [unwired: 1 out]
        n747 = call "AE Variables.vi"("VariantIn"=w1793, "error in (no error)"=w1791, "Action"=Enum_Variables."Set Filter") -> ("error out"=w1796:errorcluster)  [unwired: 9 in, 7 out]
      }
      frame "Display Data" {
        # "Open measurement and display graph"
        n748 = Unbundle By Name(w1799) -> ("Data Process.ActiveItemTag"=w1805:string, "Data.Queue"=w1800:refnum<queue>)
        n749 = String To Path(string=w1805) -> (path=w1806:path)
        n750 = Build Path(base path=w1806, name or relative path="Data.tdms") -> (appended path=w1803:path)
        n751 = call-poly <userlib>:"File Exists__ogtk.vi"("file path"=w1803) -> ("exists"=w1804:bool)  [unwired: 6 in, 1 out]
        n752 = case shown="True" w1804 {
          tunnel: w1802 -> [w1808 w1819]
          tunnel: w1803 -> [_ w1816]
          tunnel: [w1808 w1817] -> w1801
          tunnel: w1800 -> [_ w1814]
          frame False {
          }
          frame True {
            # "Send command to data processing vi"
            n753 = call "AE DataProcessControl.vi"("Action"=Enum_Process_Data."Set Data Path", "error in (no error)"=w1819, "Data Path In"=w1816) -> ("error out"=w1815:errorcluster)  [unwired: 6 in, 2 out]
            n754 = call "GetHeightAdj.vi"("appended path"=w1816) -> ("Numeric"=w1809:dbl)
            n755 = Enqueue Element(queue=w1814, element=cluster{"Msg":string, "Data":variant} {"Msg"="Update", "Data"=variant}, error in (no error)=w1815) -> (error out=w1812:errorcluster)  [unwired: 1 in, 2 out]
            n756 = call "AE Variables.vi"("VariantIn"=w1809, "error in (no error)"=w1812, "Action"=Enum_Variables."Set Recorded Height") -> ("error out"=w1811:errorcluster)  [unwired: 9 in, 7 out]
            n757 = call "AE Variables.vi"("error in (no error)"=w1811, "Action"=Enum_Variables."Reset Pressure") -> ("error out"=w1817:errorcluster)  [unwired: 10 in, 7 out]
          }
        }
        n758 = Bundle By Name(cluster=w1799, "Database.PatientdataPath"=w1806) -> (w1798:T3)
      }
      frame "Flow: View Signals" {
        n759 = Unbundle By Name(w1826) -> ("Data Process.ActiveItemTag"=w1825:string)
        n760 = String To Path(string=w1825) -> (path=w1824:path)
        n761 = Build Path(base path=w1824, name or relative path="Data.tdms") -> (appended path=w1822:path)
        n762 = call-poly <userlib>:"File Exists__ogtk.vi"("file path"=w1822) -> ("exists"=w1821:bool)  [unwired: 6 in, 1 out]
        n763 = case shown="True" w1821 {
          tunnel: w1822 -> [_ w1828]
          frame False {
          }
          frame True {
            n764 = call "FlowPopup.vi"("Path"=w1828) -> ()  [unwired: 11 in]
          }
        }
      }
      frame "Set Tangent Mode" {
        n765 = Unbundle By Name(w1833) -> ("Data.Queue"=w1832:refnum<queue>, "cRef.Data.References.Tangent On/Off"=w1830:refnum<vi>)
        n766 = property class="Bool (strict)"(reference=w1830) -> ("Value"=w1829:bool)  [unwired: 1 in, 2 out]
        n767 = call "AE DataProcessControl.vi"("Action"=Enum_Process_Data."Set Cursor Mode", "error in (no error)"=w1836, "Cursor Mode In"=w1829) -> ("error out"=w1835:errorcluster)  [unwired: 6 in, 2 out]
        n768 = Enqueue Element(queue=w1832, element=cluster{"Msg":string, "Data":variant} {"Msg"="Set Tangent Mode", "Data"=variant}, error in (no error)=w1835) -> (error out=w1834:errorcluster)  [unwired: 1 in, 2 out]
      }
      frame "Set Tangent Mode: True" {
        w1838 = TRUE ("Value")
        n769 = Unbundle By Name(w1842) -> ("Data.Queue"=w1841:refnum<queue>, "cRef.Data.References.Tangent On/Off"=w1839:refnum<vi>)
        n770 = property class="Bool (strict)"(reference=w1839, "Value"=w1838) -> ()  [unwired: 1 in, 2 out]
        n771 = call "AE DataProcessControl.vi"("Action"=Enum_Process_Data."Set Cursor Mode", "error in (no error)"=w1845, "Cursor Mode In"=w1838) -> ("error out"=w1844:errorcluster)  [unwired: 6 in, 2 out]
        n772 = Enqueue Element(queue=w1841, element=cluster{"Msg":string, "Data":variant} {"Msg"="Set Tangent Mode", "Data"=variant}, error in (no error)=w1844) -> (error out=w1843:errorcluster)  [unwired: 1 in, 2 out]
      }
      frame "Reset Graphs" {
        n773 = Unbundle By Name(w1851) -> ("Data.Queue"=w1850:refnum<queue>, "cRef.Data.References.Tangent On/Off"=w1848:refnum<vi>)
        n774 = property class="Bool (strict)"(reference=w1848) -> ("Value"=w1847:bool)  [unwired: 1 in, 2 out]
        n775 = call "AE DataProcessControl.vi"("Action"=Enum_Process_Data."Set Cursor Mode", "error in (no error)"=w1854, "Cursor Mode In"=w1847) -> ("error out"=w1853:errorcluster)  [unwired: 6 in, 2 out]
        n776 = Enqueue Element(queue=w1850, element=cluster{"Msg":string, "Data":variant} {"Msg"="Reset", "Data"=variant}, error in (no error)=w1853) -> (error out=w1852:errorcluster)  [unwired: 1 in, 2 out]
      }
      frame "ExportGraphs" {
        w1859 = "\r"
        n777 = Unbundle By Name(w1866) -> ("User Parameters.CPR Number"=w1860:string, "User Parameters.Name"=w1861:string, "User Parameters.Operator"=w1865:string, "User Parameters.Measuring Type"=w1858:string)
        n778 = call "FindDatePath.vi"("Message Value"=w1863) -> ("String"=w1862:string)  [unwired: 10 in]
        n779 = Concatenate Strings(w1860, w1859, w1861, w1859, w1865) -> (w1864:string)
        n780 = call "exportGraphsToPDF.vi"("PatientID"=w1860, "error in (no error)"=w1867, "Type"=w1858, "Text"=w1864, "Folder"=w1862) -> ("error out"=w1857:errorcluster)  [unwired: 6 in]
        n781 = case shown="Error" w1857 {
          selector: w1857 -> [w1868 w1872]
          tunnel: [w1868 errorcluster {"status"=FALSE, "code"=0, "source"=""} ("error IO")] -> w1856
          frame No Error {
          }
          frame Error {
            n782 = Unbundle By Name(w1872) -> ("source"=w1871:string)
            n783 = Concatenate Strings("An error occured when trying to export the graph:  " ("message"), w1871) -> (w1869:string)
            n784 = One Button Dialog(message=w1869) -> ()  [unwired: 1 in, 1 out]
          }
        }
      }
      frame "ChangeSegment" {
        n785 = Unbundle By Name(w1875) -> ("cRef.Configuration.References.ListboxMeasurementArea"=w1874:refnum<vi>)
        n786 = call "ChangeSegment.vi"("error in (no error)"=w1881, "Message Value"=w1876, "cRef.Configuration.References.ListboxMeasurementArea"=w1874) -> ("error out"=w1879:errorcluster, "Moved?"=w1880:bool, "target out"=w1877:path)  [unwired: 6 in]
        n787 = case shown="True" w1880 {
          tunnel: w1879 -> [w1882 w1902]
          tunnel: [w1882 w1886] -> w1878
          tunnel: w1877 -> [_ w1898]
          tunnel: w1876 -> [_ w1895]
          tunnel: w1875 -> [_ w1892]
          frame False {
          }
          frame True {
            n788 = Unbundle By Name(w1892) -> ("User Parameters.CPR Number"=w1891:string, "cRef.Data.References.Menu"=w1884:refnum<vi>, "cRef.Journal.References.Menu"=w1883:refnum<vi>)
            n789 = invoke class="Tree (strict)" method="Edit Tree Items.Delete"(reference=w1884, error in=w1902, "tag"=w1895, "Delete Children"=TRUE ("Delete Children?")) -> (reference out=w1896:refnum<vi>, error out=w1899:errorcluster)  [unwired: 1 in, 3 out]
            n790 = global read "DataPathGlobalVariable.vi" "DataPath"() -> (w1889:path)
            n791 = call "Encrypt.vi"("Input"=w1891) -> ("Output"=w1890:string)  [unwired: 10 in]
            n792 = call "TreeMenuUpdatePath.vi"("error in"=w1899, "Level"=2, "ProcessDataTreeMenu"=w1896, "stripped path"=w1898) -> ("error out"=w1894:errorcluster, "stripped path out"=w1893:path)  [unwired: 1 in]
            n793 = Build Path(base path=w1889, name or relative path=w1890) -> (appended path=w1888:path)
            n794 = Path To String(path=w1893) -> (string=w1900:string)
            n795 = property class="Tree (strict)"(reference=w1896, error in=w1894, "Value"=w1900) -> (error out=w1885:errorcluster)  [unwired: 1 out]
            n796 = call "Init_Open_Close.vi"("error in"=w1885, "Level"=1, "path to start the search"=w1888, "Tree In"=w1883) -> ("error out"=w1886:errorcluster)  [unwired: 5 in, 2 out]
          }
        }
      }
      frame "DeleteTreeItem" {
        n797 = Two Button Dialog(message="Are you sure you want to delete this data permanently?", 2:"Yes" ("T button name (\"OK\")")) -> (T button?=w1907:bool)  [unwired: 1 in]
        n798 = case shown="True" w1907 {
          tunnel: w1908 -> [_ w1921]
          tunnel: w1906 -> [w1910 w1915]
          tunnel: [w1910 w1920] -> w1909
          tunnel: w1908 -> [_ w1914]
          tunnel: w1903 -> [_ w1913]
          frame False {
          }
          frame True {
            n799 = Unbundle By Name(w1913) -> ("cRef.Data.References.Menu"=w1912:refnum<vi>, "cRef.Journal.References.Menu"=w1911:refnum<vi>)
            n800 = String To Path(string=w1914) -> (path=w1917:path)
            n801 = Delete(path (use dialog)=w1917, entire hierarchy (F)=TRUE, confirm (F)=FALSE, error in=w1915) -> (error out=w1916:errorcluster)  [unwired: 1 in, 2 out]
            n802 = Build Array(w1912, w1911) -> (w1922:refnum<vi>[])
            n803 = for {
              tunnel: w1922 -> [w1925] mode=indexing
              tunnel: w1921 -> [w1928]
              tunnel: w1916 -> [w1926]
              tunnel: [w1923] -> w1920
              n804 = invoke class="Tree (strict)" method="Edit Tree Items.Delete"(reference=w1925, error in=w1926, "tag"=w1928, "Delete Children"=TRUE ("Delete Children?")) -> (error out=w1924:errorcluster)  [unwired: 1 in, 4 out]
              n805 = call <userlib>:"Clear All Errors__ogtk.vi"("Error In"=w1924) -> ("Error Out"=w1923:errorcluster)  [unwired: 3 in]
            }
          }
        }
      }
      frame "/***Journal***/" {
      }
      frame "FillDataTable" {
        # "Update path to user/date"
        # "Extract data and populate table"
        n806 = Unbundle By Name(w1939) -> ("cRef.Journal.References.Data"=w1931:refnum<vi>, "Database.ActiveItemTag"=w1937:string)
        n807 = Empty String/Path?(string/path=w1936) -> (empty?=w1935:bool)
        n808 = Select(t=w1937, s=w1935, f=w1936) -> (s? t:f=w1938:string)
        n809 = String To Path(string=w1938) -> (path=w1933:path)
        n810 = call-poly <userlib>:"File Exists__ogtk.vi"("file path"=w1933) -> ("exists"=w1934:bool)  [unwired: 6 in, 1 out]
        n811 = case shown="True" w1934 {
          tunnel: [w1942 w1946] -> w1940
          tunnel: w1932 -> [w1942 w1945]
          tunnel: w1933 -> [_ w1944]
          tunnel: w1931 -> [_ w1943]
          frame False {
          }
          frame True {
            n812 = case shown="No Error" w1945 {
              selector: w1945 -> [w1948 w1951]
              tunnel: [w1950 w1952] -> w1946
              tunnel: w1944 -> [w1949 _]
              tunnel: w1943 -> [w1947 _]
              frame No Error {
                n813 = call "ListboxItems (SubVI).vi"("error in (no error)"=w1948, "MCListbox Refnum"=w1947, "path"=w1949) -> ("error out"=w1950:errorcluster)  [unwired: 2 in]
              }
              frame Error {
                n814 = call-poly <userlib>:"MGI Suppress Error Code.vi"("Error Code"=1430, "Error In"=w1951) -> ("Error Out"=w1952:errorcluster)  [unwired: 4 in, 1 out]
              }
            }
          }
        }
        n815 = Bundle By Name(cluster=w1939, "Database.ActiveItemTag"=w1938) -> (w1941:T3)
      }
      frame "GenerateReport" {
        n816 = Unbundle By Name(w1962) -> ("Database.ActiveItemTag"=w1955:string, "cRef.Journal.References.ReportSelection"=w1957:refnum<vi>)
        n817 = case shown="False" FALSE {
          tunnel: [T20."leave excel open after last close" ("closing behavior (leave open)") T20."close excel after last close" ("closing behavior (leave open)")] -> w1963
          frame False {
          }
          frame True {
          }
        }
        n818 = property class="Ring (strict)"(reference=w1957) -> ("Value"=w1956:u16)  [unwired: 1 in, 2 out]
        n819 = Empty String/Path?(string/path=w1955) -> (empty?=w1954:bool)
        n820 = case shown="False" w1954 {
          tunnel: w1964 -> [w1970 w1972]
          tunnel: w1963 -> [w1969 _]
          tunnel: [w1968 path "" ("ReportPath")] -> w1960
          tunnel: [w1967 w1972] -> w1959
          tunnel: w1956 -> [w1965 _]
          tunnel: w1955 -> [w1966 _]
          frame False {
            n821 = call "GetDataForExcel.vi"("error in (no error)"=w1970, "ID"=w1966, "ReportSelection"=w1965, "closing behavior (leave open)"=w1969) -> ("error out"=w1967:errorcluster, "ReportPath"=w1968:path)  [unwired: 5 in, 1 out]
          }
          frame True {
          }
        }
        n822 = Bundle By Name(cluster=w1962, "Database.JournalPath"=w1960) -> (w1961:T3)
      }
      frame "DeleteSingleMeasurement" {
        n823 = Unflatten From String(type=cluster{i32, i32} {0, 0}, binary string=w1995, error in (no error)=w1980) -> (value=w1993:cluster{i32, i32}, error out=w1982:errorcluster)  [unwired: 2 in, 1 out]
        n824 = Unbundle By Name(w1992) -> ("Database.ActiveItemTag"=w1978:string, "cRef.Journal.References.Data"=w1975:refnum<vi>)
        n825 = Unbundle(w1993) -> (w1991:i32, w1984:i32)
        n826 = String To Path(string=w1978) -> (path=w1976:path)
        n827 = List Folder(path=w1976, error in=w1982) -> (folder names=w1990:string[], error out=w1981:errorcluster)  [unwired: 2 in, 2 out]
        n828 = Index Array(array=w1990, index=w1991) -> (element=w1989:string)
        n829 = Build Path(base path=w1976, name or relative path=w1989) -> (appended path=w1988:path)
        n830 = Build Path(base path=w1988, name or relative path="processdata.dm2000") -> (appended path=w1986:path)
        n831 = call <vilib>:"Check if File or Folder Exists.vi"("error in (no error)"=w1981, "path"=w1986) -> ("error out"=w1979:errorcluster, "file or folder exists?"=w1985:bool, "dup path"=w1983:path)  [unwired: 7 in]
        n832 = case shown="True" w1985 {
          tunnel: w1984 -> [_ w2005]
          tunnel: w1983 -> [_ w2003]
          tunnel: w1979 -> [w1996 w2001]
          tunnel: [w1996 w2000] -> w1977
          tunnel: w1976 -> [_ w1999]
          tunnel: w1975 -> [_ w1997]
          frame False {
          }
          frame True {
            n833 = call-poly <vilib>:"Read From Spreadsheet File.vi"("delimiter (\\t)"=";" ("delimiter (\\t)"), "file path (dialog if empty)"=w2003) -> ("first row"=w2002:dbl[])  [unwired: 5 in, 4 out]
            n834 = case shown="1" w2005 {
              tunnel: w2003 -> [_ w2014 w2022]
              tunnel: w2002 -> [_ w2013 w2021]
              tunnel: w1999 -> [w2006 w2007 w2015]
              tunnel: [w2006 w2007 w2015] -> w1998
              frame 0, Default {
              }
              frame 1 {
                n835 = Replace Array Subset(array=w2013, new element=0.0 ("new element/subarray"), index=0) -> (w2010:dbl[])
                n836 = call-poly <vilib>:"Write To Spreadsheet File.vi"("delimiter (\\t)"=";" ("delimiter (\\t)"), "append to file? (new file:F)"=FALSE, "1D data"=w2010, "file path (dialog if empty)"=w2014) -> ()  [unwired: 4 in, 1 out]
              }
              frame 2 {
                n837 = Replace Array Subset(array=w2021, new element=0.0 ("new element/subarray"), index=1) -> (w2018:dbl[])
                n838 = call-poly <vilib>:"Write To Spreadsheet File.vi"("delimiter (\\t)"=";" ("delimiter (\\t)"), "append to file? (new file:F)"=FALSE, "1D data"=w2018, "file path (dialog if empty)"=w2022) -> ()  [unwired: 4 in, 1 out]
              }
            }
            n839 = call "ListboxItems (SubVI).vi"("error in (no error)"=w2001, "MCListbox Refnum"=w1997, "path"=w1998) -> ("error out"=w2000:errorcluster)  [unwired: 2 in]
          }
        }
      }
      frame "/****Save Data****/" {
      }
      frame "SaveArmPressure" {
        w2029 = 0 ("index (row)")
        w2035 = 0 ("index (row)")
        n840 = Unbundle By Name(w2052) -> ("User Parameters.CPR Number"=w2047:string, "System Parameters.Date"=w2050:string, "User Parameters.RightArm"=w2040:string[][], "User Parameters.LeftArm"=w2039:string[][], "User Parameters.Puls"=w2025:dbl)
        n841 = call "Encrypt.vi"("Input"=w2047) -> ("Output"=w2046:string)  [unwired: 10 in]
        n842 = global read "DataPathGlobalVariable.vi" "DataPath"() -> (w2048:path)
        n843 = Initialize Array(0, 2 ("dimension size"), 4) -> (w2031:i32[][])
        n844 = Decimal String To Number(string=w2040) -> (number=w2038:i32[][])  [unwired: 2 in, 1 out]
        n845 = Decimal String To Number(string=w2039) -> (number=w2037:i32[][])  [unwired: 2 in, 1 out]
        n846 = Transpose 2D Array(2D array=w2038) -> (transposed array=w2032:i32[][])
        n847 = Build Path(base path=w2048, name or relative path=w2046) -> (appended path=w2051:path)
        n848 = Transpose 2D Array(2D array=w2037) -> (transposed array=w2030:i32[][])
        n849 = Build Path(base path=w2051, name or relative path=w2050) -> (appended path=w2049:path)
        n850 = Replace Array Subset(array=w2031, new element=w2032, index (row)=w2035, index (col)=w2035) -> (w2028:i32[][])
        n851 = Replace Array Subset(array=w2031, new element=w2030, index (row)=w2029, index (col)=w2029) -> (w2027:i32[][])
        n852 = call <userlib>:"Create Dir if Non-Existant__ogtk.vi"("error in (no error)"=w2045, "Directory Path"=w2049) -> ("error out"=w2041:errorcluster, "dup Directory Path"=w2043:path)  [unwired: 7 in, 1 out]
        n853 = Build Array (concatenate)(w2028, w2027) -> (w2026:i32[][])
        n854 = Not A Number/Path/Refnum?(number/path/refnum=w2043) -> (NaN/Path/Refnum?=w2042:bool)
        n855 = case shown="No Error" w2041 {
          selector: w2041 -> [w2055 w2074]
          tunnel: w2043 -> [w2058 _]
          tunnel: [w2057 w2074] -> w2044
          tunnel: w2042 -> [w2056 _]
          tunnel: w2026 -> [w2054 _]
          tunnel: w2025 -> [w2053 _]
          frame No Error {
            n856 = case shown="False" w2056 {
              tunnel: [w2064 w2073] -> w2057
              tunnel: w2058 -> [w2065 _]
              tunnel: w2055 -> [w2064 w2072]
              tunnel: w2054 -> [w2063 _]
              tunnel: w2053 -> [w2061 _]
              frame False {
                n857 = Build Path(base path=w2065, name or relative path="armpressure.dm2000") -> (appended path=w2059:path)
                n858 = Build Array(w2061) -> (w2060:dbl[])
                n859 = Build Array (concatenate)(w2063, w2060) -> (w2062:dbl[][])
                n860 = call-poly <vilib>:"Write To Spreadsheet File.vi"("delimiter (\\t)"=";" ("delimiter (\\t)"), "append to file? (new file:F)"=FALSE, "2D data"=w2062, "file path (dialog if empty)"=w2059) -> ()  [unwired: 4 in, 1 out]
              }
              frame True {
                w2070 = 7 items=["No error", "Argument error", "Memory is full", "Out of zone", "End of file", "File already open", "Generic file I/O error", "File not found", "File permission error", "Disk is full", "Duplicate path", "Too many files open", "System feature not enabled", "Resource file not found", "Cannot add resource", "Resource not found", "Image not found", "Image memory error", "Pen does not exist", "Config type invalid", "Config token not found", "Config parse error", "Config memory error", "Bad external code format", "Bad external code offset", "External code not present", "Null window", "Destroy window error", "Null menu", "Print aborted", "Bad print record", "Print driver error", "Windows error during printing", "Memory error during printing", "Print dialog error", "Generic print error", "Invalid device refnum", "Device not found", "Device parameter error", "Device unit error", "Cannot open device", "Device call aborted", "Generic error", "Cancelled by user", "Object ID too low", "Object ID too high", "Object not in heap", "Unknown heap", "Unknown object (invalid DefProc)", "Unknown object (DefProc not in table)", "Message out of range", "Invalid (null) method", "Unknown message", "Manager call not supported", "Bad address", "Network operation in progress", "Network operation timed out", "Connection is busy", "Network attribute not supported", "Network error", "Address in use", "System out of memory", "Connection aborted", "Connection refused", "Not connected", "Already connected", "Connection closed", "Initialization error (interapplication manager)", "Bad occurrence", "Wait on unbound occurrence handler", "Occurrence queue overflow", "Datalog type conflict", "Unused", "Unrecognized type (interapplication manager)", "Memory corrupt", "Failed to make temporary DLL", "Old CIN version", "Drag socket not found", "Failed to load drop-object", "Failed to register OLE object", "Failed to release OLE object", "Format specifier type mismatch", "Unknown format specifier", "Too few format specifiers", "Too many format specifiers", "Scan failed", "Newer CIN version", "Error converting to variant", "Runtime menu error", "Password tampered", "Variant attribute not found", "Incompatible variant data type", "Event data is not available", "Event Store is not present", "Occurrence is not found", "Event Queue is not created", "Event info is not available", "Refnum passed is NULL", "Error retrieving Class GUID", "Error retrieving CoClass GUID", "Error retrieving TypeLib GUID.", "Bad built application magic bytes.", "Specific driver is different from the specific driver associated with the Logical Name.", "There is no session opened to the class driver.", "Max Error", "MAX - Error with config objects", "MAX - Error loading configuration", "MAX - Group not supported"]
                n861 = call <userlib>:"Build Error Cluster__ogtk.vi"("String to Prepend to source (\"\")"="Armpressure file could not be located or created" ("String to Prepend to source (\"\")"), "code"=w2070) -> ("error out"=w2071:errorcluster)
                n862 = Merge Errors(w2072, w2071) -> (w2073:errorcluster)
              }
            }
          }
          frame Error {
          }
        }
      }
      frame "SaveArmPressure_new" {
        n863 = Unbundle By Name(w2082) -> ("User Parameters.RightArm"=w2081:string[][], "User Parameters.Puls"=w2075:dbl)
        n864 = Decimal String To Number(string=w2081) -> (number=w2080:i32[][])  [unwired: 2 in, 1 out]
        n865 = Transpose 2D Array(2D array=w2080) -> (transposed array=w2076:i32[][])
        n866 = for {
          tunnel: w2079 -> [w2091]
          tunnel: [w2090] -> w2078
          tunnel: T21 {"sys"=0.0, "dia"=0.0, "puls"=0.0, "date"="", "time"="", "code"="", "serial"="", "temp"=0.0, "activity"=""} ("data") -> [w2089]
          tunnel: w2076 -> [w2088] mode=indexing
          tunnel: w2075 -> [w2085]
          n867 = Index Array(array=w2088) -> (element #1=w2087:i32, element #2=w2086:i32)  [unwired: 2 in]
          n868 = Bundle By Name(cluster=w2089, "sys"=w2087, "dia"=w2086, "puls"=w2085) -> (w2084:T21)
          n869 = call "AddArmpressureAndSave.vi"("error in"=w2091, "Side(Left/Right)"="", "data"=w2084) -> ("error out"=w2090:errorcluster)  [unwired: 8 in]
        }
      }
      frame "SavePalpationData" {
        n870 = Unbundle By Name(w2107) -> ("User Parameters.CPR Number"=w2103:string, "System Parameters.Date"=w2105:string, "User Parameters.Temp One"=w2095:dbl, "User Parameters.Temp Two"=w2094:dbl, "User Parameters.PalpationRight"=w2093:string, "User Parameters.PalpationLeft"=w2092:string)
        n871 = global read "DataPathGlobalVariable.vi" "DataPath"() -> (w2104:path)
        n872 = call "Encrypt.vi"("Input"=w2103) -> ("Output"=w2102:string)  [unwired: 10 in]
        n873 = Build Array(w2093, w2092) -> (w2098:string[])
        n874 = Build Array(w2095, w2094) -> (w2096:dbl[])
        n875 = Build Path(base path=w2104, name or relative path=w2102) -> (appended path=w2106:path)
        n876 = Number To Decimal String(number=w2096) -> (decimal integer string=w2097:string[])  [unwired: 1 in]
        n877 = Build Path(base path=w2106, name or relative path=w2105) -> (appended path=w2099:path)
        n878 = case shown="No Error" w2100 {
          selector: w2100 -> [w2117 w2119]
          tunnel: w2099 -> [w2118 _]
          tunnel: [w2117 w2119] -> w2101
          tunnel: w2097 -> [w2108 _]
          tunnel: w2098 -> [w2109 _]
          frame No Error {
            n879 = Build Path(base path=w2118, name or relative path="armpressure.dm2000") -> (appended path=w2114:path)
            n880 = call-poly <vilib>:"Read From Spreadsheet File.vi"("delimiter (\\t)"=";" ("delimiter (\\t)"), "file path (dialog if empty)"=w2114) -> ("all rows"=w2113:string[][])  [unwired: 5 in, 4 out]
            n881 = Build Array (concatenate)(w2113, w2108, w2109) -> (w2112:string[][])
            n882 = call-poly <vilib>:"Write To Spreadsheet File.vi"("delimiter (\\t)"=";" ("delimiter (\\t)"), "append to file? (new file:F)"=FALSE, "2D data"=w2112, "file path (dialog if empty)"=w2114) -> ()  [unwired: 4 in, 1 out]
          }
          frame Error {
          }
        }
      }
      frame "SavePatientData" {
        n883 = Unbundle By Name(w2131) -> ("User Parameters.CPR Number"=w2120:string, "User Parameters.Name"=w2130:string, "User Parameters.Operator"=w2129:string, "User Parameters.Doctor"=w2128:string, "User Parameters.Comment"=w2127:string, "cRef.Profile.References.HospitalName"=w2126:refnum<vi>, "cRef.Profile.References.HospitalDepartment"=w2125:refnum<vi>, "cRef.Profile.References.HospitalAddress"=w2124:refnum<vi>)
        n884 = Empty String/Path?(string/path=w2120) -> (empty?=w2121:bool)
        n885 = case shown="False" w2121 {
          tunnel: w2130 -> [w2149 _]
          tunnel: w2129 -> [w2148 _]
          tunnel: w2128 -> [w2147 _]
          tunnel: w2127 -> [w2146 _]
          tunnel: w2126 -> [w2143 _]
          tunnel: w2125 -> [w2142 _]
          tunnel: w2124 -> [w2141 _]
          tunnel: w2123 -> [w2136 w2151]
          tunnel: [w2134 w2151] -> w2122
          tunnel: w2120 -> [w2133 _]
          frame False {
            n886 = call "Encrypt.vi"("Input"=w2133) -> ("Output"=w2132:string)  [unwired: 10 in]
            n887 = Bundle By Name(cluster=T23 {"id"="", "name"="", "operator"="", "doctor"="", "comment"=""} ("profile"), "id"=w2132, "name"=w2149, "operator"=w2148, "doctor"=w2147, "comment"=w2146) -> (w2145:T23)
            n888 = call "SavePatientDateInfo_Profile.vi"("error in"=w2136, "profile"=w2145) -> ("error out"=w2135:errorcluster)  [unwired: 9 in]
            n889 = property class="Str"(reference=w2143) -> ("Value"=w2140:string)  [unwired: 1 in, 2 out]
            n890 = property class="Str"(reference=w2142) -> ("Value"=w2139:string)  [unwired: 1 in, 2 out]
            n891 = property class="Str"(reference=w2141) -> ("Value"=w2138:string)  [unwired: 1 in, 2 out]
            n892 = Bundle By Name(cluster=T22 {"name"="", "department"="", "address"=""} ("hospital"), "name"=w2140, "department"=w2139, "address"=w2138) -> (w2137:T22)
            n893 = call "SavePatientDateInfo_Hospital.vi"("error in"=w2135, "hospital"=w2137) -> ("error out"=w2134:errorcluster)  [unwired: 9 in]
          }
          frame True {
          }
        }
      }
      frame "_SavePatientData" {
        n894 = Unbundle By Name(w2173) -> ("User Parameters.CPR Number"=w2155:string, "User Parameters.Name"=w2172:string, "User Parameters.Operator"=w2171:string, "User Parameters.Doctor"=w2170:string, "User Parameters.Comment"=w2169:string, "cRef.Profile.References.HospitalName"=w2152:refnum<vi>, "cRef.Profile.References.HospitalDepartment"=w2153:refnum<vi>, "cRef.Profile.References.HospitalAddress"=w2154:refnum<vi>)
        n895 = global read "DataPathGlobalVariable.vi" "DataPath"() -> (w2168:path)
        n896 = call "Encrypt.vi"("Input"=w2155) -> ("Output"=w2156:string)  [unwired: 10 in]
        n897 = property class="Str"(reference=w2152) -> ("Value"=w2164:string)  [unwired: 1 in, 2 out]
        n898 = property class="Str"(reference=w2153) -> ("Value"=w2163:string)  [unwired: 1 in, 2 out]
        n899 = property class="Str"(reference=w2154) -> ("Value"=w2165:string)  [unwired: 1 in, 2 out]
        n900 = Build Path(base path=w2168, name or relative path=w2156) -> (appended path=w2166:path)
        n901 = Build Array(w2164, w2163) -> (w2162:string[])
        n902 = call <userlib>:"Multi-line String to Array__ogtk.vi"("string"=w2165) -> ("lines"=w2161:string[])
        n903 = Empty String/Path?(string/path=w2155) -> (empty?=w2160:bool)
        n904 = Build Array (concatenate)(w2162, w2161) -> (w2159:string[])
        n905 = Build Array(w2156, w2172, w2171, w2170, w2169) -> (w2167:string[])
        n906 = case shown="False" w2160 {
          tunnel: w2167 -> [w2182 _]
          tunnel: w2166 -> [w2180 _]
          tunnel: w2159 -> [w2175 _]
          tunnel: w2158 -> [w2174 w2183]
          tunnel: [w2174 w2183] -> w2157
          frame False {
            n907 = Build Array(w2182, w2175) -> (w2181:string[][])
            n908 = Build Path(base path=w2180, name or relative path=T19 "index.dm2000" ("FileName")) -> (appended path=w2177:path)
            n909 = call-poly <vilib>:"Write To Spreadsheet File.vi"("delimiter (\\t)"=";" ("delimiter (\\t)"), "append to file? (new file:F)"=FALSE, "2D data"=w2181, "file path (dialog if empty)"=w2177) -> ()  [unwired: 4 in, 1 out]
          }
          frame True {
          }
        }
      }
      frame "SavePatientDataOnDate" {
        n910 = call "AMC Send Local Message.vi"("Message Name"="SavePatientData", "Message Queue in"=w2185) -> ()  [unwired: 8 in, 2 out]
      }
      frame "GetProcessData" {
        n911 = call "AE Variables.vi"("error in (no error)"=w2194, "Action"=Enum_Variables."Get Red Cursors") -> ("Dbl Array"=w2189:dbl[][], "error out"=w2193:errorcluster)  [unwired: 10 in, 6 out]
        n912 = call "AE Variables.vi"("error in (no error)"=w2193, "Action"=Enum_Variables."Get Blue Cursors") -> ("Dbl Array"=w2188:dbl[][], "error out"=w2192:errorcluster)  [unwired: 10 in, 6 out]
        n913 = call "AE Variables.vi"("error in (no error)"=w2192, "Action"=Enum_Variables."Get Red Pressure") -> ("NumericOut"=w2195:dbl, "error out"=w2197:errorcluster)  [unwired: 10 in, 6 out]
        n914 = call "AE Variables.vi"("error in (no error)"=w2197, "Action"=Enum_Variables."Get Blue Pressure") -> ("NumericOut"=w2196:dbl, "error out"=w2202:errorcluster)  [unwired: 10 in, 6 out]
        n915 = Bundle By Name(cluster=w2201, "Database.Blue Pressure"=w2196, "Database.Red Pressure"=w2195, "Database.BluePositionArray"=w2188, "Database.RedPositionArray"=w2189) -> (w2200:T3)
      }
      frame "SaveProcessData" {
        n916 = Unbundle By Name(w2218) -> ("Database.PatientdataPath"=w2214:path, "Database.Blue Pressure"=w2217:dbl, "Database.Red Pressure"=w2216:dbl, "Database.BluePositionArray"=w2207:dbl[][], "Database.RedPositionArray"=w2211:dbl[][])
        n917 = Matrix Size(0:w2207) -> (1:w2210:i32, 2:w2209:i32)
        n918 = Add(x=w2210, y=w2209) -> (x+y=w2204:i32)
        n919 = Less?(x=w2204, y=6 ("x")) -> (x < y?=w2208:bool)
        n920 = Select(t=dbl[][] [[0.0, 0.0], [0.0, 0.0], [0.0, 0.0], [0.0, 0.0]], s=w2208, f=w2207) -> (s? t:f=w2206:dbl[][])
        n921 = Build Array(w2217, w2216) -> (w2213:dbl[])
        n922 = Build Array (concatenate)(w2213, w2206, w2211) -> (w2212:dbl[][])
        n923 = call-poly <userlib>:"Valid Path__ogtk.vi"("path"=w2214) -> ("valid"=w2215:bool)
        n924 = case shown="True" w2215 {
          tunnel: w2212 -> [_ w2220]
          tunnel: w2214 -> [_ w2222]
          frame False {
          }
          frame True {
            n925 = Build Path(base path=w2222, name or relative path=T19 "processdata.dm2000" ("FileName")) -> (appended path=w2223:path)
            n926 = call-poly <vilib>:"Write To Spreadsheet File.vi"("delimiter (\\t)"=";" ("delimiter (\\t)"), "format (%.3f)"="%s" ("format (%s)"), "append to file? (new file:F)"=FALSE, "2D data"=w2220, "file path (dialog if empty)"=w2223) -> ()  [unwired: 3 in, 1 out]
          }
        }
      }
      frame "DeleteMeasurement" {
        n927 = Unbundle By Name(w2241) -> ("cRef.Data.References.Menu"=w2228:refnum<vi>, "cRef.Data.References.Menu"=w2227:refnum<vi>, "Database.ActiveItemTag"=w2237:string, "cRef.Journal.References.Data"=w2231:refnum<vi>)
        n928 = property class="MCListbox (strict)"(reference=w2231, error in=w2238) -> (reference out=w2239:refnum<vi>, error out=w2233:errorcluster, "ItemNames"=w2242:string[][], "Value"=w2230:i32)
        n929 = String To Path(string=w2237) -> (path=w2240:path)
        n930 = Index Array(array=w2242, index (row)=w2230, index (col)=0 ("disabled index (col)")) -> (element=w2229:string)
        n931 = Build Path(base path=w2240, name or relative path=w2229) -> (appended path=w2235:path)
        n932 = call <vilib>:"Check if File or Folder Exists.vi"("error in (no error)"=w2233, "path"=w2235) -> ("error out"=w2232:errorcluster, "file or folder exists?"=w2234:bool)  [unwired: 7 in, 1 out]
        n933 = case shown="True" w2234 {
          tunnel: w2235 -> [_ w2258]
          tunnel: w2239 -> [_ w2255]
          tunnel: w2237 -> [_ w2247]
          tunnel: [w2244 w2252] -> w2236
          tunnel: w2232 -> [w2244 w2249]
          tunnel: w2228 -> [_ w2246]
          tunnel: w2227 -> [_ w2245]
          frame False {
          }
          frame True {
            n934 = Delete(path (use dialog)=w2258, entire hierarchy (F)=TRUE, confirm (F)=TRUE, error in=w2249) -> (deleted path=w2251:path, cancelled=w2250:bool, error out=w2254:errorcluster)  [unwired: 1 in]
            n935 = String To Path(string=w2247) -> (path=w2248:path)
            n936 = call "ListboxItems (SubVI).vi"("error in (no error)"=w2254, "MCListbox Refnum"=w2255, "path"=w2248) -> ("error out"=w2253:errorcluster)  [unwired: 2 in]
            n937 = case shown="False" w2250 {
              tunnel: w2253 -> [w2263 w2273]
              tunnel: [w2262 w2272] -> w2252
              tunnel: w2251 -> [w2264 _]
              tunnel: w2246 -> [w2260 _]
              tunnel: w2245 -> [w2259 _]
              frame False {
                n938 = Build Array(w2260, w2259) -> (w2261:refnum<vi>[])
                n939 = Path To String(path=w2264) -> (string=w2265:string)
                n940 = for {
                  tunnel: w2261 -> [w2267] mode=indexing
                  tunnel: TRUE ("Delete Children?") -> [w2271]
                  tunnel: w2265 -> [w2270]
                  tunnel: w2263 -> [w2269]
                  tunnel: [w2268] -> w2262
                  n941 = invoke class="Tree (strict)" method="Edit Tree Items.Delete"(reference=w2267, error in=w2269, "tag"=w2270, "Delete Children"=w2271) -> (error out=w2268:errorcluster)  [unwired: 1 in, 4 out]
                }
              }
              frame True {
                n942 = call <vilib>:"Clear Errors.vi"("error in (no error)"=w2273) -> ("error out"=w2272:errorcluster)  [unwired: 6 in]
              }
            }
          }
        }
      }
      frame "/*********Shutdown********/" {
      }
      frame "Error" {
        n943 = call <vilib>:"General Error Handler CORE.vi"("type of dialog (OK msg:1)"=DialogTypeEnum."auto error handling dialog", "error in (no error)"=w2283) -> ("stop event propagated"=w2280:bool, "error out"=w2276:errorcluster)  [unwired: 12 out]
        n944 = case "User Chose to Stop and Not Continue\nFALSE = Continue: CLEAR ERRORS" shown="True" w2280 {
          tunnel: [w2284 w2288] -> w2282
          tunnel: w2276 -> [w2285 w2293]
          tunnel: w2281 -> [_ w2292]
          tunnel: w2278 -> [w2286 w2295]
          tunnel: [w2286 w2294] -> w2277
          frame False {
            n945 = call <vilib>:"Clear Errors.vi"("error in (no error)"=w2285) -> ("error out"=w2284:errorcluster)  [unwired: 6 out]
          }
          frame True {
            n946 = call <vilib>:"Clear Errors.vi"("error in (no error)"=w2293) -> ("error out"=w2291:errorcluster)  [unwired: 6 out]
            n947 = Bundle By Name(cluster=w2295, "Terminate Error"=w2293) -> (w2294:T3)
            n948 = call "AMC Flush Message Queue.vi"("error in (no error)"=w2291, "Message Queue in"=w2292) -> ("error out"=w2290:errorcluster, "Message Queue out"=w2289:T6)  [unwired: 7 in]
            n949 = call "AMC Send Local Messages.vi"("error in (no error)"=w2290, "Message Names"=string[] ["Close SubVI", "Exit"], "Message Queue in"=w2289) -> ("error out"=w2288:errorcluster)  [unwired: 7 in, 1 out]
          }
        }
      }
      frame "Exit" {
        w2296 = refnum<class> refnum  # event data
        # "Don't wire 'Error In'\nMust Execute Regardless"
        n950 = Unbundle By Name(w2302) -> ("Exit Event"=w2301:T4, "Terminate Error"=w2298:errorcluster)
        n951 = Generate User Event(user event=w2301, event data cluster=w2296) -> (error out=w2300:errorcluster)  [unwired: 2 in, 1 out]
        n952 = Merge Errors(w2300, w2298, w2297) -> (w2299:errorcluster)
      }
      frame "Close SubVI" {
      }
      frame Default {
        w2308 = 1 items=["No error", "Argument error", "Memory is full", "Out of zone", "End of file", "File already open", "Generic file I/O error", "File not found", "File permission error", "Disk is full", "Duplicate path", "Too many files open", "System feature not enabled", "Resource file not found", "Cannot add resource", "Resource not found", "Image not found", "Image memory error", "Pen does not exist", "Config type invalid", "Config token not found", "Config parse error", "Config memory error", "Bad external code format", "Bad external code offset", "External code not present", "Null window", "Destroy window error", "Null menu", "Print aborted", "Bad print record", "Print driver error", "Windows error during printing", "Memory error during printing", "Print dialog error", "Generic print error", "Invalid device refnum", "Device not found", "Device parameter error", "Device unit error", "Cannot open device", "Device call aborted", "Generic error", "Cancelled by user", "Object ID too low", "Object ID too high", "Object not in heap", "Unknown heap", "Unknown object (invalid DefProc)", "Unknown object (DefProc not in table)", "Message out of range", "Invalid (null) method", "Unknown message", "Manager call not supported", "Bad address", "Network operation in progress", "Network operation timed out", "Connection is busy", "Network attribute not supported", "Network error", "Address in use", "System out of memory", "Connection aborted", "Connection refused", "Not connected", "Already connected", "Connection closed", "Initialization error (interapplication manager)", "Bad occurrence", "Wait on unbound occurrence handler", "Occurrence queue overflow", "Datalog type conflict", "Unused", "Unrecognized type (interapplication manager)", "Memory corrupt", "Failed to make temporary DLL", "Old CIN version", "Drag socket not found", "Failed to load drop-object", "Failed to register OLE object", "Failed to release OLE object", "Format specifier type mismatch", "Unknown format specifier", "Too few format specifiers", "Too many format specifiers", "Scan failed", "Newer CIN version", "Error converting to variant", "Runtime menu error", "Password tampered", "Variant attribute not found", "Incompatible variant data type", "Event data is not available", "Event Store is not present", "Occurrence is not found", "Event Queue is not created", "Event info is not available", "Refnum passed is NULL", "Error retrieving Class GUID", "Error retrieving CoClass GUID", "Error retrieving TypeLib GUID.", "Bad built application magic bytes.", "Specific driver is different from the specific driver associated with the Logical Name.", "There is no session opened to the class driver.", "Max Error", "MAX - Error with config objects", "MAX - Error loading configuration", "MAX - Group not supported"]
        w2309 = TRUE  # status
        n953 = Format Into String(format string="DEVELOPER ERROR:\nImproper State Requested\n================\nState {%s} does not exist within this architecture\n\nCheck for spelling and case errors" ("source"), w2306) -> (resulting string=w2307:string)  [unwired: 2 in, 1 out]
        n954 = Bundle By Name(cluster=w2311, "status"=w2309, "code"=w2308, "source"=w2307) -> (w2310:errorcluster)
      }
    }
    n955 = Get Date/Time In Seconds() -> (seconds since 1Jan1904=w361:timestamp)
    n956 = Get Date/Time String(seconds (now)=w361, want seconds? (F)=TRUE) -> (time string=w359:string)  [unwired: 1 in, 1 out]
    n957 = Concatenate Strings(w359, w360) -> (w358:string)
  }
  n958 = control-ref of="This VI"() -> (w2:refnum<vi>)
  n959 = call "Save Log.vi"("Array"=w1, "VI in"=w2) -> ()  [unwired: 10 in]
  n960 = while "App Close" {
    shift-right: [w2319] -> _
    shift-left: enum16{"Close Display", "Clear References"}."Close Display" -> [w2318]
    tunnel: w15 -> [w2316]
    tunnel: w17 -> [w2317]
    tunnel: [w2314] -> w11
    shift-right: [w2313] -> w10
    shift-left: w16 -> [w2315]
    i -> [w2320]
    stop <- w2321 stop-if-true
    n961 = case shown="\"Clear References\"" w2318 {
      tunnel: [w2322 w2329] -> w2314
      tunnel: [w2324 w2328] -> w2313
      tunnel: [w2323 _] -> _
      tunnel: w2317 -> [w2322 w2329]
      tunnel: w2316 -> [w2323 w2330]
      tunnel: w2315 -> [w2324 w2328]
      frame "Close Display" {
        n962 = disable-structure shown="RUN_TIME_ENGINE==True" {
          frame condition #0 (active) {
          }
          frame condition #1 {
            n963 = control-ref of="This VI"() -> (w2325:refnum<vi>)
            n964 = invoke class="VI" method="FP.Open"(reference=w2325, "Activate"=TRUE ("Activate?"), "State"=T2."Standard") -> ()  [unwired: 2 in, 5 out]
          }
        }
      }
      frame "Clear References" {
        n965 = Unbundle By Name(w2328) -> ("Exit Event"=w2331:T4)
        n966 = call "Close SubVI.vi"("SHIFTER DATA"=w2328) -> ()  [unwired: 11 in]
        n967 = Unregister For Events(event registration refnum=w2330) -> ()  [unwired: 1 in, 1 out]
        n968 = Destroy User Event(user event=w2331) -> ()  [unwired: 1 in, 1 out]
      }
    }
    n969 = call "Enum Loop Complete.vi"("Current State Enum"=w2318, "Itteration"=w2320) -> ("Loop Complete?"=w2321:bool)  [unwired: 13 out]
    n970 = Increment(x=w2318) -> (x+1=w2319:enum16{"Close Display", "Clear References"})
  }
  n971 = disable-structure shown="RUN_TIME_ENGINE==True" {
    disable-tunnel: [w2332 w2333] -> w9
    disable-tunnel: w11 -> [w2332 w2333]
    frame condition #0 (active) {
    }
    frame condition #1 {
      n972 = Quit LabVIEW() -> ()  [unwired: 1 in]
    }
  }
  n973 = Unbundle By Name(w10) -> ("Terminate Error"=w8:errorcluster)
  n974 = Merge Errors(w8, w9) -> (w4:errorcluster)
  n975 = call <vilib>:"Clear Errors.vi"("error in (no error)"=w4) -> ()  [unwired: 6 in, 1 out]
